vi "PDC.vi"() -> ()   [LabVIEW 2013]
uses:
  CTRLs/PMU_CMDs.ctl
panel:
  in  "data array [mag, phase (deg)]":cluster{"magnitude":dbl, "phase":dbl}[](array[cluster])=[{"magnitude"=10.0, "phase"=0.0}, {"magnitude"=10.0, "phase"=0.0}, {"magnitude"=10.0, "phase"=0.0}, {"magnitude"=10.0, "phase"=0.0}, {"magnitude"=10.0, "phase"=0.0}, {"magnitude"=10.0, "phase"=0.0}, {"magnitude"=10.0, "phase"=0.0}, {"magnitude"=10.0, "phase"=0.0}, {"magnitude"=10.0, "phase"=0.0}, {"magnitude"=10.0, "phase"=0.0}, {"magnitude"=10.0, "phase"=0.0}, {"magnitude"=10.0, "phase"=0.0}, {"magnitude"=10.0, "phase"=0.0}, {"magnitude"=10.0, "phase"=0.0}, {"magnitude"=10.0, "phase"=0.0}, {"magnitude"=10.0, "phase"=0.0}, {"magnitude"=10.0, "phase"=0.0}, {"magnitude"=10.0, "phase"=0.0}, {"magnitude"=10.0, "phase"=0.0}] {"phase" format="%0.2f"; "magnitude" format="%0.2f"}
  in  "Size":u16=4
  out "Freq":sgl[](array[numeric])
  out "path":path
  out "T button?":bool
  out "PMU1 CFG Packet":string[](array[string])
  out "PMU Row Number":i32
  out "UDP STRNG 2":string
  out "Date/Time 4":string
  out "Phasor Row Number":i32
  in  "Tab Control 2":T1(tab)
  out "MagnitudePMU":waveform(sgl)(graph)
  out "FrequencyPMU":waveform(sgl)(graph)
  out "PMUROCOF":waveform(sgl)(graph)
  out "PMUAnalogs":waveform(sgl)(graph)
  out "seconds":dbl
  out "Array 2":u16[][](array[numeric]) format="%b"
  out "Array":string[][](array[string])
  out "Analogs":string[][](array[string])
  out "Freq Floating?":bool[](array[boolean])
  out "Analog Floating?":bool[](array[boolean])
  out "Polar?":bool[](array[boolean])
  out "Transposed":string[][](array[string])
  out "Real":string[][](array[string])
  out "Imaginary":string[][](array[string])
  out "transposed array 5":sgl[][](array[numeric])
  out "transposed array 4":sgl[][](array[numeric])
  out "Phasors Floatingpoint?":bool[](array[boolean])
  out "Format":u16[](array[numeric]) format="%b"
  out "Digitals":u16[](array[numeric])
  out "Analog":u16[](array[numeric])
  out "Phasor":u16[](array[numeric])
  out "DGTL Packet":string[](array[string])
  out "ANG Packet":string[](array[string])
  out "DFREQ Packet":string[](array[string])
  out "FREQ Packet":string[](array[string])
  out "PZRs Packet":string[](array[string])
  out "UNITs 2":T2
  out "Date/Time 3":string
  out "PMU DATA Packet 2":string[](array[string])
  out "DATA FRAME 2":string
  out "error out 2":errorcluster
  out "UDP STRNG":string
  out "UNITs":T2
  out "Date/Time 2":string
  in  "Start Com Button":bool
  in  "User Configuration":T3(tab)
  in  "IP Address":string="127.0.0.1"
  in  "remote port":u16=4712
  in  "Device ID":u16
  in  "Unicast Address":string="127.0.0.1"
  in  "Local Port":u16=58431
  in  "TTL":u16=16
  in  "Send to Port":u16=58432
  out "Alert Incorrect \nNetwork Info":bool
  in  "Data Display":T4(tab)
  in  "PMU Phasors":i32(listbox)
  in  "PMU Analogs":i32(listbox)
  in  "PMU Digitals":i32(listbox)
  in  "dFreq":sgl[](array[numeric])
  in  "Frequency":sgl[](array[numeric])
  in  "Tab Control":T5(tab)
  in  "Complex Phasors":csg[][](array[numeric])
  in  "Magnitude":sgl[][](array[numeric])
  in  "Angle (Radians)":sgl[][](array[numeric])
  in  "Analog Values":sgl[][](array[numeric])
  out "Boolean array":bool[][](array[boolean])
  out "Magnitude":sgl[](array[numeric])
  out "Angle":sgl[](array[numeric])
  out "Complex Phasors":csg[](array[numeric])
  out "DFREQ Values":dbl[](array[numeric])
  out "FREQ Values":dbl[](array[numeric])
  out "Chosen Data 2":i32(listbox)
  out "DATA ONLINE":bool
  in  "Display Cluster Output":bool
  out "UDP String":string
  out "Freq >Threshold":bool
  out "Frequency Monitoring":waveform(sgl)[](graph)
  out "Freq < Threshold":bool
  out "Warning":string[](array[string])
  out "Phasor Plot":picture
  out "Available Phasors in the PMU/PDC Stream":string[](array[string])
  out "Phasor Magnitude":sgl[](array[numeric])
  out "Phasor Angle (Degrees)":sgl[](array[numeric])
  in  "Data Selector":T6(tab)
  out "No. of Digitals in this PMU":u8
  out "No. of Analogs in this PMU":u8
  out "No. of Phasors in this PMU":u8
  out "Freq/dFreq Format":string
  out "Analog Format":string
  out "Phasor Format":string
  out "Phasor Type":string
  out "DATA_RATE":u32
  in  "Names of PMUs":i32(listbox)
  out "Nominal_Frequency":string
  out "NUM_of_PMUs":u32
  in  "PMU Phasors List 2":i32(listbox)
  out "Phasor_Names":string[](array[string])
  in  "PMU Phasors List":i32(listbox)
  out "Phasors Index":u16[](array[numeric])
  out "PMU number in List":i32[](array[numeric])
  out "Phasor number in selected PMU":i32[](array[numeric])
  out "Time Quality":string[](array[string])
  out "STAT FIELD  WITH RESPEC TO PMU List":string[](array[string])
  out "PMUs List":i32(listbox)
  out "GPS Sync?":bool[](array[boolean])
  out "Status - PMU Sync with GPS":string[](array[string])
  out "Unlocked Time":string[](array[string])
  out "Config Change?":bool[](array[boolean])
  out "Change in Configuration":string[](array[string])
  out "PMUs List 2":i32(listbox)
  out "PMU DATA Packet":string[](array[string])
  out "Data size to read":u32
  out "Size of DATA Frame":u32
  out "CFG-2 Frame":string
  out "PMU1 CFG Packet":string[](array[string])
  out "Date/Time":string
  out "TIME_BASE":u32
  out "FRACSEC":u64
  out "SOC":u64
  out "IDCODE":u32
  out "FRAMSIZE":u32
  out "SYNC":u32
  out "Valid?!":bool
  out "CRC-Bytes":string
  out "DATA FRAME":string
  in  "Stop Button":bool
  out "COMMAND Frame":string
  out "bytes written":i32
  in  "DATA ON":bool
  in  "DATA OFF":bool
  out "length":i32
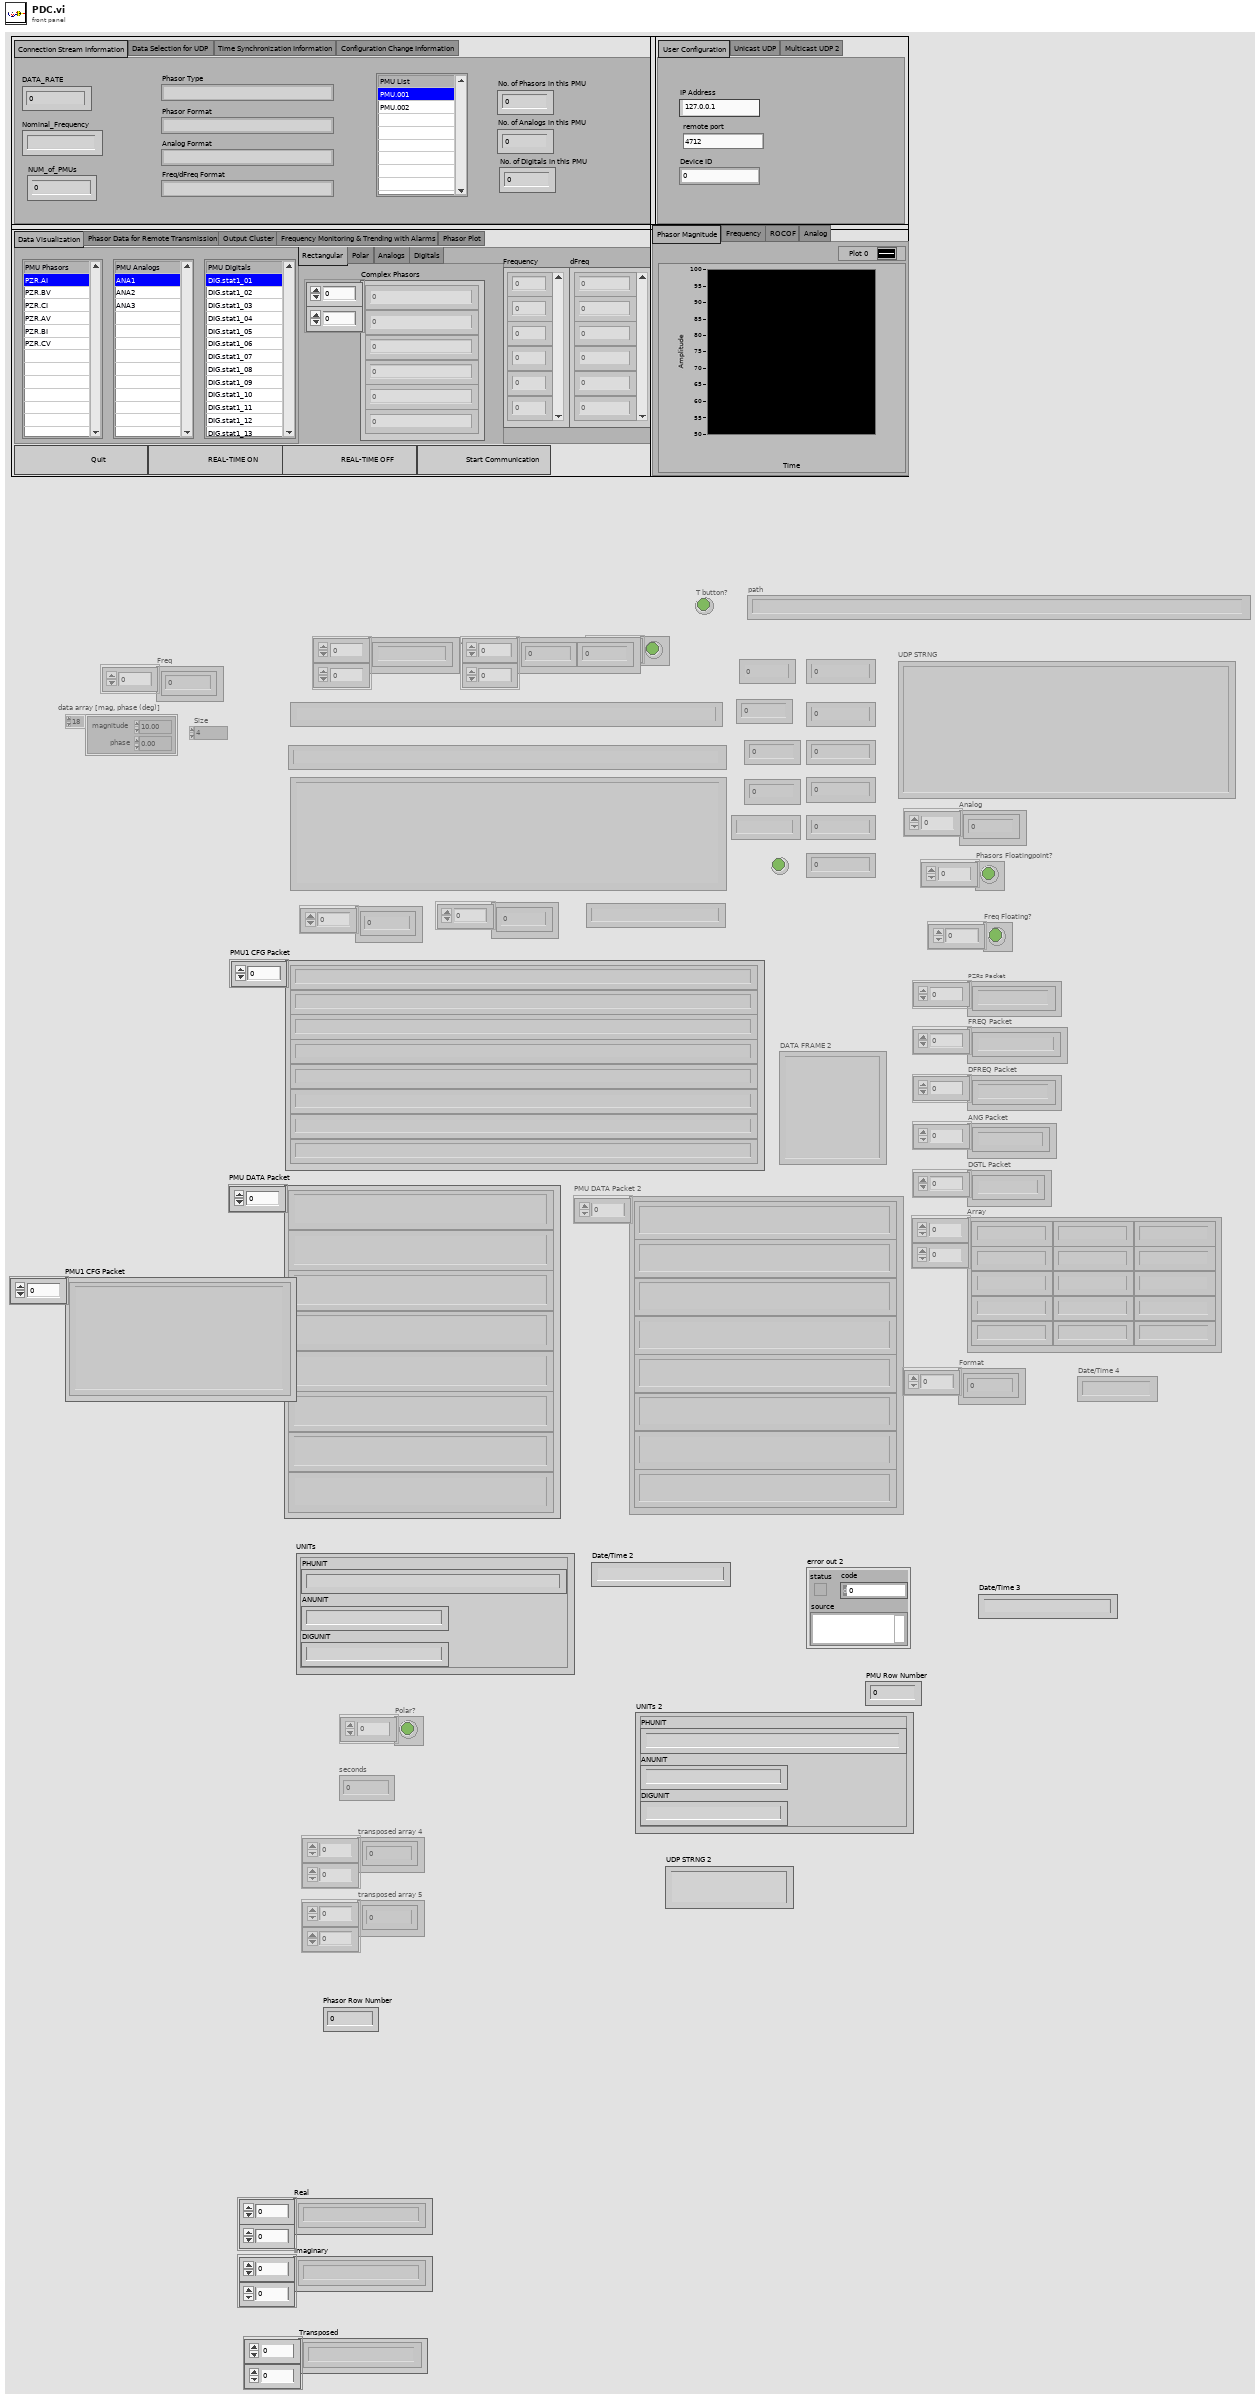
[diagram p1: front panel]
types:
  T1 = enum32{"Phasor Magnitude", "Frequency", "ROCOF", "Analog"}
  T2 = cluster{"PHUNIT":string, "ANUNIT":string, "DIGUNIT":string}
  T3 = enum32{"User Configuration", "Unicast UDP", "Multicast UDP 2"}
  T4 = enum32{"Data Visualization", "Phasor Data for Remote Transmission", "Output Cluster", "Frequency Monitoring & Trending with Alarms", "Phasor Plot"}
  T5 = enum32{"Rectangular", "Polar", "Analogs", "Digitals"}
  T6 = enum32{"Connection Stream Information", "Data Selection for UDP", "Time Synchronization Information", "Configuration Change Information"}
  T7 = cluster{"Date/Time":string, "DATA_DTLD":cluster{"PZRs Packet":string[], "FREQ Packet":string[], "DFREQ Packet":string[], "ANG Packet":string[], "DGTL Packet":string[]}}
  T8 = typedef "PMU_CMDs.ctl" = enum16{"dummy", "Turn off Transmission of Data Frame", "Turn on Transmission of Data Frame", "Send Header Frame", "Send CFG-1 Frame", "Send CFG-2 Frame", "Extended Frame"}
  T9 = cluster{"SYNC":u32, "FRAMSIZE":u32, "IDCODE":u32, "SOC":u64, "DATA_RATE":u32, "FRACSEC":u64, "TIME_BASE":u32, "NUM_PMU":u32}
  T10 = cluster{"PHASORS":cluster{"PZR 1":string, "PZR 2":string, "PZR 3":string, "PZR 4":string, "PZR 5":string, "PZR 6":string}, "NUMs":cluster{"PHNMR":u8, "ANNMR":u8, "DGNMR":u8}, "FORMAT":cluster{"PH_MAG_ANG":u16, "PH_FLOATING":u16, "AN_FLOATING":u16, "FREQ_DFREQ_FLOATING":u16}, "ANGs":cluster{"AN1":string, "AN2":string, "AN3":string}, "DIGs":cluster{"DIG 1":string, "DIG 2":string, "DIG 3":string, "DIG 4":string, "DIG 5":string, "DIG 6":string, "DIG 7":string, "DIG 8":string, "DIG 9":string, "DIG 10":string, "DIG 11":string, "DIG 12":string, "DIG 13":string, "DIG 14":string, "DIG 15":string, "DIG 16":string}, "IDCODE":u16, "Station Name":string, "UNITs":cluster{"PHUNIT":string, "ANUNIT":string, "DIGUNIT":string}, "FNOM":string, "CFGCNT":string}
  T11 = cluster{"PZRs Packet":string[], "FREQ Packet":string[], "DFREQ Packet":string[], "ANG Packet":string[], "DGTL Packet":string[]}
  T12 = typedef "LVDateTimeRec.ctl" = cluster{"fractional second":dbl, "second":i32, "minute":i32, "hour":i32, "day of month":i32, "month":i32, "year":i32, "day of week":i32, "day of year":i32, "DST":i32}
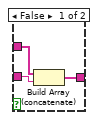
[diagram p4: hidden frame]
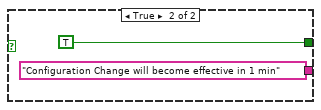
[diagram p5: hidden frame]
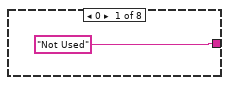
[diagram p6: hidden frame]
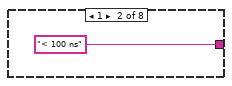
[diagram p7: hidden frame]
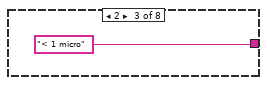
[diagram p8: hidden frame]
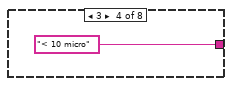
[diagram p9: hidden frame]
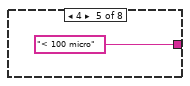
[diagram p10: hidden frame]
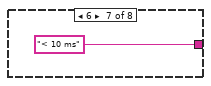
[diagram p11: hidden frame]
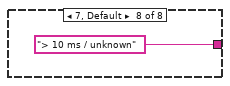
[diagram p12: hidden frame]
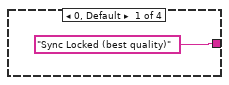
[diagram p13: hidden frame]
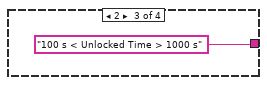
[diagram p14: hidden frame]
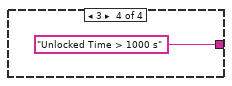
[diagram p15: hidden frame]
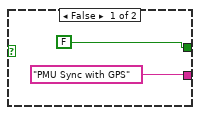
[diagram p16: hidden frame]
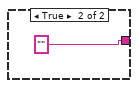
[diagram p17: hidden frame]
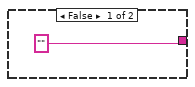
[diagram p18: hidden frame]
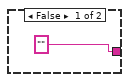
[diagram p19: hidden frame]
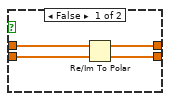
[diagram p20: hidden frame]
diagram:
  # "This file is part of BFE.\n\n    BFE is free software: you can redistribute it and/or modify\n    it under the terms of the GNU General Public License as published by\n    the Free Software Foundation, either version 3 of the License, or\n    (at your option) any later version.\n\n   BFE is distributed in the hope that it will be useful,\n    but WITHOUT ANY WARRANTY; without even the implied warranty of\n    MERCHANTABILITY or FITNESS FOR A PARTICULAR PURPOSE.  See the\n    GNU General Public License for more details.\n\n    You should have received a copy of the GNU General Public License\n    along with BFE.  If not, see <http://www.gnu.org/licenses/>."
  n1 = flat-sequence {
    tunnel: [w84] -> w64
    tunnel: [w83] -> w62
    frame #0 {
      w74 = "" ("Phasor Type")
      w73 = u8 0 ("No. of Phasors in this PMU")
      w72 = string[] [""] ("Phasor Name")
      # "License Prompt"
      # "Initializing all variables to their default values"
      n2 = Two Button Dialog(message="<BFE>  Copyright (C) <2016>  <Luigi Vanfretti, Muhammad Shoaib Almas, Maxime Baudette>\n    This program comes with ABSOLUTELY NO WARRANTY; for details click on \"show details\"'.\n    This is free software, and you are welcome to redistribute it\n    under certain conditions; click on `show details' for details.", 1:"Show Details" ("F button name (\"Cancel\")"), 2:"OK" ("T button name (\"OK\")")) -> (T button?=w67:bool)
      "T button?" <- w67
      n3 = Equal?(x=w67, y=FALSE) -> (x = y?=w65:bool)
      n4 = case shown="True" w65 {
        frame False {
        }
        frame True {
          n5 = Current VI's Path() -> (path=w79:path)
          "path" <- w79
          n6 = Strip Path(path=w79) -> (stripped path=w77:path)  [unwired: 1 out]
          n7 = Build Path(base path=w77, name or relative path="License") -> (appended path=w75:path)
          n8 = call <vilib>:"System Exec.vi"("working directory"=w75, "command line"="Notepad COPYING") -> ()  [unwired: 6 in, 4 out]
        }
      }
      n9 = property on="NUM_of_PMUs" class="DigNum (strict)"("Value"=w73) -> ()  [unwired: 2 in, 2 out]
      n10 = property on="DATA_RATE" class="DigNum (strict)"("Value"=w73) -> ()  [unwired: 2 in, 2 out]
      n11 = property on="No. of Phasors in this PMU" class="DigNum (strict)"("Value"=w73) -> ()  [unwired: 2 in, 2 out]
      n12 = property on="No. of Analogs in this PMU" class="DigNum (strict)"("Value"=w73) -> ()  [unwired: 2 in, 2 out]
      n13 = property on="No. of Digitals in this PMU" class="DigNum (strict)"("Value"=w73) -> ()  [unwired: 2 in, 2 out]
      n14 = property on="Analog Format" class="Str"("Value"=w74) -> ()  [unwired: 2 in, 2 out]
      n15 = property on="Phasor Type" class="Str"("Value"=w74) -> ()  [unwired: 2 in, 2 out]
      n16 = property on="Phasor Format" class="Str"("Value"=w74) -> ()  [unwired: 2 in, 2 out]
      n17 = property on="Freq/dFreq Format" class="Str"("Value"=w74) -> ()  [unwired: 2 in, 2 out]
      n18 = property on="Phasors Index" class="Arr (strict)"("Value"=u16[] [0, 0, 0, 0] ("Phasors Index")) -> ()  [unwired: 2 in, 2 out]
      n19 = property on="Nominal_Frequency" class="Str"("Value"=w74) -> ()  [unwired: 2 in, 2 out]
      n20 = property on="PMU Phasors List" class="LstBox (strict)"("Item Names"=w72) -> ()  [unwired: 2 in, 2 out]
      n21 = property on="PMU Analogs" class="LstBox (strict)"("Item Names"=w72) -> ()  [unwired: 2 in, 2 out]
      n22 = property on="PMU Phasors" class="LstBox (strict)"("Item Names"=w72) -> ()  [unwired: 2 in, 2 out]
      n23 = property on="PMU Digitals" class="LstBox (strict)"("Item Names"=w72) -> ()  [unwired: 2 in, 2 out]
      n24 = property on="Names of PMUs" class="LstBox (strict)"("Item Names"=w72) -> ()  [unwired: 2 in, 2 out]
      n25 = property on="Names of PMUs" class="LstBox (strict)"("Item Names"=w72) -> ()  [unwired: 2 in, 2 out]
      n26 = property on="Phasor_Names" class="Arr (strict)"("Value"=w72) -> ()  [unwired: 2 in, 2 out]
    }
    frame #1 {
      n27 = while {
        stop <- "Start Com Button" stop-if-true
      }
    }
    frame #2 {
      n28 = TCP Open Connection(address="IP Address", remote port or service name="remote port") -> (connection ID=w84:refnum<k5>, error out=w83:errorcluster)  [unwired: 3 in]
    }
  }
  n29 = flat-sequence {
    tunnel: w64 -> [w90]
    tunnel: w62 -> [w91]
    tunnel: [w89] -> w50
    tunnel: [w88] -> w49
    tunnel: ["Device ID"] -> w24
    tunnel: w50 -> [w95]
    tunnel: [w98] -> w48
    tunnel: w49 -> [w96]
    tunnel: [w97] -> w46
    tunnel: w24 -> [w92]
    tunnel: [w92] -> w23
    tunnel: w48 -> [w107]
    tunnel: [w108] -> w47
    tunnel: w46 -> [w106]
    tunnel: [w109] -> w45
    tunnel: [w100] -> w44
    tunnel: w23 -> [w99]
    tunnel: [w99] -> w22
    tunnel: w47 -> [w114]
    tunnel: [w114] -> w52
    tunnel: w45 -> [w113]
    tunnel: [w113] -> w51
    tunnel: w44 -> [w111]
    tunnel: [w111] -> w43
    tunnel: w22 -> [w110]
    tunnel: [w110] -> w21
    tunnel: w52 -> [w120]
    tunnel: [w119] -> w41
    tunnel: w51 -> [w118]
    tunnel: [w117] -> w40
    tunnel: w43 -> [w122]
    tunnel: [w122] -> w39
    tunnel: w21 -> [w115]
    tunnel: [w115] -> w20
    tunnel: w41 -> [w127]
    tunnel: w40 -> [w126]
    tunnel: [w129] -> w60
    tunnel: [w128] -> w59
    tunnel: w39 -> [w124]
    tunnel: [w124] -> w42
    tunnel: w20 -> [w123]
    tunnel: w60 -> [w141]
    tunnel: w59 -> [w140]
    tunnel: [w143] -> w58
    tunnel: [w142] -> w57
    tunnel: [w131] -> w56
    tunnel: w42 -> [w139]
    tunnel: w58 -> [w158]
    tunnel: w57 -> [w157]
    tunnel: w56 -> [w149]
    tunnel: [w158] -> w55
    tunnel: [w157] -> w54
    tunnel: [w149] -> w53
    tunnel: [w144] -> w38
    tunnel: w55 -> [w197]
    tunnel: w54 -> [w196]
    tunnel: w53 -> [w195]
    tunnel: w38 -> [w176]
    tunnel: [w197] -> w33
    tunnel: [w196] -> w32
    tunnel: [w172] -> w31
    tunnel: w33 -> [w218]
    tunnel: w32 -> [w217]
    tunnel: w31 -> [w216]
    tunnel: [w218] -> w28
    tunnel: [w217] -> w27
    tunnel: [w216] -> w26
    tunnel: [w230] -> w30
    tunnel: [w227] -> w61
    tunnel: [w225] -> w63
    tunnel: w28 -> [w226]
    tunnel: w27 -> [w228]
    tunnel: w26 -> [w230]
    frame #0 {
      n30 = call "CMD.vi"("PMU ID"="Device ID", "command"=PMU_CMDs."Turn off Transmission of Data Frame") -> ("CMD"=w87:string)  [unwired: 4 in, 1 out]
      n31 = TCP Write(connection ID=w90, data in=w87, error in (no error)=w91) -> (connection ID out=w89:refnum<k5>, error out=w88:errorcluster)  [unwired: 1 in, 1 out]
    }
    frame #1 {
      n32 = call "CMD.vi"("PMU ID"=w92, "command"=PMU_CMDs."Send CFG-2 Frame") -> ("CMD"=w93:string)  [unwired: 4 in, 1 out]
      n33 = TCP Write(connection ID=w95, data in=w93, error in (no error)=w96) -> (connection ID out=w98:refnum<k5>, error out=w97:errorcluster)  [unwired: 1 in, 1 out]
    }
    frame #2 {
      w103 = 2 ("offset (0)")
      n34 = TCP Read(connection ID=w107, bytes to read=4, error in (no error)=w106) -> (connection ID out=w108:refnum<k5>, data out=w104:string, error out=w109:errorcluster)  [unwired: 2 in]
      n35 = String Subset(string=w104, offset (0)=w103, length (rest)=w103) -> (substring=w102:string)
      n36 = Type Cast(type=u16 0 ("bytes to read"), x=w102) -> (*(type *) &x=w100:u16)
    }
    frame #3 {
      n37 = Wait (ms)(milliseconds to wait=u32 20) -> ()  [unwired: 1 out]
    }
    frame #4 {
      n38 = call "CMD.vi"("PMU ID"=w115, "command"=PMU_CMDs."Turn off Transmission of Data Frame") -> ("CMD"=w121:string)  [unwired: 4 in, 1 out]
      n39 = TCP Write(connection ID=w120, data in=w121, error in (no error)=w118) -> (connection ID out=w119:refnum<k5>, error out=w117:errorcluster)  [unwired: 1 in, 1 out]
    }
    frame #5 {
      n40 = call "CMD.vi"("PMU ID"=w123, "command"=PMU_CMDs."Send CFG-2 Frame") -> ("CMD"=w125:string)  [unwired: 4 in, 1 out]
      n41 = TCP Write(connection ID=w127, data in=w125, error in (no error)=w126) -> (connection ID out=w129:refnum<k5>, error out=w128:errorcluster)  [unwired: 1 in, 1 out]
    }
    frame #6 {
      w137 = 4 ("y")
      n42 = TCP Read(connection ID=w141, bytes to read=w139, error in (no error)=w140) -> (connection ID out=w143:refnum<k5>, data out=w132:string, error out=w142:errorcluster)  [unwired: 2 in]
      n43 = String Length(string=w132) -> (length=w138:i32)
      n44 = Subtract(x=w138, y=w137) -> (x-y=w133:i32)
      n45 = String Subset(string=w132, offset (0)=w133, length (rest)=w137) -> (substring=w136:string)
      n46 = String Subset(string=w132, offset (0)=0, length (rest)=w133) -> (substring=w135:string)
      n47 = Concatenate Strings(w136, w135) -> (w131:string)
      "CFG-2 Frame" <- w131
    }
    frame #7 {
      n48 = call "CHK_CRC.vi"("data in"=w149) -> ("Valid?!"=→"Valid?!":bool, "CRC-Bytes"=→"CRC-Bytes":string)
      n49 = call "SYS_INFO.vi"("CFG-2"=w149) -> ("output cluster"=w150:T9)
      n50 = Unbundle By Name(w150) -> ("SYNC"=→"SYNC":u32, "FRAMSIZE"=→"FRAMSIZE":u32, "IDCODE"=→"IDCODE":u32, "SOC"=w148:u64, "FRACSEC"=w146:u64, "TIME_BASE"=w145:u32, "NUM_PMU"=w144:u32, "DATA_RATE"=→"DATA_RATE":u32)
      "SOC" <- w148
      "FRACSEC" <- w146
      "TIME_BASE" <- w145
      "NUM_of_PMUs" <- w144
      n51 = call "UNIX-DATE_TIME.vi"("TIME_BASE"=w145, "FRACSEC"=w146, "SOC"=w148) -> ("Date/Time"=→"Date/Time":string)  [unwired: 1 out]
    }
    frame #8 {
      w192 = 4
      w174 = 2
      n52 = call "PMU_CFG-2_PACK.vi"("String"=w195) -> ("PMU1 CFG Packet"=w172:string[])
      "PMU1 CFG Packet" <- w172
      n53 = Index Array(array=w172, index=0) -> (element=w194:string)
      n54 = call "PMU_INFO.vi"("data in"=w194) -> ("RET_DATA"=w162:T10)
      n55 = Unbundle By Name(w162) -> ("FNOM"=w161:string)
      n56 = Type Cast(type=u16 2 ("length (rest)"), x=w161) -> (*(type *) &x=w160:u16)
      n57 = Unbundle By Name(w162) -> ("FORMAT.PH_MAG_ANG"=w168:u16, "FORMAT.PH_FLOATING"=w167:u16, "FORMAT.AN_FLOATING"=w166:u16, "FORMAT.FREQ_DFREQ_FLOATING"=w165:u16)
      n58 = case shown="1" w160 {
        tunnel: ["60 Hz Nominal" "50 Hz"] -> w159
        frame 0, Default {
        }
        frame 1 {
        }
      }
      "Nominal_Frequency" <- w159
      n59 = case shown="0, Default" w168 {
        tunnel: ["Rectangular Coordinates" "Polar Coordinates"] -> w164
        frame 0, Default {
        }
        frame 1 {
        }
      }
      "Phasor Type" <- w164
      n60 = case shown="0, Default" w167 {
        tunnel: ["16 bit integer" "32 bit floating point"] -> w171
        frame 0, Default {
        }
        frame 1 {
        }
      }
      "Phasor Format" <- w171
      n61 = case shown="0, Default" w166 {
        tunnel: ["16 bit integer" "32 bit floating point"] -> w170
        frame 0, Default {
        }
        frame 1 {
        }
      }
      "Analog Format" <- w170
      n62 = case shown="0, Default" w165 {
        tunnel: ["16 bit integer" "32 bit floating point"] -> w169
        frame 0, Default {
        }
        frame 1 {
        }
      }
      "Freq/dFreq Format" <- w169
      n63 = Unbundle By Name(w162) -> ("FORMAT.PH_FLOATING"=w185:u16, "FORMAT.AN_FLOATING"=w184:u16, "FORMAT.FREQ_DFREQ_FLOATING"=w186:u16, "NUMs.PHNMR"=w190:u8, "NUMs.ANNMR"=w182:u8, "NUMs.DGNMR"=w179:u8)  [unwired: 1 out]
      n64 = case shown="0, Default" w185 {
        tunnel: [4 8] -> w191
        frame 0, Default {
        }
        frame 1 {
          # "PH_FACTOR"
        }
      }
      n65 = case shown="0, Default" w184 {
        tunnel: [2 4] -> w183
        frame 0, Default {
        }
        frame 1 {
          # "PH_FACTOR"
        }
      }
      n66 = Multiply(x=w179, y=2) -> (x*y=w180:i32)
      n67 = case shown="1" w186 {
        tunnel: [2 4] -> w187
        frame 0, Default {
        }
        frame 1 {
          # "PH_FACTOR"
        }
      }
      n68 = Multiply(x=w191, y=w190) -> (x*y=w188:i32)
      n69 = Multiply(x=w182, y=w183) -> (x*y=w181:i32)
      n70 = Compound Arithmetic op=ADD(2, w188, w187, w187, w181, w180) -> (w177:i32)
      n71 = Multiply(x=w177, y=w176) -> (x*y=w175:u32)
      n72 = Compound Arithmetic op=ADD(w174, w174, w174, w192, w192, w175, w174) -> (→"Size of DATA Frame":u32)
    }
    frame #9 {
      n73 = property on="NUM_of_PMUs" class="DigNum (strict)"() -> ("Value"=w215:u32)  [unwired: 2 in, 2 out]
      n74 = for {
        N: w215 -> [_]
        tunnel: w216 -> [w222] mode=indexing
        tunnel: [w219] -> w214 mode=indexing
        n75 = String Subset(string=w222, offset (0)=0, length (rest)=16 ("length (rest)")) -> (substring=w219:string)
      }
      n76 = property on="PMU Phasors List 2" class="LstBox (strict)"("Item Names"=w214) -> ()  [unwired: 2 in, 2 out]
      n77 = property on="PMUs List 2" class="LstBox (strict)"("Item Names"=w214) -> ()  [unwired: 2 in, 2 out]
      n78 = property on="Names of PMUs" class="LstBox (strict)"("Item Names"=w214) -> ()  [unwired: 2 in, 2 out]
      n79 = property on="PMUs List" class="LstBox (strict)"("Item Names"=w214) -> ()  [unwired: 2 in, 2 out]
    }
    frame #10 {
      n80 = local read "Device ID"() -> (w223:u16)
      n81 = call "CMD.vi"("PMU ID"=w223, "command"=PMU_CMDs."Turn off Transmission of Data Frame") -> ("CMD"=w229:string)  [unwired: 4 in, 1 out]
      n82 = TCP Write(connection ID=w226, data in=w229, error in (no error)=w228) -> (connection ID out=w225:refnum<k5>, error out=w227:errorcluster)  [unwired: 1 in, 1 out]
    }
  }
  n83 = flat-sequence {
    tunnel: ["Send to Port"] -> w10
    tunnel: [w249] -> w7
    tunnel: [w248] -> w9
    tunnel: [w236] -> w8
    frame #0 {
      # "Local Port number on this\nmachine"
      # "Time To Live edit\nbox usually 16 is the\nbest to send over networks"
      # "IP Address of destination\nsite over UDP."
      # "send the phasor\nparameters to this\nUDP port edit box"
      # "Open a UDP port for Multicast Write Only."
      n84 = String To IP(1:"0.0.0.0" ("x")) -> (0:w245:u32)
      n85 = String To IP(1:"223.255.255.255" ("x")) -> (0:w244:u32)
      n86 = String To IP(1:"Unicast Address") -> (0:w236:u32)
      n87 = String To IP(1:"240.255.255.255" ("x")) -> (0:w240:u32)
      n88 = String To IP(1:"247.255.255.255" ("x")) -> (0:w239:u32)
      n89 = Greater Or Equal?(x=w236, y=w245) -> (x >= y?=w247:bool)
      n90 = Less Or Equal?(x=w236, y=w244) -> (x <= y?=w246:bool)
      n91 = Greater Or Equal?(x=w236, y=w240) -> (x >= y?=w235:bool)
      n92 = Less Or Equal?(x=w236, y=w239) -> (x <= y?=w234:bool)
      n93 = Not And(1:w246, 2:w247) -> (0:w233:bool)
      n94 = Not And(1:w234, 2:w235) -> (0:w232:bool)
      n95 = And(x=w233, y=w232) -> (x .and. y?=w231:bool)
      "Alert Incorrect \nNetwork Info" <- w231
      n96 = case shown="True" w231 {
        frame False {
        }
        frame True {
          n97 = call "Display Message to User"() -> ()  [unwired: 10 in, 2 out]
        }
      }
      n98 = UDP Open(9:"TTL", 11:"Local Port") -> (port=w249:refnum<k16>, 0:w248:errorcluster)  [unwired: 3 in, 1 out]
      "error out 2" <- w248
    }
  }
  n99 = Obtain Queue(name (unnamed)="DISP DATA", element data type=T7 {"Date/Time"="26-12-2013, 0:30:36 0.866666", "DATA_DTLD"={"PZRs Packet"=[], "FREQ Packet"=[], "DFREQ Packet"=[], "ANG Packet"=[], "DGTL Packet"=[]}}) -> (queue out=w4:refnum<queue>, error out=w3:errorcluster)  [unwired: 3 in, 1 out]
  n100 = Obtain Queue(name (unnamed)="DATA FRAME", element data type=cluster{"DATA Type":string, "CFG Type":string[]} {"DATA Type"="", "CFG Type"=["PMU.001\u0000\u0000\u0000\u0000\u0000\u0000\u0000\u0000\u0000\u0000\u0001\u0000\u000f\u0000\u0006\u0000\u0003\u0000\u0001PZR.AI          PZR.BV          PZR.CI          PZR.AV          PZR.BI          PZR.CV          ANA1            ANA2            ANA3            DIG.stat1_01    DIG.stat1_02    DIG.stat1_03    DIG.stat1_04    DIG.stat1_05    DIG.stat1_06    DIG.stat1_07    DIG.stat1_08    DIG.stat1_09    DIG.stat1_10    DIG.stat1_11    DIG.stat1_12    DIG.stat1_13    DIG.stat1_14    DIG.stat1_15    DIG.stat1_16    \u0001\u0000\u0000\u0000\u0000\u0000\u0000\u0000\u0001\u0000\u0000\u0000\u0000\u0000\u0000\u0000\u0001\u0000\u0000\u0000\u0000\u0000\u0000\u0000\u0000\u0000\u0000\u0000\u0000\u0000\u0000\u0000\u0000\u0000\u0000\u0000ÿÿ\u0000\u0000\u0000\u0000\u0000\u0000", "PMU.002\u0000\u0000\u0000\u0000\u0000\u0000\u0000\u0000\u0000\u0000\u0002\u0000\u000f\u0000\u0006\u0000\u0003\u0000\u0001PZR.AI          PZR.BV          PZR.CI          PZR.AV          PZR.BI          PZR.CV          ANA1            ANA2            ANA3            DIG.stat1_01    DIG.stat1_02    DIG.stat1_03    DIG.stat1_04    DIG.stat1_05    DIG.stat1_06    DIG.stat1_07    DIG.stat1_08    DIG.stat1_09    DIG.stat1_10    DIG.stat1_11    DIG.stat1_12    DIG.stat1_13    DIG.stat1_14    DIG.stat1_15    DIG.stat1_16    \u0001\u0000\u0000\u0000\u0000\u0000\u0000\u0000\u0001\u0000\u0000\u0000\u0000\u0000\u0000\u0000\u0001\u0000\u0000\u0000\u0000\u0000\u0000\u0000\u0000\u0000\u0000\u0000\u0000\u0000\u0000\u0000\u0000\u0000\u0000\u0000ÿÿ\u0000\u0000\u0000\u0000\u0000\u0000", "PMU.003\u0000\u0000\u0000\u0000\u0000\u0000\u0000\u0000\u0000\u0000\u0003\u0000\u000f\u0000\u0006\u0000\u0003\u0000\u0001PZR.AI          PZR.BV          PZR.CI          PZR.AV          PZR.BI          PZR.CV          ANA1            ANA2            ANA3            DIG.stat1_01    DIG.stat1_02    DIG.stat1_03    DIG.stat1_04    DIG.stat1_05    DIG.stat1_06    DIG.stat1_07    DIG.stat1_08    DIG.stat1_09    DIG.stat1_10    DIG.stat1_11    DIG.stat1_12    DIG.stat1_13    DIG.stat1_14    DIG.stat1_15    DIG.stat1_16    \u0001\u0000\u0000\u0000\u0000\u0000\u0000\u0000\u0001\u0000\u0000\u0000\u0000\u0000\u0000\u0000\u0001\u0000\u0000\u0000\u0000\u0000\u0000\u0000\u0000\u0000\u0000\u0000\u0000\u0000\u0000\u0000\u0000\u0000\u0000\u0000ÿÿ\u0000\u0000\u0000\u0000\u0000\u0000", "PMU.004\u0000\u0000\u0000\u0000\u0000\u0000\u0000\u0000\u0000\u0000\u0004\u0000\u000f\u0000\u0006\u0000\u0003\u0000\u0001PZR.AI          PZR.BV          PZR.CI          PZR.AV          PZR.BI          PZR.CV          ANA1            ANA2            ANA3            DIG.stat1_01    DIG.stat1_02    DIG.stat1_03    DIG.stat1_04    DIG.stat1_05    DIG.stat1_06    DIG.stat1_07    DIG.stat1_08    DIG.stat1_09    DIG.stat1_10    DIG.stat1_11    DIG.stat1_12    DIG.stat1_13    DIG.stat1_14    DIG.stat1_15    DIG.stat1_16    \u0001\u0000\u0000\u0000\u0000\u0000\u0000\u0000\u0001\u0000\u0000\u0000\u0000\u0000\u0000\u0000\u0001\u0000\u0000\u0000\u0000\u0000\u0000\u0000\u0000\u0000\u0000\u0000\u0000\u0000\u0000\u0000\u0000\u0000\u0000\u0000ÿÿ\u0000\u0000\u0000\u0000\u0000\u0000", "PMU.005\u0000\u0000\u0000\u0000\u0000\u0000\u0000\u0000\u0000\u0000\u0005\u0000\u000f\u0000\u0006\u0000\u0003\u0000\u0001PZR.AI          PZR.BV          PZR.CI          PZR.AV          PZR.BI          PZR.CV          ANA1            ANA2            ANA3            DIG.stat1_01    DIG.stat1_02    DIG.stat1_03    DIG.stat1_04    DIG.stat1_05    DIG.stat1_06    DIG.stat1_07    DIG.stat1_08    DIG.stat1_09    DIG.stat1_10    DIG.stat1_11    DIG.stat1_12    DIG.stat1_13    DIG.stat1_14    DIG.stat1_15    DIG.stat1_16    \u0001\u0000\u0000\u0000\u0000\u0000\u0000\u0000\u0001\u0000\u0000\u0000\u0000\u0000\u0000\u0000\u0001\u0000\u0000\u0000\u0000\u0000\u0000\u0000\u0000\u0000\u0000\u0000\u0000\u0000\u0000\u0000\u0000\u0000\u0000\u0000ÿÿ\u0000\u0000\u0000\u0000\u0000\u0000", "PMU.006\u0000\u0000\u0000\u0000\u0000\u0000\u0000\u0000\u0000\u0000\u0006\u0000\u000f\u0000\u0006\u0000\u0003\u0000\u0001PZR.AI          PZR.BV          PZR.CI          PZR.AV          PZR.BI          PZR.CV          ANA1            ANA2            ANA3            DIG.stat1_01    DIG.stat1_02    DIG.stat1_03    DIG.stat1_04    DIG.stat1_05    DIG.stat1_06    DIG.stat1_07    DIG.stat1_08    DIG.stat1_09    DIG.stat1_10    DIG.stat1_11    DIG.stat1_12    DIG.stat1_13    DIG.stat1_14    DIG.stat1_15    DIG.stat1_16    \u0001\u0000\u0000\u0000\u0000\u0000\u0000\u0000\u0001\u0000\u0000\u0000\u0000\u0000\u0000\u0000\u0001\u0000\u0000\u0000\u0000\u0000\u0000\u0000\u0000\u0000\u0000\u0000\u0000\u0000\u0000\u0000\u0000\u0000\u0000\u0000ÿÿ\u0000\u0000\u0000\u0000\u0000\u0000", "PMU.007\u0000\u0000\u0000\u0000\u0000\u0000\u0000\u0000\u0000\u0000\u0007\u0000\u000f\u0000\u0006\u0000\u0003\u0000\u0001PZR.AI          PZR.BV          PZR.CI          PZR.AV          PZR.BI          PZR.CV          ANA1            ANA2            ANA3            DIG.stat1_01    DIG.stat1_02    DIG.stat1_03    DIG.stat1_04    DIG.stat1_05    DIG.stat1_06    DIG.stat1_07    DIG.stat1_08    DIG.stat1_09    DIG.stat1_10    DIG.stat1_11    DIG.stat1_12    DIG.stat1_13    DIG.stat1_14    DIG.stat1_15    DIG.stat1_16    \u0001\u0000\u0000\u0000\u0000\u0000\u0000\u0000\u0001\u0000\u0000\u0000\u0000\u0000\u0000\u0000\u0001\u0000\u0000\u0000\u0000\u0000\u0000\u0000\u0000\u0000\u0000\u0000\u0000\u0000\u0000\u0000\u0000\u0000\u0000\u0000ÿÿ\u0000\u0000\u0000\u0000\u0000\u0000", "PMU.008\u0000\u0000\u0000\u0000\u0000\u0000\u0000\u0000\u0000\u0000\b\u0000\u000f\u0000\u0006\u0000\u0003\u0000\u0001PZR.AI          PZR.BV          PZR.CI          PZR.AV          PZR.BI          PZR.CV          ANA1            ANA2            ANA3            DIG.stat1_01    DIG.stat1_02    DIG.stat1_03    DIG.stat1_04    DIG.stat1_05    DIG.stat1_06    DIG.stat1_07    DIG.stat1_08    DIG.stat1_09    DIG.stat1_10    DIG.stat1_11    DIG.stat1_12    DIG.stat1_13    DIG.stat1_14    DIG.stat1_15    DIG.stat1_16    \u0001\u0000\u0000\u0000\u0000\u0000\u0000\u0000\u0001\u0000\u0000\u0000\u0000\u0000\u0000\u0000\u0001\u0000\u0000\u0000\u0000\u0000\u0000\u0000\u0000\u0000\u0000\u0000\u0000\u0000\u0000\u0000\u0000\u0000\u0000\u0000ÿÿ\u0000\u0000\u0000\u0000\u0000\u0000", "PMU.009\u0000\u0000\u0000\u0000\u0000\u0000\u0000\u0000\u0000\u0000\t\u0000\u000f\u0000\u0006\u0000\u0003\u0000\u0001PZR.AI          PZR.BV          PZR.CI          PZR.AV          PZR.BI          PZR.CV          ANA1            ANA2            ANA3            DIG.stat1_01    DIG.stat1_02    DIG.stat1_03    DIG.stat1_04    DIG.stat1_05    DIG.stat1_06    DIG.stat1_07    DIG.stat1_08    DIG.stat1_09    DIG.stat1_10    DIG.stat1_11    DIG.stat1_12    DIG.stat1_13    DIG.stat1_14    DIG.stat1_15    DIG.stat1_16    \u0001\u0000\u0000\u0000\u0000\u0000\u0000\u0000\u0001\u0000\u0000\u0000\u0000\u0000\u0000\u0000\u0001\u0000\u0000\u0000\u0000\u0000\u0000\u0000\u0000\u0000\u0000\u0000\u0000\u0000\u0000\u0000\u0000\u0000\u0000\u0000ÿÿ\u0000\u0000\u0000\u0000\u0000\u0000", "PMU.010\u0000\u0000\u0000\u0000\u0000\u0000\u0000\u0000\u0000\u0000\n\u0000\u000f\u0000\u0006\u0000\u0003\u0000\u0001PZR.AI          PZR.BV          PZR.CI          PZR.AV          PZR.BI          PZR.CV          ANA1            ANA2            ANA3            DIG.stat1_01    DIG.stat1_02    DIG.stat1_03    DIG.stat1_04    DIG.stat1_05    DIG.stat1_06    DIG.stat1_07    DIG.stat1_08    DIG.stat1_09    DIG.stat1_10    DIG.stat1_11    DIG.stat1_12    DIG.stat1_13    DIG.stat1_14    DIG.stat1_15    DIG.stat1_16    \u0001\u0000\u0000\u0000\u0000\u0000\u0000\u0000\u0001\u0000\u0000\u0000\u0000\u0000\u0000\u0000\u0001\u0000\u0000\u0000\u0000\u0000\u0000\u0000\u0000\u0000\u0000\u0000\u0000\u0000\u0000\u0000\u0000\u0000\u0000\u0000ÿÿ\u0000\u0000\u0000\u0000\u0000\u0000", "PMU.011\u0000\u0000\u0000\u0000\u0000\u0000\u0000\u0000\u0000\u0000\u000b\u0000\u000f\u0000\u0006\u0000\u0003\u0000\u0001PZR.AI          PZR.BV          PZR.CI          PZR.AV          PZR.BI          PZR.CV          ANA1            ANA2            ANA3            DIG.stat1_01    DIG.stat1_02    DIG.stat1_03    DIG.stat1_04    DIG.stat1_05    DIG.stat1_06    DIG.stat1_07    DIG.stat1_08    DIG.stat1_09    DIG.stat1_10    DIG.stat1_11    DIG.stat1_12    DIG.stat1_13    DIG.stat1_14    DIG.stat1_15    DIG.stat1_16    \u0001\u0000\u0000\u0000\u0000\u0000\u0000\u0000\u0001\u0000\u0000\u0000\u0000\u0000\u0000\u0000\u0001\u0000\u0000\u0000\u0000\u0000\u0000\u0000\u0000\u0000\u0000\u0000\u0000\u0000\u0000\u0000\u0000\u0000\u0000\u0000ÿÿ\u0000\u0000\u0000\u0000\u0000\u0000", "PMU.012\u0000\u0000\u0000\u0000\u0000\u0000\u0000\u0000\u0000\u0000\f\u0000\u000f\u0000\u0006\u0000\u0003\u0000\u0001PZR.AI          PZR.BV          PZR.CI          PZR.AV          PZR.BI          PZR.CV          ANA1            ANA2            ANA3            DIG.stat1_01    DIG.stat1_02    DIG.stat1_03    DIG.stat1_04    DIG.stat1_05    DIG.stat1_06    DIG.stat1_07    DIG.stat1_08    DIG.stat1_09    DIG.stat1_10    DIG.stat1_11    DIG.stat1_12    DIG.stat1_13    DIG.stat1_14    DIG.stat1_15    DIG.stat1_16    \u0001\u0000\u0000\u0000\u0000\u0000\u0000\u0000\u0001\u0000\u0000\u0000\u0000\u0000\u0000\u0000\u0001\u0000\u0000\u0000\u0000\u0000\u0000\u0000\u0000\u0000\u0000\u0000\u0000\u0000\u0000\u0000\u0000\u0000\u0000\u0000ÿÿ\u0000\u0000\u0000\u0000\u0000\u0000", "PMU.013\u0000\u0000\u0000\u0000\u0000\u0000\u0000\u0000\u0000\u0000\r\u0000\u000f\u0000\u0006\u0000\u0003\u0000\u0001PZR.AI          PZR.BV          PZR.CI          PZR.AV          PZR.BI          PZR.CV          ANA1            ANA2            ANA3            DIG.stat1_01    DIG.stat1_02    DIG.stat1_03    DIG.stat1_04    DIG.stat1_05    DIG.stat1_06    DIG.stat1_07    DIG.stat1_08    DIG.stat1_09    DIG.stat1_10    DIG.stat1_11    DIG.stat1_12    DIG.stat1_13    DIG.stat1_14    DIG.stat1_15    DIG.stat1_16    \u0001\u0000\u0000\u0000\u0000\u0000\u0000\u0000\u0001\u0000\u0000\u0000\u0000\u0000\u0000\u0000\u0001\u0000\u0000\u0000\u0000\u0000\u0000\u0000\u0000\u0000\u0000\u0000\u0000\u0000\u0000\u0000\u0000\u0000\u0000\u0000ÿÿ\u0000\u0000\u0000\u0000\u0000\u0000", "PMU.014\u0000\u0000\u0000\u0000\u0000\u0000\u0000\u0000\u0000\u0000\u000e\u0000\u000f\u0000\u0006\u0000\u0003\u0000\u0001PZR.AI          PZR.BV          PZR.CI          PZR.AV          PZR.BI          PZR.CV          ANA1            ANA2            ANA3            DIG.stat1_01    DIG.stat1_02    DIG.stat1_03    DIG.stat1_04    DIG.stat1_05    DIG.stat1_06    DIG.stat1_07    DIG.stat1_08    DIG.stat1_09    DIG.stat1_10    DIG.stat1_11    DIG.stat1_12    DIG.stat1_13    DIG.stat1_14    DIG.stat1_15    DIG.stat1_16    \u0001\u0000\u0000\u0000\u0000\u0000\u0000\u0000\u0001\u0000\u0000\u0000\u0000\u0000\u0000\u0000\u0001\u0000\u0000\u0000\u0000\u0000\u0000\u0000\u0000\u0000\u0000\u0000\u0000\u0000\u0000\u0000\u0000\u0000\u0000\u0000ÿÿ\u0000\u0000\u0000\u0000\u0000\u0000", "PMU.015\u0000\u0000\u0000\u0000\u0000\u0000\u0000\u0000\u0000\u0000\u000f\u0000\u000f\u0000\u0006\u0000\u0003\u0000\u0001PZR.AI          PZR.BV          PZR.CI          PZR.AV          PZR.BI          PZR.CV          ANA1            ANA2            ANA3            DIG.stat1_01    DIG.stat1_02    DIG.stat1_03    DIG.stat1_04    DIG.stat1_05    DIG.stat1_06    DIG.stat1_07    DIG.stat1_08    DIG.stat1_09    DIG.stat1_10    DIG.stat1_11    DIG.stat1_12    DIG.stat1_13    DIG.stat1_14    DIG.stat1_15    DIG.stat1_16    \u0001\u0000\u0000\u0000\u0000\u0000\u0000\u0000\u0001\u0000\u0000\u0000\u0000\u0000\u0000\u0000\u0001\u0000\u0000\u0000\u0000\u0000\u0000\u0000\u0000\u0000\u0000\u0000\u0000\u0000\u0000\u0000\u0000\u0000\u0000\u0000ÿÿ\u0000\u0000\u0000\u0000\u0000\u0000", "PMU.016\u0000\u0000\u0000\u0000\u0000\u0000\u0000\u0000\u0000\u0000\u0010\u0000\u000f\u0000\u0006\u0000\u0003\u0000\u0001PZR.AI          PZR.BV          PZR.CI          PZR.AV          PZR.BI          PZR.CV          ANA1            ANA2            ANA3            DIG.stat1_01    DIG.stat1_02    DIG.stat1_03    DIG.stat1_04    DIG.stat1_05    DIG.stat1_06    DIG.stat1_07    DIG.stat1_08    DIG.stat1_09    DIG.stat1_10    DIG.stat1_11    DIG.stat1_12    DIG.stat1_13    DIG.stat1_14    DIG.stat1_15    DIG.stat1_16    \u0001\u0000\u0000\u0000\u0000\u0000\u0000\u0000\u0001\u0000\u0000\u0000\u0000\u0000\u0000\u0000\u0001\u0000\u0000\u0000\u0000\u0000\u0000\u0000\u0000\u0000\u0000\u0000\u0000\u0000\u0000\u0000\u0000\u0000\u0000\u0000ÿÿ\u0000\u0000\u0000\u0000\u0000\u0000", "PMU.017\u0000\u0000\u0000\u0000\u0000\u0000\u0000\u0000\u0000\u0000\u0011\u0000\u000f\u0000\u0006\u0000\u0003\u0000\u0001PZR.AI          PZR.BV          PZR.CI          PZR.AV          PZR.BI          PZR.CV          ANA1            ANA2            ANA3            DIG.stat1_01    DIG.stat1_02    DIG.stat1_03    DIG.stat1_04    DIG.stat1_05    DIG.stat1_06    DIG.stat1_07    DIG.stat1_08    DIG.stat1_09    DIG.stat1_10    DIG.stat1_11    DIG.stat1_12    DIG.stat1_13    DIG.stat1_14    DIG.stat1_15    DIG.stat1_16    \u0001\u0000\u0000\u0000\u0000\u0000\u0000\u0000\u0001\u0000\u0000\u0000\u0000\u0000\u0000\u0000\u0001\u0000\u0000\u0000\u0000\u0000\u0000\u0000\u0000\u0000\u0000\u0000\u0000\u0000\u0000\u0000\u0000\u0000\u0000\u0000ÿÿ\u0000\u0000\u0000\u0000\u0000\u0000", "PMU.018\u0000\u0000\u0000\u0000\u0000\u0000\u0000\u0000\u0000\u0000\u0012\u0000\u000f\u0000\u0006\u0000\u0003\u0000\u0001PZR.AI          PZR.BV          PZR.CI          PZR.AV          PZR.BI          PZR.CV          ANA1            ANA2            ANA3            DIG.stat1_01    DIG.stat1_02    DIG.stat1_03    DIG.stat1_04    DIG.stat1_05    DIG.stat1_06    DIG.stat1_07    DIG.stat1_08    DIG.stat1_09    DIG.stat1_10    DIG.stat1_11    DIG.stat1_12    DIG.stat1_13    DIG.stat1_14    DIG.stat1_15    DIG.stat1_16    \u0001\u0000\u0000\u0000\u0000\u0000\u0000\u0000\u0001\u0000\u0000\u0000\u0000\u0000\u0000\u0000\u0001\u0000\u0000\u0000\u0000\u0000\u0000\u0000\u0000\u0000\u0000\u0000\u0000\u0000\u0000\u0000\u0000\u0000\u0000\u0000ÿÿ\u0000\u0000\u0000\u0000\u0000\u0000", "PMU.019\u0000\u0000\u0000\u0000\u0000\u0000\u0000\u0000\u0000\u0000\u0013\u0000\u000f\u0000\u0006\u0000\u0003\u0000\u0001PZR.AI          PZR.BV          PZR.CI          PZR.AV          PZR.BI          PZR.CV          ANA1            ANA2            ANA3            DIG.stat1_01    DIG.stat1_02    DIG.stat1_03    DIG.stat1_04    DIG.stat1_05    DIG.stat1_06    DIG.stat1_07    DIG.stat1_08    DIG.stat1_09    DIG.stat1_10    DIG.stat1_11    DIG.stat1_12    DIG.stat1_13    DIG.stat1_14    DIG.stat1_15    DIG.stat1_16    \u0001\u0000\u0000\u0000\u0000\u0000\u0000\u0000\u0001\u0000\u0000\u0000\u0000\u0000\u0000\u0000\u0001\u0000\u0000\u0000\u0000\u0000\u0000\u0000\u0000\u0000\u0000\u0000\u0000\u0000\u0000\u0000\u0000\u0000\u0000\u0000ÿÿ\u0000\u0000\u0000\u0000\u0000\u0000", "PMU.020\u0000\u0000\u0000\u0000\u0000\u0000\u0000\u0000\u0000\u0000\u0014\u0000\u000f\u0000\u0006\u0000\u0003\u0000\u0001PZR.AI          PZR.BV          PZR.CI          PZR.AV          PZR.BI          PZR.CV          ANA1            ANA2            ANA3            DIG.stat1_01    DIG.stat1_02    DIG.stat1_03    DIG.stat1_04    DIG.stat1_05    DIG.stat1_06    DIG.stat1_07    DIG.stat1_08    DIG.stat1_09    DIG.stat1_10    DIG.stat1_11    DIG.stat1_12    DIG.stat1_13    DIG.stat1_14    DIG.stat1_15    DIG.stat1_16    \u0001\u0000\u0000\u0000\u0000\u0000\u0000\u0000\u0001\u0000\u0000\u0000\u0000\u0000\u0000\u0000\u0001\u0000\u0000\u0000\u0000\u0000\u0000\u0000\u0000\u0000\u0000\u0000\u0000\u0000\u0000\u0000\u0000\u0000\u0000\u0000ÿÿ\u0000\u0000\u0000\u0000\u0000\u0000", "PMU.021\u0000\u0000\u0000\u0000\u0000\u0000\u0000\u0000\u0000\u0000\u0015\u0000\u000f\u0000\u0006\u0000\u0003\u0000\u0001PZR.AI          PZR.BV          PZR.CI          PZR.AV          PZR.BI          PZR.CV          ANA1            ANA2            ANA3            DIG.stat1_01    DIG.stat1_02    DIG.stat1_03    DIG.stat1_04    DIG.stat1_05    DIG.stat1_06    DIG.stat1_07    DIG.stat1_08    DIG.stat1_09    DIG.stat1_10    DIG.stat1_11    DIG.stat1_12    DIG.stat1_13    DIG.stat1_14    DIG.stat1_15    DIG.stat1_16    \u0001\u0000\u0000\u0000\u0000\u0000\u0000\u0000\u0001\u0000\u0000\u0000\u0000\u0000\u0000\u0000\u0001\u0000\u0000\u0000\u0000\u0000\u0000\u0000\u0000\u0000\u0000\u0000\u0000\u0000\u0000\u0000\u0000\u0000\u0000\u0000ÿÿ\u0000\u0000\u0000\u0000\u0000\u0000", "PMU.022\u0000\u0000\u0000\u0000\u0000\u0000\u0000\u0000\u0000\u0000\u0016\u0000\u000f\u0000\u0006\u0000\u0003\u0000\u0001PZR.AI          PZR.BV          PZR.CI          PZR.AV          PZR.BI          PZR.CV          ANA1            ANA2            ANA3            DIG.stat1_01    DIG.stat1_02    DIG.stat1_03    DIG.stat1_04    DIG.stat1_05    DIG.stat1_06    DIG.stat1_07    DIG.stat1_08    DIG.stat1_09    DIG.stat1_10    DIG.stat1_11    DIG.stat1_12    DIG.stat1_13    DIG.stat1_14    DIG.stat1_15    DIG.stat1_16    \u0001\u0000\u0000\u0000\u0000\u0000\u0000\u0000\u0001\u0000\u0000\u0000\u0000\u0000\u0000\u0000\u0001\u0000\u0000\u0000\u0000\u0000\u0000\u0000\u0000\u0000\u0000\u0000\u0000\u0000\u0000\u0000\u0000\u0000\u0000\u0000ÿÿ\u0000\u0000\u0000\u0000\u0000\u0000", "PMU.023\u0000\u0000\u0000\u0000\u0000\u0000\u0000\u0000\u0000\u0000\u0017\u0000\u000f\u0000\u0006\u0000\u0003\u0000\u0001PZR.AI          PZR.BV          PZR.CI          PZR.AV          PZR.BI          PZR.CV          ANA1            ANA2            ANA3            DIG.stat1_01    DIG.stat1_02    DIG.stat1_03    DIG.stat1_04    DIG.stat1_05    DIG.stat1_06    DIG.stat1_07    DIG.stat1_08    DIG.stat1_09    DIG.stat1_10    DIG.stat1_11    DIG.stat1_12    DIG.stat1_13    DIG.stat1_14    DIG.stat1_15    DIG.stat1_16    \u0001\u0000\u0000\u0000\u0000\u0000\u0000\u0000\u0001\u0000\u0000\u0000\u0000\u0000\u0000\u0000\u0001\u0000\u0000\u0000\u0000\u0000\u0000\u0000\u0000\u0000\u0000\u0000\u0000\u0000\u0000\u0000\u0000\u0000\u0000\u0000ÿÿ\u0000\u0000\u0000\u0000\u0000\u0000", "PMU.024\u0000\u0000\u0000\u0000\u0000\u0000\u0000\u0000\u0000\u0000\u0018\u0000\u000f\u0000\u0006\u0000\u0003\u0000\u0001PZR.AI          PZR.BV          PZR.CI          PZR.AV          PZR.BI          PZR.CV          ANA1            ANA2            ANA3            DIG.stat1_01    DIG.stat1_02    DIG.stat1_03    DIG.stat1_04    DIG.stat1_05    DIG.stat1_06    DIG.stat1_07    DIG.stat1_08    DIG.stat1_09    DIG.stat1_10    DIG.stat1_11    DIG.stat1_12    DIG.stat1_13    DIG.stat1_14    DIG.stat1_15    DIG.stat1_16    \u0001\u0000\u0000\u0000\u0000\u0000\u0000\u0000\u0001\u0000\u0000\u0000\u0000\u0000\u0000\u0000\u0001\u0000\u0000\u0000\u0000\u0000\u0000\u0000\u0000\u0000\u0000\u0000\u0000\u0000\u0000\u0000\u0000\u0000\u0000\u0000ÿÿ\u0000\u0000\u0000\u0000\u0000\u0000", "PMU.025\u0000\u0000\u0000\u0000\u0000\u0000\u0000\u0000\u0000\u0000\u0019\u0000\u000f\u0000\u0006\u0000\u0003\u0000\u0001PZR.AI          PZR.BV          PZR.CI          PZR.AV          PZR.BI          PZR.CV          ANA1            ANA2            ANA3            DIG.stat1_01    DIG.stat1_02    DIG.stat1_03    DIG.stat1_04    DIG.stat1_05    DIG.stat1_06    DIG.stat1_07    DIG.stat1_08    DIG.stat1_09    DIG.stat1_10    DIG.stat1_11    DIG.stat1_12    DIG.stat1_13    DIG.stat1_14    DIG.stat1_15    DIG.stat1_16    \u0001\u0000\u0000\u0000\u0000\u0000\u0000\u0000\u0001\u0000\u0000\u0000\u0000\u0000\u0000\u0000\u0001\u0000\u0000\u0000\u0000\u0000\u0000\u0000\u0000\u0000\u0000\u0000\u0000\u0000\u0000\u0000\u0000\u0000\u0000\u0000ÿÿ\u0000\u0000\u0000\u0000\u0000\u0000", "PMU.026\u0000\u0000\u0000\u0000\u0000\u0000\u0000\u0000\u0000\u0000\u001a\u0000\u000f\u0000\u0006\u0000\u0003\u0000\u0001PZR.AI          PZR.BV          PZR.CI          PZR.AV          PZR.BI          PZR.CV          ANA1            ANA2            ANA3            DIG.stat1_01    DIG.stat1_02    DIG.stat1_03    DIG.stat1_04    DIG.stat1_05    DIG.stat1_06    DIG.stat1_07    DIG.stat1_08    DIG.stat1_09    DIG.stat1_10    DIG.stat1_11    DIG.stat1_12    DIG.stat1_13    DIG.stat1_14    DIG.stat1_15    DIG.stat1_16    \u0001\u0000\u0000\u0000\u0000\u0000\u0000\u0000\u0001\u0000\u0000\u0000\u0000\u0000\u0000\u0000\u0001\u0000\u0000\u0000\u0000\u0000\u0000\u0000\u0000\u0000\u0000\u0000\u0000\u0000\u0000\u0000\u0000\u0000\u0000\u0000ÿÿ\u0000\u0000\u0000\u0000\u0000\u0000", "PMU.027\u0000\u0000\u0000\u0000\u0000\u0000\u0000\u0000\u0000\u0000\u001b\u0000\u000f\u0000\u0006\u0000\u0003\u0000\u0001PZR.AI          PZR.BV          PZR.CI          PZR.AV          PZR.BI          PZR.CV          ANA1            ANA2            ANA3            DIG.stat1_01    DIG.stat1_02    DIG.stat1_03    DIG.stat1_04    DIG.stat1_05    DIG.stat1_06    DIG.stat1_07    DIG.stat1_08    DIG.stat1_09    DIG.stat1_10    DIG.stat1_11    DIG.stat1_12    DIG.stat1_13    DIG.stat1_14    DIG.stat1_15    DIG.stat1_16    \u0001\u0000\u0000\u0000\u0000\u0000\u0000\u0000\u0001\u0000\u0000\u0000\u0000\u0000\u0000\u0000\u0001\u0000\u0000\u0000\u0000\u0000\u0000\u0000\u0000\u0000\u0000\u0000\u0000\u0000\u0000\u0000\u0000\u0000\u0000\u0000ÿÿ\u0000\u0000\u0000\u0000\u0000\u0000", "PMU.028\u0000\u0000\u0000\u0000\u0000\u0000\u0000\u0000\u0000\u0000\u001c\u0000\u000f\u0000\u0006\u0000\u0003\u0000\u0001PZR.AI          PZR.BV          PZR.CI          PZR.AV          PZR.BI          PZR.CV          ANA1            ANA2            ANA3            DIG.stat1_01    DIG.stat1_02    DIG.stat1_03    DIG.stat1_04    DIG.stat1_05    DIG.stat1_06    DIG.stat1_07    DIG.stat1_08    DIG.stat1_09    DIG.stat1_10    DIG.stat1_11    DIG.stat1_12    DIG.stat1_13    DIG.stat1_14    DIG.stat1_15    DIG.stat1_16    \u0001\u0000\u0000\u0000\u0000\u0000\u0000\u0000\u0001\u0000\u0000\u0000\u0000\u0000\u0000\u0000\u0001\u0000\u0000\u0000\u0000\u0000\u0000\u0000\u0000\u0000\u0000\u0000\u0000\u0000\u0000\u0000\u0000\u0000\u0000\u0000ÿÿ\u0000\u0000\u0000\u0000\u0000\u0000", "PMU.029\u0000\u0000\u0000\u0000\u0000\u0000\u0000\u0000\u0000\u0000\u001d\u0000\u000f\u0000\u0006\u0000\u0003\u0000\u0001PZR.AI          PZR.BV          PZR.CI          PZR.AV          PZR.BI          PZR.CV          ANA1            ANA2            ANA3            DIG.stat1_01    DIG.stat1_02    DIG.stat1_03    DIG.stat1_04    DIG.stat1_05    DIG.stat1_06    DIG.stat1_07    DIG.stat1_08    DIG.stat1_09    DIG.stat1_10    DIG.stat1_11    DIG.stat1_12    DIG.stat1_13    DIG.stat1_14    DIG.stat1_15    DIG.stat1_16    \u0001\u0000\u0000\u0000\u0000\u0000\u0000\u0000\u0001\u0000\u0000\u0000\u0000\u0000\u0000\u0000\u0001\u0000\u0000\u0000\u0000\u0000\u0000\u0000\u0000\u0000\u0000\u0000\u0000\u0000\u0000\u0000\u0000\u0000\u0000\u0000ÿÿ\u0000\u0000\u0000\u0000\u0000\u0000", "PMU.030\u0000\u0000\u0000\u0000\u0000\u0000\u0000\u0000\u0000\u0000\u001e\u0000\u000f\u0000\u0006\u0000\u0003\u0000\u0001PZR.AI          PZR.BV          PZR.CI          PZR.AV          PZR.BI          PZR.CV          ANA1            ANA2            ANA3            DIG.stat1_01    DIG.stat1_02    DIG.stat1_03    DIG.stat1_04    DIG.stat1_05    DIG.stat1_06    DIG.stat1_07    DIG.stat1_08    DIG.stat1_09    DIG.stat1_10    DIG.stat1_11    DIG.stat1_12    DIG.stat1_13    DIG.stat1_14    DIG.stat1_15    DIG.stat1_16    \u0001\u0000\u0000\u0000\u0000\u0000\u0000\u0000\u0001\u0000\u0000\u0000\u0000\u0000\u0000\u0000\u0001\u0000\u0000\u0000\u0000\u0000\u0000\u0000\u0000\u0000\u0000\u0000\u0000\u0000\u0000\u0000\u0000\u0000\u0000\u0000ÿÿ\u0000\u0000\u0000\u0000\u0000\u0000", "PMU.031\u0000\u0000\u0000\u0000\u0000\u0000\u0000\u0000\u0000\u0000\u001f\u0000\u000f\u0000\u0006\u0000\u0003\u0000\u0001PZR.AI          PZR.BV          PZR.CI          PZR.AV          PZR.BI          PZR.CV          ANA1            ANA2            ANA3            DIG.stat1_01    DIG.stat1_02    DIG.stat1_03    DIG.stat1_04    DIG.stat1_05    DIG.stat1_06    DIG.stat1_07    DIG.stat1_08    DIG.stat1_09    DIG.stat1_10    DIG.stat1_11    DIG.stat1_12    DIG.stat1_13    DIG.stat1_14    DIG.stat1_15    DIG.stat1_16    \u0001\u0000\u0000\u0000\u0000\u0000\u0000\u0000\u0001\u0000\u0000\u0000\u0000\u0000\u0000\u0000\u0001\u0000\u0000\u0000\u0000\u0000\u0000\u0000\u0000\u0000\u0000\u0000\u0000\u0000\u0000\u0000\u0000\u0000\u0000\u0000ÿÿ\u0000\u0000\u0000\u0000\u0000\u0000", "PMU.032\u0000\u0000\u0000\u0000\u0000\u0000\u0000\u0000\u0000\u0000 \u0000\u000f\u0000\u0006\u0000\u0003\u0000\u0001PZR.AI          PZR.BV          PZR.CI          PZR.AV          PZR.BI          PZR.CV          ANA1            ANA2            ANA3            DIG.stat1_01    DIG.stat1_02    DIG.stat1_03    DIG.stat1_04    DIG.stat1_05    DIG.stat1_06    DIG.stat1_07    DIG.stat1_08    DIG.stat1_09    DIG.stat1_10    DIG.stat1_11    DIG.stat1_12    DIG.stat1_13    DIG.stat1_14    DIG.stat1_15    DIG.stat1_16    \u0001\u0000\u0000\u0000\u0000\u0000\u0000\u0000\u0001\u0000\u0000\u0000\u0000\u0000\u0000\u0000\u0001\u0000\u0000\u0000\u0000\u0000\u0000\u0000\u0000\u0000\u0000\u0000\u0000\u0000\u0000\u0000\u0000\u0000\u0000\u0000ÿÿ\u0000\u0000\u0000\u0000\u0000\u0000", "PMU.033\u0000\u0000\u0000\u0000\u0000\u0000\u0000\u0000\u0000\u0000!\u0000\u000f\u0000\u0006\u0000\u0003\u0000\u0001PZR.AI          PZR.BV          PZR.CI          PZR.AV          PZR.BI          PZR.CV          ANA1            ANA2            ANA3            DIG.stat1_01    DIG.stat1_02    DIG.stat1_03    DIG.stat1_04    DIG.stat1_05    DIG.stat1_06    DIG.stat1_07    DIG.stat1_08    DIG.stat1_09    DIG.stat1_10    DIG.stat1_11    DIG.stat1_12    DIG.stat1_13    DIG.stat1_14    DIG.stat1_15    DIG.stat1_16    \u0001\u0000\u0000\u0000\u0000\u0000\u0000\u0000\u0001\u0000\u0000\u0000\u0000\u0000\u0000\u0000\u0001\u0000\u0000\u0000\u0000\u0000\u0000\u0000\u0000\u0000\u0000\u0000\u0000\u0000\u0000\u0000\u0000\u0000\u0000\u0000ÿÿ\u0000\u0000\u0000\u0000\u0000\u0000", "PMU.034\u0000\u0000\u0000\u0000\u0000\u0000\u0000\u0000\u0000\u0000\"\u0000\u000f\u0000\u0006\u0000\u0003\u0000\u0001PZR.AI          PZR.BV          PZR.CI          PZR.AV          PZR.BI          PZR.CV          ANA1            ANA2            ANA3            DIG.stat1_01    DIG.stat1_02    DIG.stat1_03    DIG.stat1_04    DIG.stat1_05    DIG.stat1_06    DIG.stat1_07    DIG.stat1_08    DIG.stat1_09    DIG.stat1_10    DIG.stat1_11    DIG.stat1_12    DIG.stat1_13    DIG.stat1_14    DIG.stat1_15    DIG.stat1_16    \u0001\u0000\u0000\u0000\u0000\u0000\u0000\u0000\u0001\u0000\u0000\u0000\u0000\u0000\u0000\u0000\u0001\u0000\u0000\u0000\u0000\u0000\u0000\u0000\u0000\u0000\u0000\u0000\u0000\u0000\u0000\u0000\u0000\u0000\u0000\u0000ÿÿ\u0000\u0000\u0000\u0000\u0000\u0000", "PMU.035\u0000\u0000\u0000\u0000\u0000\u0000\u0000\u0000\u0000\u0000#\u0000\u000f\u0000\u0006\u0000\u0003\u0000\u0001PZR.AI          PZR.BV          PZR.CI          PZR.AV          PZR.BI          PZR.CV          ANA1            ANA2            ANA3            DIG.stat1_01    DIG.stat1_02    DIG.stat1_03    DIG.stat1_04    DIG.stat1_05    DIG.stat1_06    DIG.stat1_07    DIG.stat1_08    DIG.stat1_09    DIG.stat1_10    DIG.stat1_11    DIG.stat1_12    DIG.stat1_13    DIG.stat1_14    DIG.stat1_15    DIG.stat1_16    \u0001\u0000\u0000\u0000\u0000\u0000\u0000\u0000\u0001\u0000\u0000\u0000\u0000\u0000\u0000\u0000\u0001\u0000\u0000\u0000\u0000\u0000\u0000\u0000\u0000\u0000\u0000\u0000\u0000\u0000\u0000\u0000\u0000\u0000\u0000\u0000ÿÿ\u0000\u0000\u0000\u0000\u0000\u0000", "PMU.036\u0000\u0000\u0000\u0000\u0000\u0000\u0000\u0000\u0000\u0000$\u0000\u000f\u0000\u0006\u0000\u0003\u0000\u0001PZR.AI          PZR.BV          PZR.CI          PZR.AV          PZR.BI          PZR.CV          ANA1            ANA2            ANA3            DIG.stat1_01    DIG.stat1_02    DIG.stat1_03    DIG.stat1_04    DIG.stat1_05    DIG.stat1_06    DIG.stat1_07    DIG.stat1_08    DIG.stat1_09    DIG.stat1_10    DIG.stat1_11    DIG.stat1_12    DIG.stat1_13    DIG.stat1_14    DIG.stat1_15    DIG.stat1_16    \u0001\u0000\u0000\u0000\u0000\u0000\u0000\u0000\u0001\u0000\u0000\u0000\u0000\u0000\u0000\u0000\u0001\u0000\u0000\u0000\u0000\u0000\u0000\u0000\u0000\u0000\u0000\u0000\u0000\u0000\u0000\u0000\u0000\u0000\u0000\u0000ÿÿ\u0000\u0000\u0000\u0000\u0000\u0000", "PMU.037\u0000\u0000\u0000\u0000\u0000\u0000\u0000\u0000\u0000\u0000%\u0000\u000f\u0000\u0006\u0000\u0003\u0000\u0001PZR.AI          PZR.BV          PZR.CI          PZR.AV          PZR.BI          PZR.CV          ANA1            ANA2            ANA3            DIG.stat1_01    DIG.stat1_02    DIG.stat1_03    DIG.stat1_04    DIG.stat1_05    DIG.stat1_06    DIG.stat1_07    DIG.stat1_08    DIG.stat1_09    DIG.stat1_10    DIG.stat1_11    DIG.stat1_12    DIG.stat1_13    DIG.stat1_14    DIG.stat1_15    DIG.stat1_16    \u0001\u0000\u0000\u0000\u0000\u0000\u0000\u0000\u0001\u0000\u0000\u0000\u0000\u0000\u0000\u0000\u0001\u0000\u0000\u0000\u0000\u0000\u0000\u0000\u0000\u0000\u0000\u0000\u0000\u0000\u0000\u0000\u0000\u0000\u0000\u0000ÿÿ\u0000\u0000\u0000\u0000\u0000\u0000", "PMU.038\u0000\u0000\u0000\u0000\u0000\u0000\u0000\u0000\u0000\u0000&\u0000\u000f\u0000\u0006\u0000\u0003\u0000\u0001PZR.AI          PZR.BV          PZR.CI          PZR.AV          PZR.BI          PZR.CV          ANA1            ANA2            ANA3            DIG.stat1_01    DIG.stat1_02    DIG.stat1_03    DIG.stat1_04    DIG.stat1_05    DIG.stat1_06    DIG.stat1_07    DIG.stat1_08    DIG.stat1_09    DIG.stat1_10    DIG.stat1_11    DIG.stat1_12    DIG.stat1_13    DIG.stat1_14    DIG.stat1_15    DIG.stat1_16    \u0001\u0000\u0000\u0000\u0000\u0000\u0000\u0000\u0001\u0000\u0000\u0000\u0000\u0000\u0000\u0000\u0001\u0000\u0000\u0000\u0000\u0000\u0000\u0000\u0000\u0000\u0000\u0000\u0000\u0000\u0000\u0000\u0000\u0000\u0000\u0000ÿÿ\u0000\u0000\u0000\u0000\u0000\u0000", "PMU.039\u0000\u0000\u0000\u0000\u0000\u0000\u0000\u0000\u0000\u0000'\u0000\u000f\u0000\u0006\u0000\u0003\u0000\u0001PZR.AI          PZR.BV          PZR.CI          PZR.AV          PZR.BI          PZR.CV          ANA1            ANA2            ANA3            DIG.stat1_01    DIG.stat1_02    DIG.stat1_03    DIG.stat1_04    DIG.stat1_05    DIG.stat1_06    DIG.stat1_07    DIG.stat1_08    DIG.stat1_09    DIG.stat1_10    DIG.stat1_11    DIG.stat1_12    DIG.stat1_13    DIG.stat1_14    DIG.stat1_15    DIG.stat1_16    \u0001\u0000\u0000\u0000\u0000\u0000\u0000\u0000\u0001\u0000\u0000\u0000\u0000\u0000\u0000\u0000\u0001\u0000\u0000\u0000\u0000\u0000\u0000\u0000\u0000\u0000\u0000\u0000\u0000\u0000\u0000\u0000\u0000\u0000\u0000\u0000ÿÿ\u0000\u0000\u0000\u0000\u0000\u0000", "PMU.040\u0000\u0000\u0000\u0000\u0000\u0000\u0000\u0000\u0000\u0000(\u0000\u000f\u0000\u0006\u0000\u0003\u0000\u0001PZR.AI          PZR.BV          PZR.CI          PZR.AV          PZR.BI          PZR.CV          ANA1            ANA2            ANA3            DIG.stat1_01    DIG.stat1_02    DIG.stat1_03    DIG.stat1_04    DIG.stat1_05    DIG.stat1_06    DIG.stat1_07    DIG.stat1_08    DIG.stat1_09    DIG.stat1_10    DIG.stat1_11    DIG.stat1_12    DIG.stat1_13    DIG.stat1_14    DIG.stat1_15    DIG.stat1_16    \u0001\u0000\u0000\u0000\u0000\u0000\u0000\u0000\u0001\u0000\u0000\u0000\u0000\u0000\u0000\u0000\u0001\u0000\u0000\u0000\u0000\u0000\u0000\u0000\u0000\u0000\u0000\u0000\u0000\u0000\u0000\u0000\u0000\u0000\u0000\u0000ÿÿ\u0000\u0000\u0000\u0000\u0000\u0000", "PMU.041\u0000\u0000\u0000\u0000\u0000\u0000\u0000\u0000\u0000\u0000)\u0000\u000f\u0000\u0006\u0000\u0003\u0000\u0001PZR.AI          PZR.BV          PZR.CI          PZR.AV          PZR.BI          PZR.CV          ANA1            ANA2            ANA3            DIG.stat1_01    DIG.stat1_02    DIG.stat1_03    DIG.stat1_04    DIG.stat1_05    DIG.stat1_06    DIG.stat1_07    DIG.stat1_08    DIG.stat1_09    DIG.stat1_10    DIG.stat1_11    DIG.stat1_12    DIG.stat1_13    DIG.stat1_14    DIG.stat1_15    DIG.stat1_16    \u0001\u0000\u0000\u0000\u0000\u0000\u0000\u0000\u0001\u0000\u0000\u0000\u0000\u0000\u0000\u0000\u0001\u0000\u0000\u0000\u0000\u0000\u0000\u0000\u0000\u0000\u0000\u0000\u0000\u0000\u0000\u0000\u0000\u0000\u0000\u0000ÿÿ\u0000\u0000\u0000\u0000\u0000\u0000", "PMU.042\u0000\u0000\u0000\u0000\u0000\u0000\u0000\u0000\u0000\u0000*\u0000\u000f\u0000\u0006\u0000\u0003\u0000\u0001PZR.AI          PZR.BV          PZR.CI          PZR.AV          PZR.BI          PZR.CV          ANA1            ANA2            ANA3            DIG.stat1_01    DIG.stat1_02    DIG.stat1_03    DIG.stat1_04    DIG.stat1_05    DIG.stat1_06    DIG.stat1_07    DIG.stat1_08    DIG.stat1_09    DIG.stat1_10    DIG.stat1_11    DIG.stat1_12    DIG.stat1_13    DIG.stat1_14    DIG.stat1_15    DIG.stat1_16    \u0001\u0000\u0000\u0000\u0000\u0000\u0000\u0000\u0001\u0000\u0000\u0000\u0000\u0000\u0000\u0000\u0001\u0000\u0000\u0000\u0000\u0000\u0000\u0000\u0000\u0000\u0000\u0000\u0000\u0000\u0000\u0000\u0000\u0000\u0000\u0000ÿÿ\u0000\u0000\u0000\u0000\u0000\u0000", "PMU.043\u0000\u0000\u0000\u0000\u0000\u0000\u0000\u0000\u0000\u0000+\u0000\u000f\u0000\u0006\u0000\u0003\u0000\u0001PZR.AI          PZR.BV          PZR.CI          PZR.AV          PZR.BI          PZR.CV          ANA1            ANA2            ANA3            DIG.stat1_01    DIG.stat1_02    DIG.stat1_03    DIG.stat1_04    DIG.stat1_05    DIG.stat1_06    DIG.stat1_07    DIG.stat1_08    DIG.stat1_09    DIG.stat1_10    DIG.stat1_11    DIG.stat1_12    DIG.stat1_13    DIG.stat1_14    DIG.stat1_15    DIG.stat1_16    \u0001\u0000\u0000\u0000\u0000\u0000\u0000\u0000\u0001\u0000\u0000\u0000\u0000\u0000\u0000\u0000\u0001\u0000\u0000\u0000\u0000\u0000\u0000\u0000\u0000\u0000\u0000\u0000\u0000\u0000\u0000\u0000\u0000\u0000\u0000\u0000ÿÿ\u0000\u0000\u0000\u0000\u0000\u0000", "PMU.044\u0000\u0000\u0000\u0000\u0000\u0000\u0000\u0000\u0000\u0000,\u0000\u000f\u0000\u0006\u0000\u0003\u0000\u0001PZR.AI          PZR.BV          PZR.CI          PZR.AV          PZR.BI          PZR.CV          ANA1            ANA2            ANA3            DIG.stat1_01    DIG.stat1_02    DIG.stat1_03    DIG.stat1_04    DIG.stat1_05    DIG.stat1_06    DIG.stat1_07    DIG.stat1_08    DIG.stat1_09    DIG.stat1_10    DIG.stat1_11    DIG.stat1_12    DIG.stat1_13    DIG.stat1_14    DIG.stat1_15    DIG.stat1_16    \u0001\u0000\u0000\u0000\u0000\u0000\u0000\u0000\u0001\u0000\u0000\u0000\u0000\u0000\u0000\u0000\u0001\u0000\u0000\u0000\u0000\u0000\u0000\u0000\u0000\u0000\u0000\u0000\u0000\u0000\u0000\u0000\u0000\u0000\u0000\u0000ÿÿ\u0000\u0000\u0000\u0000\u0000\u0000", "PMU.045\u0000\u0000\u0000\u0000\u0000\u0000\u0000\u0000\u0000\u0000-\u0000\u000f\u0000\u0006\u0000\u0003\u0000\u0001PZR.AI          PZR.BV          PZR.CI          PZR.AV          PZR.BI          PZR.CV          ANA1            ANA2            ANA3            DIG.stat1_01    DIG.stat1_02    DIG.stat1_03    DIG.stat1_04    DIG.stat1_05    DIG.stat1_06    DIG.stat1_07    DIG.stat1_08    DIG.stat1_09    DIG.stat1_10    DIG.stat1_11    DIG.stat1_12    DIG.stat1_13    DIG.stat1_14    DIG.stat1_15    DIG.stat1_16    \u0001\u0000\u0000\u0000\u0000\u0000\u0000\u0000\u0001\u0000\u0000\u0000\u0000\u0000\u0000\u0000\u0001\u0000\u0000\u0000\u0000\u0000\u0000\u0000\u0000\u0000\u0000\u0000\u0000\u0000\u0000\u0000\u0000\u0000\u0000\u0000ÿÿ\u0000\u0000\u0000\u0000\u0000\u0000", "PMU.046\u0000\u0000\u0000\u0000\u0000\u0000\u0000\u0000\u0000\u0000.\u0000\u000f\u0000\u0006\u0000\u0003\u0000\u0001PZR.AI          PZR.BV          PZR.CI          PZR.AV          PZR.BI          PZR.CV          ANA1            ANA2            ANA3            DIG.stat1_01    DIG.stat1_02    DIG.stat1_03    DIG.stat1_04    DIG.stat1_05    DIG.stat1_06    DIG.stat1_07    DIG.stat1_08    DIG.stat1_09    DIG.stat1_10    DIG.stat1_11    DIG.stat1_12    DIG.stat1_13    DIG.stat1_14    DIG.stat1_15    DIG.stat1_16    \u0001\u0000\u0000\u0000\u0000\u0000\u0000\u0000\u0001\u0000\u0000\u0000\u0000\u0000\u0000\u0000\u0001\u0000\u0000\u0000\u0000\u0000\u0000\u0000\u0000\u0000\u0000\u0000\u0000\u0000\u0000\u0000\u0000\u0000\u0000\u0000ÿÿ\u0000\u0000\u0000\u0000\u0000\u0000", "PMU.047\u0000\u0000\u0000\u0000\u0000\u0000\u0000\u0000\u0000\u0000/\u0000\u000f\u0000\u0006\u0000\u0003\u0000\u0001PZR.AI          PZR.BV          PZR.CI          PZR.AV          PZR.BI          PZR.CV          ANA1            ANA2            ANA3            DIG.stat1_01    DIG.stat1_02    DIG.stat1_03    DIG.stat1_04    DIG.stat1_05    DIG.stat1_06    DIG.stat1_07    DIG.stat1_08    DIG.stat1_09    DIG.stat1_10    DIG.stat1_11    DIG.stat1_12    DIG.stat1_13    DIG.stat1_14    DIG.stat1_15    DIG.stat1_16    \u0001\u0000\u0000\u0000\u0000\u0000\u0000\u0000\u0001\u0000\u0000\u0000\u0000\u0000\u0000\u0000\u0001\u0000\u0000\u0000\u0000\u0000\u0000\u0000\u0000\u0000\u0000\u0000\u0000\u0000\u0000\u0000\u0000\u0000\u0000\u0000ÿÿ\u0000\u0000\u0000\u0000\u0000\u0000", "PMU.048\u0000\u0000\u0000\u0000\u0000\u0000\u0000\u0000\u0000\u00000\u0000\u000f\u0000\u0006\u0000\u0003\u0000\u0001PZR.AI          PZR.BV          PZR.CI          PZR.AV          PZR.BI          PZR.CV          ANA1            ANA2            ANA3            DIG.stat1_01    DIG.stat1_02    DIG.stat1_03    DIG.stat1_04    DIG.stat1_05    DIG.stat1_06    DIG.stat1_07    DIG.stat1_08    DIG.stat1_09    DIG.stat1_10    DIG.stat1_11    DIG.stat1_12    DIG.stat1_13    DIG.stat1_14    DIG.stat1_15    DIG.stat1_16    \u0001\u0000\u0000\u0000\u0000\u0000\u0000\u0000\u0001\u0000\u0000\u0000\u0000\u0000\u0000\u0000\u0001\u0000\u0000\u0000\u0000\u0000\u0000\u0000\u0000\u0000\u0000\u0000\u0000\u0000\u0000\u0000\u0000\u0000\u0000\u0000ÿÿ\u0000\u0000\u0000\u0000\u0000\u0000", "PMU.049\u0000\u0000\u0000\u0000\u0000\u0000\u0000\u0000\u0000\u00001\u0000\u000f\u0000\u0006\u0000\u0003\u0000\u0001PZR.AI          PZR.BV          PZR.CI          PZR.AV          PZR.BI          PZR.CV          ANA1            ANA2            ANA3            DIG.stat1_01    DIG.stat1_02    DIG.stat1_03    DIG.stat1_04    DIG.stat1_05    DIG.stat1_06    DIG.stat1_07    DIG.stat1_08    DIG.stat1_09    DIG.stat1_10    DIG.stat1_11    DIG.stat1_12    DIG.stat1_13    DIG.stat1_14    DIG.stat1_15    DIG.stat1_16    \u0001\u0000\u0000\u0000\u0000\u0000\u0000\u0000\u0001\u0000\u0000\u0000\u0000\u0000\u0000\u0000\u0001\u0000\u0000\u0000\u0000\u0000\u0000\u0000\u0000\u0000\u0000\u0000\u0000\u0000\u0000\u0000\u0000\u0000\u0000\u0000ÿÿ\u0000\u0000\u0000\u0000\u0000\u0000", "PMU.050\u0000\u0000\u0000\u0000\u0000\u0000\u0000\u0000\u0000\u00002\u0000\u000f\u0000\u0006\u0000\u0003\u0000\u0001PZR.AI          PZR.BV          PZR.CI          PZR.AV          PZR.BI          PZR.CV          ANA1            ANA2            ANA3            DIG.stat1_01    DIG.stat1_02    DIG.stat1_03    DIG.stat1_04    DIG.stat1_05    DIG.stat1_06    DIG.stat1_07    DIG.stat1_08    DIG.stat1_09    DIG.stat1_10    DIG.stat1_11    DIG.stat1_12    DIG.stat1_13    DIG.stat1_14    DIG.stat1_15    DIG.stat1_16    \u0001\u0000\u0000\u0000\u0000\u0000\u0000\u0000\u0001\u0000\u0000\u0000\u0000\u0000\u0000\u0000\u0001\u0000\u0000\u0000\u0000\u0000\u0000\u0000\u0000\u0000\u0000\u0000\u0000\u0000\u0000\u0000\u0000\u0000\u0000\u0000ÿÿ\u0000\u0000\u0000\u0000\u0000\u0000", "PMU.051\u0000\u0000\u0000\u0000\u0000\u0000\u0000\u0000\u0000\u00003\u0000\u000f\u0000\u0006\u0000\u0003\u0000\u0001PZR.AI          PZR.BV          PZR.CI          PZR.AV          PZR.BI          PZR.CV          ANA1            ANA2            ANA3            DIG.stat1_01    DIG.stat1_02    DIG.stat1_03    DIG.stat1_04    DIG.stat1_05    DIG.stat1_06    DIG.stat1_07    DIG.stat1_08    DIG.stat1_09    DIG.stat1_10    DIG.stat1_11    DIG.stat1_12    DIG.stat1_13    DIG.stat1_14    DIG.stat1_15    DIG.stat1_16    \u0001\u0000\u0000\u0000\u0000\u0000\u0000\u0000\u0001\u0000\u0000\u0000\u0000\u0000\u0000\u0000\u0001\u0000\u0000\u0000\u0000\u0000\u0000\u0000\u0000\u0000\u0000\u0000\u0000\u0000\u0000\u0000\u0000\u0000\u0000\u0000ÿÿ\u0000\u0000\u0000\u0000\u0000\u0000", "PMU.052\u0000\u0000\u0000\u0000\u0000\u0000\u0000\u0000\u0000\u00004\u0000\u000f\u0000\u0006\u0000\u0003\u0000\u0001PZR.AI          PZR.BV          PZR.CI          PZR.AV          PZR.BI          PZR.CV          ANA1            ANA2            ANA3            DIG.stat1_01    DIG.stat1_02    DIG.stat1_03    DIG.stat1_04    DIG.stat1_05    DIG.stat1_06    DIG.stat1_07    DIG.stat1_08    DIG.stat1_09    DIG.stat1_10    DIG.stat1_11    DIG.stat1_12    DIG.stat1_13    DIG.stat1_14    DIG.stat1_15    DIG.stat1_16    \u0001\u0000\u0000\u0000\u0000\u0000\u0000\u0000\u0001\u0000\u0000\u0000\u0000\u0000\u0000\u0000\u0001\u0000\u0000\u0000\u0000\u0000\u0000\u0000\u0000\u0000\u0000\u0000\u0000\u0000\u0000\u0000\u0000\u0000\u0000\u0000ÿÿ\u0000\u0000\u0000\u0000\u0000\u0000", "PMU.053\u0000\u0000\u0000\u0000\u0000\u0000\u0000\u0000\u0000\u00005\u0000\u000f\u0000\u0006\u0000\u0003\u0000\u0001PZR.AI          PZR.BV          PZR.CI          PZR.AV          PZR.BI          PZR.CV          ANA1            ANA2            ANA3            DIG.stat1_01    DIG.stat1_02    DIG.stat1_03    DIG.stat1_04    DIG.stat1_05    DIG.stat1_06    DIG.stat1_07    DIG.stat1_08    DIG.stat1_09    DIG.stat1_10    DIG.stat1_11    DIG.stat1_12    DIG.stat1_13    DIG.stat1_14    DIG.stat1_15    DIG.stat1_16    \u0001\u0000\u0000\u0000\u0000\u0000\u0000\u0000\u0001\u0000\u0000\u0000\u0000\u0000\u0000\u0000\u0001\u0000\u0000\u0000\u0000\u0000\u0000\u0000\u0000\u0000\u0000\u0000\u0000\u0000\u0000\u0000\u0000\u0000\u0000\u0000ÿÿ\u0000\u0000\u0000\u0000\u0000\u0000", "PMU.054\u0000\u0000\u0000\u0000\u0000\u0000\u0000\u0000\u0000\u00006\u0000\u000f\u0000\u0006\u0000\u0003\u0000\u0001PZR.AI          PZR.BV          PZR.CI          PZR.AV          PZR.BI          PZR.CV          ANA1            ANA2            ANA3            DIG.stat1_01    DIG.stat1_02    DIG.stat1_03    DIG.stat1_04    DIG.stat1_05    DIG.stat1_06    DIG.stat1_07    DIG.stat1_08    DIG.stat1_09    DIG.stat1_10    DIG.stat1_11    DIG.stat1_12    DIG.stat1_13    DIG.stat1_14    DIG.stat1_15    DIG.stat1_16    \u0001\u0000\u0000\u0000\u0000\u0000\u0000\u0000\u0001\u0000\u0000\u0000\u0000\u0000\u0000\u0000\u0001\u0000\u0000\u0000\u0000\u0000\u0000\u0000\u0000\u0000\u0000\u0000\u0000\u0000\u0000\u0000\u0000\u0000\u0000\u0000ÿÿ\u0000\u0000\u0000\u0000\u0000\u0000", "PMU.055\u0000\u0000\u0000\u0000\u0000\u0000\u0000\u0000\u0000\u00007\u0000\u000f\u0000\u0006\u0000\u0003\u0000\u0001PZR.AI          PZR.BV          PZR.CI          PZR.AV          PZR.BI          PZR.CV          ANA1            ANA2            ANA3            DIG.stat1_01    DIG.stat1_02    DIG.stat1_03    DIG.stat1_04    DIG.stat1_05    DIG.stat1_06    DIG.stat1_07    DIG.stat1_08    DIG.stat1_09    DIG.stat1_10    DIG.stat1_11    DIG.stat1_12    DIG.stat1_13    DIG.stat1_14    DIG.stat1_15    DIG.stat1_16    \u0001\u0000\u0000\u0000\u0000\u0000\u0000\u0000\u0001\u0000\u0000\u0000\u0000\u0000\u0000\u0000\u0001\u0000\u0000\u0000\u0000\u0000\u0000\u0000\u0000\u0000\u0000\u0000\u0000\u0000\u0000\u0000\u0000\u0000\u0000\u0000ÿÿ\u0000\u0000\u0000\u0000\u0000\u0000", "PMU.056\u0000\u0000\u0000\u0000\u0000\u0000\u0000\u0000\u0000\u00008\u0000\u000f\u0000\u0006\u0000\u0003\u0000\u0001PZR.AI          PZR.BV          PZR.CI          PZR.AV          PZR.BI          PZR.CV          ANA1            ANA2            ANA3            DIG.stat1_01    DIG.stat1_02    DIG.stat1_03    DIG.stat1_04    DIG.stat1_05    DIG.stat1_06    DIG.stat1_07    DIG.stat1_08    DIG.stat1_09    DIG.stat1_10    DIG.stat1_11    DIG.stat1_12    DIG.stat1_13    DIG.stat1_14    DIG.stat1_15    DIG.stat1_16    \u0001\u0000\u0000\u0000\u0000\u0000\u0000\u0000\u0001\u0000\u0000\u0000\u0000\u0000\u0000\u0000\u0001\u0000\u0000\u0000\u0000\u0000\u0000\u0000\u0000\u0000\u0000\u0000\u0000\u0000\u0000\u0000\u0000\u0000\u0000\u0000ÿÿ\u0000\u0000\u0000\u0000\u0000\u0000", "PMU.057\u0000\u0000\u0000\u0000\u0000\u0000\u0000\u0000\u0000\u00009\u0000\u000f\u0000\u0006\u0000\u0003\u0000\u0001PZR.AI          PZR.BV          PZR.CI          PZR.AV          PZR.BI          PZR.CV          ANA1            ANA2            ANA3            DIG.stat1_01    DIG.stat1_02    DIG.stat1_03    DIG.stat1_04    DIG.stat1_05    DIG.stat1_06    DIG.stat1_07    DIG.stat1_08    DIG.stat1_09    DIG.stat1_10    DIG.stat1_11    DIG.stat1_12    DIG.stat1_13    DIG.stat1_14    DIG.stat1_15    DIG.stat1_16    \u0001\u0000\u0000\u0000\u0000\u0000\u0000\u0000\u0001\u0000\u0000\u0000\u0000\u0000\u0000\u0000\u0001\u0000\u0000\u0000\u0000\u0000\u0000\u0000\u0000\u0000\u0000\u0000\u0000\u0000\u0000\u0000\u0000\u0000\u0000\u0000ÿÿ\u0000\u0000\u0000\u0000\u0000\u0000", "PMU.058\u0000\u0000\u0000\u0000\u0000\u0000\u0000\u0000\u0000\u0000:\u0000\u000f\u0000\u0006\u0000\u0003\u0000\u0001PZR.AI          PZR.BV          PZR.CI          PZR.AV          PZR.BI          PZR.CV          ANA1            ANA2            ANA3            DIG.stat1_01    DIG.stat1_02    DIG.stat1_03    DIG.stat1_04    DIG.stat1_05    DIG.stat1_06    DIG.stat1_07    DIG.stat1_08    DIG.stat1_09    DIG.stat1_10    DIG.stat1_11    DIG.stat1_12    DIG.stat1_13    DIG.stat1_14    DIG.stat1_15    DIG.stat1_16    \u0001\u0000\u0000\u0000\u0000\u0000\u0000\u0000\u0001\u0000\u0000\u0000\u0000\u0000\u0000\u0000\u0001\u0000\u0000\u0000\u0000\u0000\u0000\u0000\u0000\u0000\u0000\u0000\u0000\u0000\u0000\u0000\u0000\u0000\u0000\u0000ÿÿ\u0000\u0000\u0000\u0000\u0000\u0000", "PMU.059\u0000\u0000\u0000\u0000\u0000\u0000\u0000\u0000\u0000\u0000;\u0000\u000f\u0000\u0006\u0000\u0003\u0000\u0001PZR.AI          PZR.BV          PZR.CI          PZR.AV          PZR.BI          PZR.CV          ANA1            ANA2            ANA3            DIG.stat1_01    DIG.stat1_02    DIG.stat1_03    DIG.stat1_04    DIG.stat1_05    DIG.stat1_06    DIG.stat1_07    DIG.stat1_08    DIG.stat1_09    DIG.stat1_10    DIG.stat1_11    DIG.stat1_12    DIG.stat1_13    DIG.stat1_14    DIG.stat1_15    DIG.stat1_16    \u0001\u0000\u0000\u0000\u0000\u0000\u0000\u0000\u0001\u0000\u0000\u0000\u0000\u0000\u0000\u0000\u0001\u0000\u0000\u0000\u0000\u0000\u0000\u0000\u0000\u0000\u0000\u0000\u0000\u0000\u0000\u0000\u0000\u0000\u0000\u0000ÿÿ\u0000\u0000\u0000\u0000\u0000\u0000", "PMU.060\u0000\u0000\u0000\u0000\u0000\u0000\u0000\u0000\u0000\u0000<\u0000\u000f\u0000\u0006\u0000\u0003\u0000\u0001PZR.AI          PZR.BV          PZR.CI          PZR.AV          PZR.BI          PZR.CV          ANA1            ANA2            ANA3            DIG.stat1_01    DIG.stat1_02    DIG.stat1_03    DIG.stat1_04    DIG.stat1_05    DIG.stat1_06    DIG.stat1_07    DIG.stat1_08    DIG.stat1_09    DIG.stat1_10    DIG.stat1_11    DIG.stat1_12    DIG.stat1_13    DIG.stat1_14    DIG.stat1_15    DIG.stat1_16    \u0001\u0000\u0000\u0000\u0000\u0000\u0000\u0000\u0001\u0000\u0000\u0000\u0000\u0000\u0000\u0000\u0001\u0000\u0000\u0000\u0000\u0000\u0000\u0000\u0000\u0000\u0000\u0000\u0000\u0000\u0000\u0000\u0000\u0000\u0000\u0000ÿÿ\u0000\u0000\u0000\u0000\u0000\u0000", "PMU.061\u0000\u0000\u0000\u0000\u0000\u0000\u0000\u0000\u0000\u0000=\u0000\u000f\u0000\u0006\u0000\u0003\u0000\u0001PZR.AI          PZR.BV          PZR.CI          PZR.AV          PZR.BI          PZR.CV          ANA1            ANA2            ANA3            DIG.stat1_01    DIG.stat1_02    DIG.stat1_03    DIG.stat1_04    DIG.stat1_05    DIG.stat1_06    DIG.stat1_07    DIG.stat1_08    DIG.stat1_09    DIG.stat1_10    DIG.stat1_11    DIG.stat1_12    DIG.stat1_13    DIG.stat1_14    DIG.stat1_15    DIG.stat1_16    \u0001\u0000\u0000\u0000\u0000\u0000\u0000\u0000\u0001\u0000\u0000\u0000\u0000\u0000\u0000\u0000\u0001\u0000\u0000\u0000\u0000\u0000\u0000\u0000\u0000\u0000\u0000\u0000\u0000\u0000\u0000\u0000\u0000\u0000\u0000\u0000ÿÿ\u0000\u0000\u0000\u0000\u0000\u0000", "PMU.062\u0000\u0000\u0000\u0000\u0000\u0000\u0000\u0000\u0000\u0000>\u0000\u000f\u0000\u0006\u0000\u0003\u0000\u0001PZR.AI          PZR.BV          PZR.CI          PZR.AV          PZR.BI          PZR.CV          ANA1            ANA2            ANA3            DIG.stat1_01    DIG.stat1_02    DIG.stat1_03    DIG.stat1_04    DIG.stat1_05    DIG.stat1_06    DIG.stat1_07    DIG.stat1_08    DIG.stat1_09    DIG.stat1_10    DIG.stat1_11    DIG.stat1_12    DIG.stat1_13    DIG.stat1_14    DIG.stat1_15    DIG.stat1_16    \u0001\u0000\u0000\u0000\u0000\u0000\u0000\u0000\u0001\u0000\u0000\u0000\u0000\u0000\u0000\u0000\u0001\u0000\u0000\u0000\u0000\u0000\u0000\u0000\u0000\u0000\u0000\u0000\u0000\u0000\u0000\u0000\u0000\u0000\u0000\u0000ÿÿ\u0000\u0000\u0000\u0000\u0000\u0000", "PMU.063\u0000\u0000\u0000\u0000\u0000\u0000\u0000\u0000\u0000\u0000?\u0000\u000f\u0000\u0006\u0000\u0003\u0000\u0001PZR.AI          PZR.BV          PZR.CI          PZR.AV          PZR.BI          PZR.CV          ANA1            ANA2            ANA3            DIG.stat1_01    DIG.stat1_02    DIG.stat1_03    DIG.stat1_04    DIG.stat1_05    DIG.stat1_06    DIG.stat1_07    DIG.stat1_08    DIG.stat1_09    DIG.stat1_10    DIG.stat1_11    DIG.stat1_12    DIG.stat1_13    DIG.stat1_14    DIG.stat1_15    DIG.stat1_16    \u0001\u0000\u0000\u0000\u0000\u0000\u0000\u0000\u0001\u0000\u0000\u0000\u0000\u0000\u0000\u0000\u0001\u0000\u0000\u0000\u0000\u0000\u0000\u0000\u0000\u0000\u0000\u0000\u0000\u0000\u0000\u0000\u0000\u0000\u0000\u0000ÿÿ\u0000\u0000\u0000\u0000\u0000\u0000", "PMU.064\u0000\u0000\u0000\u0000\u0000\u0000\u0000\u0000\u0000\u0000@\u0000\u000f\u0000\u0006\u0000\u0003\u0000\u0001PZR.AI          PZR.BV          PZR.CI          PZR.AV          PZR.BI          PZR.CV          ANA1            ANA2            ANA3            DIG.stat1_01    DIG.stat1_02    DIG.stat1_03    DIG.stat1_04    DIG.stat1_05    DIG.stat1_06    DIG.stat1_07    DIG.stat1_08    DIG.stat1_09    DIG.stat1_10    DIG.stat1_11    DIG.stat1_12    DIG.stat1_13    DIG.stat1_14    DIG.stat1_15    DIG.stat1_16    \u0001\u0000\u0000\u0000\u0000\u0000\u0000\u0000\u0001\u0000\u0000\u0000\u0000\u0000\u0000\u0000\u0001\u0000\u0000\u0000\u0000\u0000\u0000\u0000\u0000\u0000\u0000\u0000\u0000\u0000\u0000\u0000\u0000\u0000\u0000\u0000ÿÿ\u0000\u0000\u0000\u0000\u0000\u0000", "PMU.065\u0000\u0000\u0000\u0000\u0000\u0000\u0000\u0000\u0000\u0000A\u0000\u000f\u0000\u0006\u0000\u0003\u0000\u0001PZR.AI          PZR.BV          PZR.CI          PZR.AV          PZR.BI          PZR.CV          ANA1            ANA2            ANA3            DIG.stat1_01    DIG.stat1_02    DIG.stat1_03    DIG.stat1_04    DIG.stat1_05    DIG.stat1_06    DIG.stat1_07    DIG.stat1_08    DIG.stat1_09    DIG.stat1_10    DIG.stat1_11    DIG.stat1_12    DIG.stat1_13    DIG.stat1_14    DIG.stat1_15    DIG.stat1_16    \u0001\u0000\u0000\u0000\u0000\u0000\u0000\u0000\u0001\u0000\u0000\u0000\u0000\u0000\u0000\u0000\u0001\u0000\u0000\u0000\u0000\u0000\u0000\u0000\u0000\u0000\u0000\u0000\u0000\u0000\u0000\u0000\u0000\u0000\u0000\u0000ÿÿ\u0000\u0000\u0000\u0000\u0000\u0000", "PMU.066\u0000\u0000\u0000\u0000\u0000\u0000\u0000\u0000\u0000\u0000B\u0000\u000f\u0000\u0006\u0000\u0003\u0000\u0001PZR.AI          PZR.BV          PZR.CI          PZR.AV          PZR.BI          PZR.CV          ANA1            ANA2            ANA3            DIG.stat1_01    DIG.stat1_02    DIG.stat1_03    DIG.stat1_04    DIG.stat1_05    DIG.stat1_06    DIG.stat1_07    DIG.stat1_08    DIG.stat1_09    DIG.stat1_10    DIG.stat1_11    DIG.stat1_12    DIG.stat1_13    DIG.stat1_14    DIG.stat1_15    DIG.stat1_16    \u0001\u0000\u0000\u0000\u0000\u0000\u0000\u0000\u0001\u0000\u0000\u0000\u0000\u0000\u0000\u0000\u0001\u0000\u0000\u0000\u0000\u0000\u0000\u0000\u0000\u0000\u0000\u0000\u0000\u0000\u0000\u0000\u0000\u0000\u0000\u0000ÿÿ\u0000\u0000\u0000\u0000\u0000\u0000", "PMU.067\u0000\u0000\u0000\u0000\u0000\u0000\u0000\u0000\u0000\u0000C\u0000\u000f\u0000\u0006\u0000\u0003\u0000\u0001PZR.AI          PZR.BV          PZR.CI          PZR.AV          PZR.BI          PZR.CV          ANA1            ANA2            ANA3            DIG.stat1_01    DIG.stat1_02    DIG.stat1_03    DIG.stat1_04    DIG.stat1_05    DIG.stat1_06    DIG.stat1_07    DIG.stat1_08    DIG.stat1_09    DIG.stat1_10    DIG.stat1_11    DIG.stat1_12    DIG.stat1_13    DIG.stat1_14    DIG.stat1_15    DIG.stat1_16    \u0001\u0000\u0000\u0000\u0000\u0000\u0000\u0000\u0001\u0000\u0000\u0000\u0000\u0000\u0000\u0000\u0001\u0000\u0000\u0000\u0000\u0000\u0000\u0000\u0000\u0000\u0000\u0000\u0000\u0000\u0000\u0000\u0000\u0000\u0000\u0000ÿÿ\u0000\u0000\u0000\u0000\u0000\u0000", "PMU.068\u0000\u0000\u0000\u0000\u0000\u0000\u0000\u0000\u0000\u0000D\u0000\u000f\u0000\u0006\u0000\u0003\u0000\u0001PZR.AI          PZR.BV          PZR.CI          PZR.AV          PZR.BI          PZR.CV          ANA1            ANA2            ANA3            DIG.stat1_01    DIG.stat1_02    DIG.stat1_03    DIG.stat1_04    DIG.stat1_05    DIG.stat1_06    DIG.stat1_07    DIG.stat1_08    DIG.stat1_09    DIG.stat1_10    DIG.stat1_11    DIG.stat1_12    DIG.stat1_13    DIG.stat1_14    DIG.stat1_15    DIG.stat1_16    \u0001\u0000\u0000\u0000\u0000\u0000\u0000\u0000\u0001\u0000\u0000\u0000\u0000\u0000\u0000\u0000\u0001\u0000\u0000\u0000\u0000\u0000\u0000\u0000\u0000\u0000\u0000\u0000\u0000\u0000\u0000\u0000\u0000\u0000\u0000\u0000ÿÿ\u0000\u0000\u0000\u0000\u0000\u0000", "PMU.069\u0000\u0000\u0000\u0000\u0000\u0000\u0000\u0000\u0000\u0000E\u0000\u000f\u0000\u0006\u0000\u0003\u0000\u0001PZR.AI          PZR.BV          PZR.CI          PZR.AV          PZR.BI          PZR.CV          ANA1            ANA2            ANA3            DIG.stat1_01    DIG.stat1_02    DIG.stat1_03    DIG.stat1_04    DIG.stat1_05    DIG.stat1_06    DIG.stat1_07    DIG.stat1_08    DIG.stat1_09    DIG.stat1_10    DIG.stat1_11    DIG.stat1_12    DIG.stat1_13    DIG.stat1_14    DIG.stat1_15    DIG.stat1_16    \u0001\u0000\u0000\u0000\u0000\u0000\u0000\u0000\u0001\u0000\u0000\u0000\u0000\u0000\u0000\u0000\u0001\u0000\u0000\u0000\u0000\u0000\u0000\u0000\u0000\u0000\u0000\u0000\u0000\u0000\u0000\u0000\u0000\u0000\u0000\u0000ÿÿ\u0000\u0000\u0000\u0000\u0000\u0000", "PMU.070\u0000\u0000\u0000\u0000\u0000\u0000\u0000\u0000\u0000\u0000F\u0000\u000f\u0000\u0006\u0000\u0003\u0000\u0001PZR.AI          PZR.BV          PZR.CI          PZR.AV          PZR.BI          PZR.CV          ANA1            ANA2            ANA3            DIG.stat1_01    DIG.stat1_02    DIG.stat1_03    DIG.stat1_04    DIG.stat1_05    DIG.stat1_06    DIG.stat1_07    DIG.stat1_08    DIG.stat1_09    DIG.stat1_10    DIG.stat1_11    DIG.stat1_12    DIG.stat1_13    DIG.stat1_14    DIG.stat1_15    DIG.stat1_16    \u0001\u0000\u0000\u0000\u0000\u0000\u0000\u0000\u0001\u0000\u0000\u0000\u0000\u0000\u0000\u0000\u0001\u0000\u0000\u0000\u0000\u0000\u0000\u0000\u0000\u0000\u0000\u0000\u0000\u0000\u0000\u0000\u0000\u0000\u0000\u0000ÿÿ\u0000\u0000\u0000\u0000\u0000\u0000", "PMU.071\u0000\u0000\u0000\u0000\u0000\u0000\u0000\u0000\u0000\u0000G\u0000\u000f\u0000\u0006\u0000\u0003\u0000\u0001PZR.AI          PZR.BV          PZR.CI          PZR.AV          PZR.BI          PZR.CV          ANA1            ANA2            ANA3            DIG.stat1_01    DIG.stat1_02    DIG.stat1_03    DIG.stat1_04    DIG.stat1_05    DIG.stat1_06    DIG.stat1_07    DIG.stat1_08    DIG.stat1_09    DIG.stat1_10    DIG.stat1_11    DIG.stat1_12    DIG.stat1_13    DIG.stat1_14    DIG.stat1_15    DIG.stat1_16    \u0001\u0000\u0000\u0000\u0000\u0000\u0000\u0000\u0001\u0000\u0000\u0000\u0000\u0000\u0000\u0000\u0001\u0000\u0000\u0000\u0000\u0000\u0000\u0000\u0000\u0000\u0000\u0000\u0000\u0000\u0000\u0000\u0000\u0000\u0000\u0000ÿÿ\u0000\u0000\u0000\u0000\u0000\u0000", "PMU.072\u0000\u0000\u0000\u0000\u0000\u0000\u0000\u0000\u0000\u0000H\u0000\u000f\u0000\u0006\u0000\u0003\u0000\u0001PZR.AI          PZR.BV          PZR.CI          PZR.AV          PZR.BI          PZR.CV          ANA1            ANA2            ANA3            DIG.stat1_01    DIG.stat1_02    DIG.stat1_03    DIG.stat1_04    DIG.stat1_05    DIG.stat1_06    DIG.stat1_07    DIG.stat1_08    DIG.stat1_09    DIG.stat1_10    DIG.stat1_11    DIG.stat1_12    DIG.stat1_13    DIG.stat1_14    DIG.stat1_15    DIG.stat1_16    \u0001\u0000\u0000\u0000\u0000\u0000\u0000\u0000\u0001\u0000\u0000\u0000\u0000\u0000\u0000\u0000\u0001\u0000\u0000\u0000\u0000\u0000\u0000\u0000\u0000\u0000\u0000\u0000\u0000\u0000\u0000\u0000\u0000\u0000\u0000\u0000ÿÿ\u0000\u0000\u0000\u0000\u0000\u0000", "PMU.073\u0000\u0000\u0000\u0000\u0000\u0000\u0000\u0000\u0000\u0000I\u0000\u000f\u0000\u0006\u0000\u0003\u0000\u0001PZR.AI          PZR.BV          PZR.CI          PZR.AV          PZR.BI          PZR.CV          ANA1            ANA2            ANA3            DIG.stat1_01    DIG.stat1_02    DIG.stat1_03    DIG.stat1_04    DIG.stat1_05    DIG.stat1_06    DIG.stat1_07    DIG.stat1_08    DIG.stat1_09    DIG.stat1_10    DIG.stat1_11    DIG.stat1_12    DIG.stat1_13    DIG.stat1_14    DIG.stat1_15    DIG.stat1_16    \u0001\u0000\u0000\u0000\u0000\u0000\u0000\u0000\u0001\u0000\u0000\u0000\u0000\u0000\u0000\u0000\u0001\u0000\u0000\u0000\u0000\u0000\u0000\u0000\u0000\u0000\u0000\u0000\u0000\u0000\u0000\u0000\u0000\u0000\u0000\u0000ÿÿ\u0000\u0000\u0000\u0000\u0000\u0000", "PMU.074\u0000\u0000\u0000\u0000\u0000\u0000\u0000\u0000\u0000\u0000J\u0000\u000f\u0000\u0006\u0000\u0003\u0000\u0001PZR.AI          PZR.BV          PZR.CI          PZR.AV          PZR.BI          PZR.CV          ANA1            ANA2            ANA3            DIG.stat1_01    DIG.stat1_02    DIG.stat1_03    DIG.stat1_04    DIG.stat1_05    DIG.stat1_06    DIG.stat1_07    DIG.stat1_08    DIG.stat1_09    DIG.stat1_10    DIG.stat1_11    DIG.stat1_12    DIG.stat1_13    DIG.stat1_14    DIG.stat1_15    DIG.stat1_16    \u0001\u0000\u0000\u0000\u0000\u0000\u0000\u0000\u0001\u0000\u0000\u0000\u0000\u0000\u0000\u0000\u0001\u0000\u0000\u0000\u0000\u0000\u0000\u0000\u0000\u0000\u0000\u0000\u0000\u0000\u0000\u0000\u0000\u0000\u0000\u0000ÿÿ\u0000\u0000\u0000\u0000\u0000\u0000", "PMU.075\u0000\u0000\u0000\u0000\u0000\u0000\u0000\u0000\u0000\u0000K\u0000\u000f\u0000\u0006\u0000\u0003\u0000\u0001PZR.AI          PZR.BV          PZR.CI          PZR.AV          PZR.BI          PZR.CV          ANA1            ANA2            ANA3            DIG.stat1_01    DIG.stat1_02    DIG.stat1_03    DIG.stat1_04    DIG.stat1_05    DIG.stat1_06    DIG.stat1_07    DIG.stat1_08    DIG.stat1_09    DIG.stat1_10    DIG.stat1_11    DIG.stat1_12    DIG.stat1_13    DIG.stat1_14    DIG.stat1_15    DIG.stat1_16    \u0001\u0000\u0000\u0000\u0000\u0000\u0000\u0000\u0001\u0000\u0000\u0000\u0000\u0000\u0000\u0000\u0001\u0000\u0000\u0000\u0000\u0000\u0000\u0000\u0000\u0000\u0000\u0000\u0000\u0000\u0000\u0000\u0000\u0000\u0000\u0000ÿÿ\u0000\u0000\u0000\u0000\u0000\u0000", "PMU.076\u0000\u0000\u0000\u0000\u0000\u0000\u0000\u0000\u0000\u0000L\u0000\u000f\u0000\u0006\u0000\u0003\u0000\u0001PZR.AI          PZR.BV          PZR.CI          PZR.AV          PZR.BI          PZR.CV          ANA1            ANA2            ANA3            DIG.stat1_01    DIG.stat1_02    DIG.stat1_03    DIG.stat1_04    DIG.stat1_05    DIG.stat1_06    DIG.stat1_07    DIG.stat1_08    DIG.stat1_09    DIG.stat1_10    DIG.stat1_11    DIG.stat1_12    DIG.stat1_13    DIG.stat1_14    DIG.stat1_15    DIG.stat1_16    \u0001\u0000\u0000\u0000\u0000\u0000\u0000\u0000\u0001\u0000\u0000\u0000\u0000\u0000\u0000\u0000\u0001\u0000\u0000\u0000\u0000\u0000\u0000\u0000\u0000\u0000\u0000\u0000\u0000\u0000\u0000\u0000\u0000\u0000\u0000\u0000ÿÿ\u0000\u0000\u0000\u0000\u0000\u0000", "PMU.077\u0000\u0000\u0000\u0000\u0000\u0000\u0000\u0000\u0000\u0000M\u0000\u000f\u0000\u0006\u0000\u0003\u0000\u0001PZR.AI          PZR.BV          PZR.CI          PZR.AV          PZR.BI          PZR.CV          ANA1            ANA2            ANA3            DIG.stat1_01    DIG.stat1_02    DIG.stat1_03    DIG.stat1_04    DIG.stat1_05    DIG.stat1_06    DIG.stat1_07    DIG.stat1_08    DIG.stat1_09    DIG.stat1_10    DIG.stat1_11    DIG.stat1_12    DIG.stat1_13    DIG.stat1_14    DIG.stat1_15    DIG.stat1_16    \u0001\u0000\u0000\u0000\u0000\u0000\u0000\u0000\u0001\u0000\u0000\u0000\u0000\u0000\u0000\u0000\u0001\u0000\u0000\u0000\u0000\u0000\u0000\u0000\u0000\u0000\u0000\u0000\u0000\u0000\u0000\u0000\u0000\u0000\u0000\u0000ÿÿ\u0000\u0000\u0000\u0000\u0000\u0000", "PMU.078\u0000\u0000\u0000\u0000\u0000\u0000\u0000\u0000\u0000\u0000N\u0000\u000f\u0000\u0006\u0000\u0003\u0000\u0001PZR.AI          PZR.BV          PZR.CI          PZR.AV          PZR.BI          PZR.CV          ANA1            ANA2            ANA3            DIG.stat1_01    DIG.stat1_02    DIG.stat1_03    DIG.stat1_04    DIG.stat1_05    DIG.stat1_06    DIG.stat1_07    DIG.stat1_08    DIG.stat1_09    DIG.stat1_10    DIG.stat1_11    DIG.stat1_12    DIG.stat1_13    DIG.stat1_14    DIG.stat1_15    DIG.stat1_16    \u0001\u0000\u0000\u0000\u0000\u0000\u0000\u0000\u0001\u0000\u0000\u0000\u0000\u0000\u0000\u0000\u0001\u0000\u0000\u0000\u0000\u0000\u0000\u0000\u0000\u0000\u0000\u0000\u0000\u0000\u0000\u0000\u0000\u0000\u0000\u0000ÿÿ\u0000\u0000\u0000\u0000\u0000\u0000", "PMU.079\u0000\u0000\u0000\u0000\u0000\u0000\u0000\u0000\u0000\u0000O\u0000\u000f\u0000\u0006\u0000\u0003\u0000\u0001PZR.AI          PZR.BV          PZR.CI          PZR.AV          PZR.BI          PZR.CV          ANA1            ANA2            ANA3            DIG.stat1_01    DIG.stat1_02    DIG.stat1_03    DIG.stat1_04    DIG.stat1_05    DIG.stat1_06    DIG.stat1_07    DIG.stat1_08    DIG.stat1_09    DIG.stat1_10    DIG.stat1_11    DIG.stat1_12    DIG.stat1_13    DIG.stat1_14    DIG.stat1_15    DIG.stat1_16    \u0001\u0000\u0000\u0000\u0000\u0000\u0000\u0000\u0001\u0000\u0000\u0000\u0000\u0000\u0000\u0000\u0001\u0000\u0000\u0000\u0000\u0000\u0000\u0000\u0000\u0000\u0000\u0000\u0000\u0000\u0000\u0000\u0000\u0000\u0000\u0000ÿÿ\u0000\u0000\u0000\u0000\u0000\u0000", "PMU.080\u0000\u0000\u0000\u0000\u0000\u0000\u0000\u0000\u0000\u0000P\u0000\u000f\u0000\u0006\u0000\u0003\u0000\u0001PZR.AI          PZR.BV          PZR.CI          PZR.AV          PZR.BI          PZR.CV          ANA1            ANA2            ANA3            DIG.stat1_01    DIG.stat1_02    DIG.stat1_03    DIG.stat1_04    DIG.stat1_05    DIG.stat1_06    DIG.stat1_07    DIG.stat1_08    DIG.stat1_09    DIG.stat1_10    DIG.stat1_11    DIG.stat1_12    DIG.stat1_13    DIG.stat1_14    DIG.stat1_15    DIG.stat1_16    \u0001\u0000\u0000\u0000\u0000\u0000\u0000\u0000\u0001\u0000\u0000\u0000\u0000\u0000\u0000\u0000\u0001\u0000\u0000\u0000\u0000\u0000\u0000\u0000\u0000\u0000\u0000\u0000\u0000\u0000\u0000\u0000\u0000\u0000\u0000\u0000ÿÿ\u0000\u0000\u0000\u0000\u0000\u0000", "PMU.081\u0000\u0000\u0000\u0000\u0000\u0000\u0000\u0000\u0000\u0000Q\u0000\u000f\u0000\u0006\u0000\u0003\u0000\u0001PZR.AI          PZR.BV          PZR.CI          PZR.AV          PZR.BI          PZR.CV          ANA1            ANA2            ANA3            DIG.stat1_01    DIG.stat1_02    DIG.stat1_03    DIG.stat1_04    DIG.stat1_05    DIG.stat1_06    DIG.stat1_07    DIG.stat1_08    DIG.stat1_09    DIG.stat1_10    DIG.stat1_11    DIG.stat1_12    DIG.stat1_13    DIG.stat1_14    DIG.stat1_15    DIG.stat1_16    \u0001\u0000\u0000\u0000\u0000\u0000\u0000\u0000\u0001\u0000\u0000\u0000\u0000\u0000\u0000\u0000\u0001\u0000\u0000\u0000\u0000\u0000\u0000\u0000\u0000\u0000\u0000\u0000\u0000\u0000\u0000\u0000\u0000\u0000\u0000\u0000ÿÿ\u0000\u0000\u0000\u0000\u0000\u0000", "PMU.082\u0000\u0000\u0000\u0000\u0000\u0000\u0000\u0000\u0000\u0000R\u0000\u000f\u0000\u0006\u0000\u0003\u0000\u0001PZR.AI          PZR.BV          PZR.CI          PZR.AV          PZR.BI          PZR.CV          ANA1            ANA2            ANA3            DIG.stat1_01    DIG.stat1_02    DIG.stat1_03    DIG.stat1_04    DIG.stat1_05    DIG.stat1_06    DIG.stat1_07    DIG.stat1_08    DIG.stat1_09    DIG.stat1_10    DIG.stat1_11    DIG.stat1_12    DIG.stat1_13    DIG.stat1_14    DIG.stat1_15    DIG.stat1_16    \u0001\u0000\u0000\u0000\u0000\u0000\u0000\u0000\u0001\u0000\u0000\u0000\u0000\u0000\u0000\u0000\u0001\u0000\u0000\u0000\u0000\u0000\u0000\u0000\u0000\u0000\u0000\u0000\u0000\u0000\u0000\u0000\u0000\u0000\u0000\u0000ÿÿ\u0000\u0000\u0000\u0000\u0000\u0000", "PMU.083\u0000\u0000\u0000\u0000\u0000\u0000\u0000\u0000\u0000\u0000S\u0000\u000f\u0000\u0006\u0000\u0003\u0000\u0001PZR.AI          PZR.BV          PZR.CI          PZR.AV          PZR.BI          PZR.CV          ANA1            ANA2            ANA3            DIG.stat1_01    DIG.stat1_02    DIG.stat1_03    DIG.stat1_04    DIG.stat1_05    DIG.stat1_06    DIG.stat1_07    DIG.stat1_08    DIG.stat1_09    DIG.stat1_10    DIG.stat1_11    DIG.stat1_12    DIG.stat1_13    DIG.stat1_14    DIG.stat1_15    DIG.stat1_16    \u0001\u0000\u0000\u0000\u0000\u0000\u0000\u0000\u0001\u0000\u0000\u0000\u0000\u0000\u0000\u0000\u0001\u0000\u0000\u0000\u0000\u0000\u0000\u0000\u0000\u0000\u0000\u0000\u0000\u0000\u0000\u0000\u0000\u0000\u0000\u0000ÿÿ\u0000\u0000\u0000\u0000\u0000\u0000", "PMU.084\u0000\u0000\u0000\u0000\u0000\u0000\u0000\u0000\u0000\u0000T\u0000\u000f\u0000\u0006\u0000\u0003\u0000\u0001PZR.AI          PZR.BV          PZR.CI          PZR.AV          PZR.BI          PZR.CV          ANA1            ANA2            ANA3            DIG.stat1_01    DIG.stat1_02    DIG.stat1_03    DIG.stat1_04    DIG.stat1_05    DIG.stat1_06    DIG.stat1_07    DIG.stat1_08    DIG.stat1_09    DIG.stat1_10    DIG.stat1_11    DIG.stat1_12    DIG.stat1_13    DIG.stat1_14    DIG.stat1_15    DIG.stat1_16    \u0001\u0000\u0000\u0000\u0000\u0000\u0000\u0000\u0001\u0000\u0000\u0000\u0000\u0000\u0000\u0000\u0001\u0000\u0000\u0000\u0000\u0000\u0000\u0000\u0000\u0000\u0000\u0000\u0000\u0000\u0000\u0000\u0000\u0000\u0000\u0000ÿÿ\u0000\u0000\u0000\u0000\u0000\u0000", "PMU.085\u0000\u0000\u0000\u0000\u0000\u0000\u0000\u0000\u0000\u0000U\u0000\u000f\u0000\u0006\u0000\u0003\u0000\u0001PZR.AI          PZR.BV          PZR.CI          PZR.AV          PZR.BI          PZR.CV          ANA1            ANA2            ANA3            DIG.stat1_01    DIG.stat1_02    DIG.stat1_03    DIG.stat1_04    DIG.stat1_05    DIG.stat1_06    DIG.stat1_07    DIG.stat1_08    DIG.stat1_09    DIG.stat1_10    DIG.stat1_11    DIG.stat1_12    DIG.stat1_13    DIG.stat1_14    DIG.stat1_15    DIG.stat1_16    \u0001\u0000\u0000\u0000\u0000\u0000\u0000\u0000\u0001\u0000\u0000\u0000\u0000\u0000\u0000\u0000\u0001\u0000\u0000\u0000\u0000\u0000\u0000\u0000\u0000\u0000\u0000\u0000\u0000\u0000\u0000\u0000\u0000\u0000\u0000\u0000ÿÿ\u0000\u0000\u0000\u0000\u0000\u0000", "PMU.086\u0000\u0000\u0000\u0000\u0000\u0000\u0000\u0000\u0000\u0000V\u0000\u000f\u0000\u0006\u0000\u0003\u0000\u0001PZR.AI          PZR.BV          PZR.CI          PZR.AV          PZR.BI          PZR.CV          ANA1            ANA2            ANA3            DIG.stat1_01    DIG.stat1_02    DIG.stat1_03    DIG.stat1_04    DIG.stat1_05    DIG.stat1_06    DIG.stat1_07    DIG.stat1_08    DIG.stat1_09    DIG.stat1_10    DIG.stat1_11    DIG.stat1_12    DIG.stat1_13    DIG.stat1_14    DIG.stat1_15    DIG.stat1_16    \u0001\u0000\u0000\u0000\u0000\u0000\u0000\u0000\u0001\u0000\u0000\u0000\u0000\u0000\u0000\u0000\u0001\u0000\u0000\u0000\u0000\u0000\u0000\u0000\u0000\u0000\u0000\u0000\u0000\u0000\u0000\u0000\u0000\u0000\u0000\u0000ÿÿ\u0000\u0000\u0000\u0000\u0000\u0000", "PMU.087\u0000\u0000\u0000\u0000\u0000\u0000\u0000\u0000\u0000\u0000W\u0000\u000f\u0000\u0006\u0000\u0003\u0000\u0001PZR.AI          PZR.BV          PZR.CI          PZR.AV          PZR.BI          PZR.CV          ANA1            ANA2            ANA3            DIG.stat1_01    DIG.stat1_02    DIG.stat1_03    DIG.stat1_04    DIG.stat1_05    DIG.stat1_06    DIG.stat1_07    DIG.stat1_08    DIG.stat1_09    DIG.stat1_10    DIG.stat1_11    DIG.stat1_12    DIG.stat1_13    DIG.stat1_14    DIG.stat1_15    DIG.stat1_16    \u0001\u0000\u0000\u0000\u0000\u0000\u0000\u0000\u0001\u0000\u0000\u0000\u0000\u0000\u0000\u0000\u0001\u0000\u0000\u0000\u0000\u0000\u0000\u0000\u0000\u0000\u0000\u0000\u0000\u0000\u0000\u0000\u0000\u0000\u0000\u0000ÿÿ\u0000\u0000\u0000\u0000\u0000\u0000", "PMU.088\u0000\u0000\u0000\u0000\u0000\u0000\u0000\u0000\u0000\u0000X\u0000\u000f\u0000\u0006\u0000\u0003\u0000\u0001PZR.AI          PZR.BV          PZR.CI          PZR.AV          PZR.BI          PZR.CV          ANA1            ANA2            ANA3            DIG.stat1_01    DIG.stat1_02    DIG.stat1_03    DIG.stat1_04    DIG.stat1_05    DIG.stat1_06    DIG.stat1_07    DIG.stat1_08    DIG.stat1_09    DIG.stat1_10    DIG.stat1_11    DIG.stat1_12    DIG.stat1_13    DIG.stat1_14    DIG.stat1_15    DIG.stat1_16    \u0001\u0000\u0000\u0000\u0000\u0000\u0000\u0000\u0001\u0000\u0000\u0000\u0000\u0000\u0000\u0000\u0001\u0000\u0000\u0000\u0000\u0000\u0000\u0000\u0000\u0000\u0000\u0000\u0000\u0000\u0000\u0000\u0000\u0000\u0000\u0000ÿÿ\u0000\u0000\u0000\u0000\u0000\u0000", "PMU.089\u0000\u0000\u0000\u0000\u0000\u0000\u0000\u0000\u0000\u0000Y\u0000\u000f\u0000\u0006\u0000\u0003\u0000\u0001PZR.AI          PZR.BV          PZR.CI          PZR.AV          PZR.BI          PZR.CV          ANA1            ANA2            ANA3            DIG.stat1_01    DIG.stat1_02    DIG.stat1_03    DIG.stat1_04    DIG.stat1_05    DIG.stat1_06    DIG.stat1_07    DIG.stat1_08    DIG.stat1_09    DIG.stat1_10    DIG.stat1_11    DIG.stat1_12    DIG.stat1_13    DIG.stat1_14    DIG.stat1_15    DIG.stat1_16    \u0001\u0000\u0000\u0000\u0000\u0000\u0000\u0000\u0001\u0000\u0000\u0000\u0000\u0000\u0000\u0000\u0001\u0000\u0000\u0000\u0000\u0000\u0000\u0000\u0000\u0000\u0000\u0000\u0000\u0000\u0000\u0000\u0000\u0000\u0000\u0000ÿÿ\u0000\u0000\u0000\u0000\u0000\u0000", "PMU.090\u0000\u0000\u0000\u0000\u0000\u0000\u0000\u0000\u0000\u0000Z\u0000\u000f\u0000\u0006\u0000\u0003\u0000\u0001PZR.AI          PZR.BV          PZR.CI          PZR.AV          PZR.BI          PZR.CV          ANA1            ANA2            ANA3            DIG.stat1_01    DIG.stat1_02    DIG.stat1_03    DIG.stat1_04    DIG.stat1_05    DIG.stat1_06    DIG.stat1_07    DIG.stat1_08    DIG.stat1_09    DIG.stat1_10    DIG.stat1_11    DIG.stat1_12    DIG.stat1_13    DIG.stat1_14    DIG.stat1_15    DIG.stat1_16    \u0001\u0000\u0000\u0000\u0000\u0000\u0000\u0000\u0001\u0000\u0000\u0000\u0000\u0000\u0000\u0000\u0001\u0000\u0000\u0000\u0000\u0000\u0000\u0000\u0000\u0000\u0000\u0000\u0000\u0000\u0000\u0000\u0000\u0000\u0000\u0000ÿÿ\u0000\u0000\u0000\u0000\u0000\u0000", "PMU.091\u0000\u0000\u0000\u0000\u0000\u0000\u0000\u0000\u0000\u0000[\u0000\u000f\u0000\u0006\u0000\u0003\u0000\u0001PZR.AI          PZR.BV          PZR.CI          PZR.AV          PZR.BI          PZR.CV          ANA1            ANA2            ANA3            DIG.stat1_01    DIG.stat1_02    DIG.stat1_03    DIG.stat1_04    DIG.stat1_05    DIG.stat1_06    DIG.stat1_07    DIG.stat1_08    DIG.stat1_09    DIG.stat1_10    DIG.stat1_11    DIG.stat1_12    DIG.stat1_13    DIG.stat1_14    DIG.stat1_15    DIG.stat1_16    \u0001\u0000\u0000\u0000\u0000\u0000\u0000\u0000\u0001\u0000\u0000\u0000\u0000\u0000\u0000\u0000\u0001\u0000\u0000\u0000\u0000\u0000\u0000\u0000\u0000\u0000\u0000\u0000\u0000\u0000\u0000\u0000\u0000\u0000\u0000\u0000ÿÿ\u0000\u0000\u0000\u0000\u0000\u0000", "PMU.092\u0000\u0000\u0000\u0000\u0000\u0000\u0000\u0000\u0000\u0000\\\u0000\u000f\u0000\u0006\u0000\u0003\u0000\u0001PZR.AI          PZR.BV          PZR.CI          PZR.AV          PZR.BI          PZR.CV          ANA1            ANA2            ANA3            DIG.stat1_01    DIG.stat1_02    DIG.stat1_03    DIG.stat1_04    DIG.stat1_05    DIG.stat1_06    DIG.stat1_07    DIG.stat1_08    DIG.stat1_09    DIG.stat1_10    DIG.stat1_11    DIG.stat1_12    DIG.stat1_13    DIG.stat1_14    DIG.stat1_15    DIG.stat1_16    \u0001\u0000\u0000\u0000\u0000\u0000\u0000\u0000\u0001\u0000\u0000\u0000\u0000\u0000\u0000\u0000\u0001\u0000\u0000\u0000\u0000\u0000\u0000\u0000\u0000\u0000\u0000\u0000\u0000\u0000\u0000\u0000\u0000\u0000\u0000\u0000ÿÿ\u0000\u0000\u0000\u0000\u0000\u0000", "PMU.093\u0000\u0000\u0000\u0000\u0000\u0000\u0000\u0000\u0000\u0000]\u0000\u000f\u0000\u0006\u0000\u0003\u0000\u0001PZR.AI          PZR.BV          PZR.CI          PZR.AV          PZR.BI          PZR.CV          ANA1            ANA2            ANA3            DIG.stat1_01    DIG.stat1_02    DIG.stat1_03    DIG.stat1_04    DIG.stat1_05    DIG.stat1_06    DIG.stat1_07    DIG.stat1_08    DIG.stat1_09    DIG.stat1_10    DIG.stat1_11    DIG.stat1_12    DIG.stat1_13    DIG.stat1_14    DIG.stat1_15    DIG.stat1_16    \u0001\u0000\u0000\u0000\u0000\u0000\u0000\u0000\u0001\u0000\u0000\u0000\u0000\u0000\u0000\u0000\u0001\u0000\u0000\u0000\u0000\u0000\u0000\u0000\u0000\u0000\u0000\u0000\u0000\u0000\u0000\u0000\u0000\u0000\u0000\u0000ÿÿ\u0000\u0000\u0000\u0000\u0000\u0000", "PMU.094\u0000\u0000\u0000\u0000\u0000\u0000\u0000\u0000\u0000\u0000^\u0000\u000f\u0000\u0006\u0000\u0003\u0000\u0001PZR.AI          PZR.BV          PZR.CI          PZR.AV          PZR.BI          PZR.CV          ANA1            ANA2            ANA3            DIG.stat1_01    DIG.stat1_02    DIG.stat1_03    DIG.stat1_04    DIG.stat1_05    DIG.stat1_06    DIG.stat1_07    DIG.stat1_08    DIG.stat1_09    DIG.stat1_10    DIG.stat1_11    DIG.stat1_12    DIG.stat1_13    DIG.stat1_14    DIG.stat1_15    DIG.stat1_16    \u0001\u0000\u0000\u0000\u0000\u0000\u0000\u0000\u0001\u0000\u0000\u0000\u0000\u0000\u0000\u0000\u0001\u0000\u0000\u0000\u0000\u0000\u0000\u0000\u0000\u0000\u0000\u0000\u0000\u0000\u0000\u0000\u0000\u0000\u0000\u0000ÿÿ\u0000\u0000\u0000\u0000\u0000\u0000", "PMU.095\u0000\u0000\u0000\u0000\u0000\u0000\u0000\u0000\u0000\u0000_\u0000\u000f\u0000\u0006\u0000\u0003\u0000\u0001PZR.AI          PZR.BV          PZR.CI          PZR.AV          PZR.BI          PZR.CV          ANA1            ANA2            ANA3            DIG.stat1_01    DIG.stat1_02    DIG.stat1_03    DIG.stat1_04    DIG.stat1_05    DIG.stat1_06    DIG.stat1_07    DIG.stat1_08    DIG.stat1_09    DIG.stat1_10    DIG.stat1_11    DIG.stat1_12    DIG.stat1_13    DIG.stat1_14    DIG.stat1_15    DIG.stat1_16    \u0001\u0000\u0000\u0000\u0000\u0000\u0000\u0000\u0001\u0000\u0000\u0000\u0000\u0000\u0000\u0000\u0001\u0000\u0000\u0000\u0000\u0000\u0000\u0000\u0000\u0000\u0000\u0000\u0000\u0000\u0000\u0000\u0000\u0000\u0000\u0000ÿÿ\u0000\u0000\u0000\u0000\u0000\u0000", "PMU.096\u0000\u0000\u0000\u0000\u0000\u0000\u0000\u0000\u0000\u0000`\u0000\u000f\u0000\u0006\u0000\u0003\u0000\u0001PZR.AI          PZR.BV          PZR.CI          PZR.AV          PZR.BI          PZR.CV          ANA1            ANA2            ANA3            DIG.stat1_01    DIG.stat1_02    DIG.stat1_03    DIG.stat1_04    DIG.stat1_05    DIG.stat1_06    DIG.stat1_07    DIG.stat1_08    DIG.stat1_09    DIG.stat1_10    DIG.stat1_11    DIG.stat1_12    DIG.stat1_13    DIG.stat1_14    DIG.stat1_15    DIG.stat1_16    \u0001\u0000\u0000\u0000\u0000\u0000\u0000\u0000\u0001\u0000\u0000\u0000\u0000\u0000\u0000\u0000\u0001\u0000\u0000\u0000\u0000\u0000\u0000\u0000\u0000\u0000\u0000\u0000\u0000\u0000\u0000\u0000\u0000\u0000\u0000\u0000ÿÿ\u0000\u0000\u0000\u0000\u0000\u0000", "PMU.097\u0000\u0000\u0000\u0000\u0000\u0000\u0000\u0000\u0000\u0000a\u0000\u000f\u0000\u0006\u0000\u0003\u0000\u0001PZR.AI          PZR.BV          PZR.CI          PZR.AV          PZR.BI          PZR.CV          ANA1            ANA2            ANA3            DIG.stat1_01    DIG.stat1_02    DIG.stat1_03    DIG.stat1_04    DIG.stat1_05    DIG.stat1_06    DIG.stat1_07    DIG.stat1_08    DIG.stat1_09    DIG.stat1_10    DIG.stat1_11    DIG.stat1_12    DIG.stat1_13    DIG.stat1_14    DIG.stat1_15    DIG.stat1_16    \u0001\u0000\u0000\u0000\u0000\u0000\u0000\u0000\u0001\u0000\u0000\u0000\u0000\u0000\u0000\u0000\u0001\u0000\u0000\u0000\u0000\u0000\u0000\u0000\u0000\u0000\u0000\u0000\u0000\u0000\u0000\u0000\u0000\u0000\u0000\u0000ÿÿ\u0000\u0000\u0000\u0000\u0000\u0000", "PMU.098\u0000\u0000\u0000\u0000\u0000\u0000\u0000\u0000\u0000\u0000b\u0000\u000f\u0000\u0006\u0000\u0003\u0000\u0001PZR.AI          PZR.BV          PZR.CI          PZR.AV          PZR.BI          PZR.CV          ANA1            ANA2            ANA3            DIG.stat1_01    DIG.stat1_02    DIG.stat1_03    DIG.stat1_04    DIG.stat1_05    DIG.stat1_06    DIG.stat1_07    DIG.stat1_08    DIG.stat1_09    DIG.stat1_10    DIG.stat1_11    DIG.stat1_12    DIG.stat1_13    DIG.stat1_14    DIG.stat1_15    DIG.stat1_16    \u0001\u0000\u0000\u0000\u0000\u0000\u0000\u0000\u0001\u0000\u0000\u0000\u0000\u0000\u0000\u0000\u0001\u0000\u0000\u0000\u0000\u0000\u0000\u0000\u0000\u0000\u0000\u0000\u0000\u0000\u0000\u0000\u0000\u0000\u0000\u0000ÿÿ\u0000\u0000\u0000\u0000\u0000\u0000", "PMU.099\u0000\u0000\u0000\u0000\u0000\u0000\u0000\u0000\u0000\u0000c\u0000\u000f\u0000\u0006\u0000\u0003\u0000\u0001PZR.AI          PZR.BV          PZR.CI          PZR.AV          PZR.BI          PZR.CV          ANA1            ANA2            ANA3            DIG.stat1_01    DIG.stat1_02    DIG.stat1_03    DIG.stat1_04    DIG.stat1_05    DIG.stat1_06    DIG.stat1_07    DIG.stat1_08    DIG.stat1_09    DIG.stat1_10    DIG.stat1_11    DIG.stat1_12    DIG.stat1_13    DIG.stat1_14    DIG.stat1_15    DIG.stat1_16    \u0001\u0000\u0000\u0000\u0000\u0000\u0000\u0000\u0001\u0000\u0000\u0000\u0000\u0000\u0000\u0000\u0001\u0000\u0000\u0000\u0000\u0000\u0000\u0000\u0000\u0000\u0000\u0000\u0000\u0000\u0000\u0000\u0000\u0000\u0000\u0000ÿÿ\u0000\u0000\u0000\u0000\u0000\u0000", "PMU.100\u0000\u0000\u0000\u0000\u0000\u0000\u0000\u0000\u0000\u0000d\u0000\u000f\u0000\u0006\u0000\u0003\u0000\u0001PZR.AI          PZR.BV          PZR.CI          PZR.AV          PZR.BI          PZR.CV          ANA1            ANA2            ANA3            DIG.stat1_01    DIG.stat1_02    DIG.stat1_03    DIG.stat1_04    DIG.stat1_05    DIG.stat1_06    DIG.stat1_07    DIG.stat1_08    DIG.stat1_09    DIG.stat1_10    DIG.stat1_11    DIG.stat1_12    DIG.stat1_13    DIG.stat1_14    DIG.stat1_15    DIG.stat1_16    \u0001\u0000\u0000\u0000\u0000\u0000\u0000\u0000\u0001\u0000\u0000\u0000\u0000\u0000\u0000\u0000\u0001\u0000\u0000\u0000\u0000\u0000\u0000\u0000\u0000\u0000\u0000\u0000\u0000\u0000\u0000\u0000\u0000\u0000\u0000\u0000ÿÿ\u0000\u0000\u0000\u0000\u0000\u0000", "PMU.101\u0000\u0000\u0000\u0000\u0000\u0000\u0000\u0000\u0000\u0000e\u0000\u000f\u0000\u0006\u0000\u0003\u0000\u0001PZR.AI          PZR.BV          PZR.CI          PZR.AV          PZR.BI          PZR.CV          ANA1            ANA2            ANA3            DIG.stat1_01    DIG.stat1_02    DIG.stat1_03    DIG.stat1_04    DIG.stat1_05    DIG.stat1_06    DIG.stat1_07    DIG.stat1_08    DIG.stat1_09    DIG.stat1_10    DIG.stat1_11    DIG.stat1_12    DIG.stat1_13    DIG.stat1_14    DIG.stat1_15    DIG.stat1_16    \u0001\u0000\u0000\u0000\u0000\u0000\u0000\u0000\u0001\u0000\u0000\u0000\u0000\u0000\u0000\u0000\u0001\u0000\u0000\u0000\u0000\u0000\u0000\u0000\u0000\u0000\u0000\u0000\u0000\u0000\u0000\u0000\u0000\u0000\u0000\u0000ÿÿ\u0000\u0000\u0000\u0000\u0000\u0000", "PMU.102\u0000\u0000\u0000\u0000\u0000\u0000\u0000\u0000\u0000\u0000f\u0000\u000f\u0000\u0006\u0000\u0003\u0000\u0001PZR.AI          PZR.BV          PZR.CI          PZR.AV          PZR.BI          PZR.CV          ANA1            ANA2            ANA3            DIG.stat1_01    DIG.stat1_02    DIG.stat1_03    DIG.stat1_04    DIG.stat1_05    DIG.stat1_06    DIG.stat1_07    DIG.stat1_08    DIG.stat1_09    DIG.stat1_10    DIG.stat1_11    DIG.stat1_12    DIG.stat1_13    DIG.stat1_14    DIG.stat1_15    DIG.stat1_16    \u0001\u0000\u0000\u0000\u0000\u0000\u0000\u0000\u0001\u0000\u0000\u0000\u0000\u0000\u0000\u0000\u0001\u0000\u0000\u0000\u0000\u0000\u0000\u0000\u0000\u0000\u0000\u0000\u0000\u0000\u0000\u0000\u0000\u0000\u0000\u0000ÿÿ\u0000\u0000\u0000\u0000\u0000\u0000", "PMU.103\u0000\u0000\u0000\u0000\u0000\u0000\u0000\u0000\u0000\u0000g\u0000\u000f\u0000\u0006\u0000\u0003\u0000\u0001PZR.AI          PZR.BV          PZR.CI          PZR.AV          PZR.BI          PZR.CV          ANA1            ANA2            ANA3            DIG.stat1_01    DIG.stat1_02    DIG.stat1_03    DIG.stat1_04    DIG.stat1_05    DIG.stat1_06    DIG.stat1_07    DIG.stat1_08    DIG.stat1_09    DIG.stat1_10    DIG.stat1_11    DIG.stat1_12    DIG.stat1_13    DIG.stat1_14    DIG.stat1_15    DIG.stat1_16    \u0001\u0000\u0000\u0000\u0000\u0000\u0000\u0000\u0001\u0000\u0000\u0000\u0000\u0000\u0000\u0000\u0001\u0000\u0000\u0000\u0000\u0000\u0000\u0000\u0000\u0000\u0000\u0000\u0000\u0000\u0000\u0000\u0000\u0000\u0000\u0000ÿÿ\u0000\u0000\u0000\u0000\u0000\u0000", "PMU.104\u0000\u0000\u0000\u0000\u0000\u0000\u0000\u0000\u0000\u0000h\u0000\u000f\u0000\u0006\u0000\u0003\u0000\u0001PZR.AI          PZR.BV          PZR.CI          PZR.AV          PZR.BI          PZR.CV          ANA1            ANA2            ANA3            DIG.stat1_01    DIG.stat1_02    DIG.stat1_03    DIG.stat1_04    DIG.stat1_05    DIG.stat1_06    DIG.stat1_07    DIG.stat1_08    DIG.stat1_09    DIG.stat1_10    DIG.stat1_11    DIG.stat1_12    DIG.stat1_13    DIG.stat1_14    DIG.stat1_15    DIG.stat1_16    \u0001\u0000\u0000\u0000\u0000\u0000\u0000\u0000\u0001\u0000\u0000\u0000\u0000\u0000\u0000\u0000\u0001\u0000\u0000\u0000\u0000\u0000\u0000\u0000\u0000\u0000\u0000\u0000\u0000\u0000\u0000\u0000\u0000\u0000\u0000\u0000ÿÿ\u0000\u0000\u0000\u0000\u0000\u0000", "PMU.105\u0000\u0000\u0000\u0000\u0000\u0000\u0000\u0000\u0000\u0000i\u0000\u000f\u0000\u0006\u0000\u0003\u0000\u0001PZR.AI          PZR.BV          PZR.CI          PZR.AV          PZR.BI          PZR.CV          ANA1            ANA2            ANA3            DIG.stat1_01    DIG.stat1_02    DIG.stat1_03    DIG.stat1_04    DIG.stat1_05    DIG.stat1_06    DIG.stat1_07    DIG.stat1_08    DIG.stat1_09    DIG.stat1_10    DIG.stat1_11    DIG.stat1_12    DIG.stat1_13    DIG.stat1_14    DIG.stat1_15    DIG.stat1_16    \u0001\u0000\u0000\u0000\u0000\u0000\u0000\u0000\u0001\u0000\u0000\u0000\u0000\u0000\u0000\u0000\u0001\u0000\u0000\u0000\u0000\u0000\u0000\u0000\u0000\u0000\u0000\u0000\u0000\u0000\u0000\u0000\u0000\u0000\u0000\u0000ÿÿ\u0000\u0000\u0000\u0000\u0000\u0000", "PMU.106\u0000\u0000\u0000\u0000\u0000\u0000\u0000\u0000\u0000\u0000j\u0000\u000f\u0000\u0006\u0000\u0003\u0000\u0001PZR.AI          PZR.BV          PZR.CI          PZR.AV          PZR.BI          PZR.CV          ANA1            ANA2            ANA3            DIG.stat1_01    DIG.stat1_02    DIG.stat1_03    DIG.stat1_04    DIG.stat1_05    DIG.stat1_06    DIG.stat1_07    DIG.stat1_08    DIG.stat1_09    DIG.stat1_10    DIG.stat1_11    DIG.stat1_12    DIG.stat1_13    DIG.stat1_14    DIG.stat1_15    DIG.stat1_16    \u0001\u0000\u0000\u0000\u0000\u0000\u0000\u0000\u0001\u0000\u0000\u0000\u0000\u0000\u0000\u0000\u0001\u0000\u0000\u0000\u0000\u0000\u0000\u0000\u0000\u0000\u0000\u0000\u0000\u0000\u0000\u0000\u0000\u0000\u0000\u0000ÿÿ\u0000\u0000\u0000\u0000\u0000\u0000", "PMU.107\u0000\u0000\u0000\u0000\u0000\u0000\u0000\u0000\u0000\u0000k\u0000\u000f\u0000\u0006\u0000\u0003\u0000\u0001PZR.AI          PZR.BV          PZR.CI          PZR.AV          PZR.BI          PZR.CV          ANA1            ANA2            ANA3            DIG.stat1_01    DIG.stat1_02    DIG.stat1_03    DIG.stat1_04    DIG.stat1_05    DIG.stat1_06    DIG.stat1_07    DIG.stat1_08    DIG.stat1_09    DIG.stat1_10    DIG.stat1_11    DIG.stat1_12    DIG.stat1_13    DIG.stat1_14    DIG.stat1_15    DIG.stat1_16    \u0001\u0000\u0000\u0000\u0000\u0000\u0000\u0000\u0001\u0000\u0000\u0000\u0000\u0000\u0000\u0000\u0001\u0000\u0000\u0000\u0000\u0000\u0000\u0000\u0000\u0000\u0000\u0000\u0000\u0000\u0000\u0000\u0000\u0000\u0000\u0000ÿÿ\u0000\u0000\u0000\u0000\u0000\u0000", "PMU.108\u0000\u0000\u0000\u0000\u0000\u0000\u0000\u0000\u0000\u0000l\u0000\u000f\u0000\u0006\u0000\u0003\u0000\u0001PZR.AI          PZR.BV          PZR.CI          PZR.AV          PZR.BI          PZR.CV          ANA1            ANA2            ANA3            DIG.stat1_01    DIG.stat1_02    DIG.stat1_03    DIG.stat1_04    DIG.stat1_05    DIG.stat1_06    DIG.stat1_07    DIG.stat1_08    DIG.stat1_09    DIG.stat1_10    DIG.stat1_11    DIG.stat1_12    DIG.stat1_13    DIG.stat1_14    DIG.stat1_15    DIG.stat1_16    \u0001\u0000\u0000\u0000\u0000\u0000\u0000\u0000\u0001\u0000\u0000\u0000\u0000\u0000\u0000\u0000\u0001\u0000\u0000\u0000\u0000\u0000\u0000\u0000\u0000\u0000\u0000\u0000\u0000\u0000\u0000\u0000\u0000\u0000\u0000\u0000ÿÿ\u0000\u0000\u0000\u0000\u0000\u0000", "PMU.109\u0000\u0000\u0000\u0000\u0000\u0000\u0000\u0000\u0000\u0000m\u0000\u000f\u0000\u0006\u0000\u0003\u0000\u0001PZR.AI          PZR.BV          PZR.CI          PZR.AV          PZR.BI          PZR.CV          ANA1            ANA2            ANA3            DIG.stat1_01    DIG.stat1_02    DIG.stat1_03    DIG.stat1_04    DIG.stat1_05    DIG.stat1_06    DIG.stat1_07    DIG.stat1_08    DIG.stat1_09    DIG.stat1_10    DIG.stat1_11    DIG.stat1_12    DIG.stat1_13    DIG.stat1_14    DIG.stat1_15    DIG.stat1_16    \u0001\u0000\u0000\u0000\u0000\u0000\u0000\u0000\u0001\u0000\u0000\u0000\u0000\u0000\u0000\u0000\u0001\u0000\u0000\u0000\u0000\u0000\u0000\u0000\u0000\u0000\u0000\u0000\u0000\u0000\u0000\u0000\u0000\u0000\u0000\u0000ÿÿ\u0000\u0000\u0000\u0000\u0000\u0000", "PMU.110\u0000\u0000\u0000\u0000\u0000\u0000\u0000\u0000\u0000\u0000n\u0000\u000f\u0000\u0006\u0000\u0003\u0000\u0001PZR.AI          PZR.BV          PZR.CI          PZR.AV          PZR.BI          PZR.CV          ANA1            ANA2            ANA3            DIG.stat1_01    DIG.stat1_02    DIG.stat1_03    DIG.stat1_04    DIG.stat1_05    DIG.stat1_06    DIG.stat1_07    DIG.stat1_08    DIG.stat1_09    DIG.stat1_10    DIG.stat1_11    DIG.stat1_12    DIG.stat1_13    DIG.stat1_14    DIG.stat1_15    DIG.stat1_16    \u0001\u0000\u0000\u0000\u0000\u0000\u0000\u0000\u0001\u0000\u0000\u0000\u0000\u0000\u0000\u0000\u0001\u0000\u0000\u0000\u0000\u0000\u0000\u0000\u0000\u0000\u0000\u0000\u0000\u0000\u0000\u0000\u0000\u0000\u0000\u0000ÿÿ\u0000\u0000\u0000\u0000\u0000\u0000", "PMU.111\u0000\u0000\u0000\u0000\u0000\u0000\u0000\u0000\u0000\u0000o\u0000\u000f\u0000\u0006\u0000\u0003\u0000\u0001PZR.AI          PZR.BV          PZR.CI          PZR.AV          PZR.BI          PZR.CV          ANA1            ANA2            ANA3            DIG.stat1_01    DIG.stat1_02    DIG.stat1_03    DIG.stat1_04    DIG.stat1_05    DIG.stat1_06    DIG.stat1_07    DIG.stat1_08    DIG.stat1_09    DIG.stat1_10    DIG.stat1_11    DIG.stat1_12    DIG.stat1_13    DIG.stat1_14    DIG.stat1_15    DIG.stat1_16    \u0001\u0000\u0000\u0000\u0000\u0000\u0000\u0000\u0001\u0000\u0000\u0000\u0000\u0000\u0000\u0000\u0001\u0000\u0000\u0000\u0000\u0000\u0000\u0000\u0000\u0000\u0000\u0000\u0000\u0000\u0000\u0000\u0000\u0000\u0000\u0000ÿÿ\u0000\u0000\u0000\u0000\u0000\u0000", "PMU.112\u0000\u0000\u0000\u0000\u0000\u0000\u0000\u0000\u0000\u0000p\u0000\u000f\u0000\u0006\u0000\u0003\u0000\u0001PZR.AI          PZR.BV          PZR.CI          PZR.AV          PZR.BI          PZR.CV          ANA1            ANA2            ANA3            DIG.stat1_01    DIG.stat1_02    DIG.stat1_03    DIG.stat1_04    DIG.stat1_05    DIG.stat1_06    DIG.stat1_07    DIG.stat1_08    DIG.stat1_09    DIG.stat1_10    DIG.stat1_11    DIG.stat1_12    DIG.stat1_13    DIG.stat1_14    DIG.stat1_15    DIG.stat1_16    \u0001\u0000\u0000\u0000\u0000\u0000\u0000\u0000\u0001\u0000\u0000\u0000\u0000\u0000\u0000\u0000\u0001\u0000\u0000\u0000\u0000\u0000\u0000\u0000\u0000\u0000\u0000\u0000\u0000\u0000\u0000\u0000\u0000\u0000\u0000\u0000ÿÿ\u0000\u0000\u0000\u0000\u0000\u0000", "PMU.113\u0000\u0000\u0000\u0000\u0000\u0000\u0000\u0000\u0000\u0000q\u0000\u000f\u0000\u0006\u0000\u0003\u0000\u0001PZR.AI          PZR.BV          PZR.CI          PZR.AV          PZR.BI          PZR.CV          ANA1            ANA2            ANA3            DIG.stat1_01    DIG.stat1_02    DIG.stat1_03    DIG.stat1_04    DIG.stat1_05    DIG.stat1_06    DIG.stat1_07    DIG.stat1_08    DIG.stat1_09    DIG.stat1_10    DIG.stat1_11    DIG.stat1_12    DIG.stat1_13    DIG.stat1_14    DIG.stat1_15    DIG.stat1_16    \u0001\u0000\u0000\u0000\u0000\u0000\u0000\u0000\u0001\u0000\u0000\u0000\u0000\u0000\u0000\u0000\u0001\u0000\u0000\u0000\u0000\u0000\u0000\u0000\u0000\u0000\u0000\u0000\u0000\u0000\u0000\u0000\u0000\u0000\u0000\u0000ÿÿ\u0000\u0000\u0000\u0000\u0000\u0000", "PMU.114\u0000\u0000\u0000\u0000\u0000\u0000\u0000\u0000\u0000\u0000r\u0000\u000f\u0000\u0006\u0000\u0003\u0000\u0001PZR.AI          PZR.BV          PZR.CI          PZR.AV          PZR.BI          PZR.CV          ANA1            ANA2            ANA3            DIG.stat1_01    DIG.stat1_02    DIG.stat1_03    DIG.stat1_04    DIG.stat1_05    DIG.stat1_06    DIG.stat1_07    DIG.stat1_08    DIG.stat1_09    DIG.stat1_10    DIG.stat1_11    DIG.stat1_12    DIG.stat1_13    DIG.stat1_14    DIG.stat1_15    DIG.stat1_16    \u0001\u0000\u0000\u0000\u0000\u0000\u0000\u0000\u0001\u0000\u0000\u0000\u0000\u0000\u0000\u0000\u0001\u0000\u0000\u0000\u0000\u0000\u0000\u0000\u0000\u0000\u0000\u0000\u0000\u0000\u0000\u0000\u0000\u0000\u0000\u0000ÿÿ\u0000\u0000\u0000\u0000\u0000\u0000", "PMU.115\u0000\u0000\u0000\u0000\u0000\u0000\u0000\u0000\u0000\u0000s\u0000\u000f\u0000\u0006\u0000\u0003\u0000\u0001PZR.AI          PZR.BV          PZR.CI          PZR.AV          PZR.BI          PZR.CV          ANA1            ANA2            ANA3            DIG.stat1_01    DIG.stat1_02    DIG.stat1_03    DIG.stat1_04    DIG.stat1_05    DIG.stat1_06    DIG.stat1_07    DIG.stat1_08    DIG.stat1_09    DIG.stat1_10    DIG.stat1_11    DIG.stat1_12    DIG.stat1_13    DIG.stat1_14    DIG.stat1_15    DIG.stat1_16    \u0001\u0000\u0000\u0000\u0000\u0000\u0000\u0000\u0001\u0000\u0000\u0000\u0000\u0000\u0000\u0000\u0001\u0000\u0000\u0000\u0000\u0000\u0000\u0000\u0000\u0000\u0000\u0000\u0000\u0000\u0000\u0000\u0000\u0000\u0000\u0000ÿÿ\u0000\u0000\u0000\u0000\u0000\u0000", "PMU.116\u0000\u0000\u0000\u0000\u0000\u0000\u0000\u0000\u0000\u0000t\u0000\u000f\u0000\u0006\u0000\u0003\u0000\u0001PZR.AI          PZR.BV          PZR.CI          PZR.AV          PZR.BI          PZR.CV          ANA1            ANA2            ANA3            DIG.stat1_01    DIG.stat1_02    DIG.stat1_03    DIG.stat1_04    DIG.stat1_05    DIG.stat1_06    DIG.stat1_07    DIG.stat1_08    DIG.stat1_09    DIG.stat1_10    DIG.stat1_11    DIG.stat1_12    DIG.stat1_13    DIG.stat1_14    DIG.stat1_15    DIG.stat1_16    \u0001\u0000\u0000\u0000\u0000\u0000\u0000\u0000\u0001\u0000\u0000\u0000\u0000\u0000\u0000\u0000\u0001\u0000\u0000\u0000\u0000\u0000\u0000\u0000\u0000\u0000\u0000\u0000\u0000\u0000\u0000\u0000\u0000\u0000\u0000\u0000ÿÿ\u0000\u0000\u0000\u0000\u0000\u0000", "PMU.117\u0000\u0000\u0000\u0000\u0000\u0000\u0000\u0000\u0000\u0000u\u0000\u000f\u0000\u0006\u0000\u0003\u0000\u0001PZR.AI          PZR.BV          PZR.CI          PZR.AV          PZR.BI          PZR.CV          ANA1            ANA2            ANA3            DIG.stat1_01    DIG.stat1_02    DIG.stat1_03    DIG.stat1_04    DIG.stat1_05    DIG.stat1_06    DIG.stat1_07    DIG.stat1_08    DIG.stat1_09    DIG.stat1_10    DIG.stat1_11    DIG.stat1_12    DIG.stat1_13    DIG.stat1_14    DIG.stat1_15    DIG.stat1_16    \u0001\u0000\u0000\u0000\u0000\u0000\u0000\u0000\u0001\u0000\u0000\u0000\u0000\u0000\u0000\u0000\u0001\u0000\u0000\u0000\u0000\u0000\u0000\u0000\u0000\u0000\u0000\u0000\u0000\u0000\u0000\u0000\u0000\u0000\u0000\u0000ÿÿ\u0000\u0000\u0000\u0000\u0000\u0000", "PMU.118\u0000\u0000\u0000\u0000\u0000\u0000\u0000\u0000\u0000\u0000v\u0000\u000f\u0000\u0006\u0000\u0003\u0000\u0001PZR.AI          PZR.BV          PZR.CI          PZR.AV          PZR.BI          PZR.CV          ANA1            ANA2            ANA3            DIG.stat1_01    DIG.stat1_02    DIG.stat1_03    DIG.stat1_04    DIG.stat1_05    DIG.stat1_06    DIG.stat1_07    DIG.stat1_08    DIG.stat1_09    DIG.stat1_10    DIG.stat1_11    DIG.stat1_12    DIG.stat1_13    DIG.stat1_14    DIG.stat1_15    DIG.stat1_16    \u0001\u0000\u0000\u0000\u0000\u0000\u0000\u0000\u0001\u0000\u0000\u0000\u0000\u0000\u0000\u0000\u0001\u0000\u0000\u0000\u0000\u0000\u0000\u0000\u0000\u0000\u0000\u0000\u0000\u0000\u0000\u0000\u0000\u0000\u0000\u0000ÿÿ\u0000\u0000\u0000\u0000\u0000\u0000", "PMU.119\u0000\u0000\u0000\u0000\u0000\u0000\u0000\u0000\u0000\u0000w\u0000\u000f\u0000\u0006\u0000\u0003\u0000\u0001PZR.AI          PZR.BV          PZR.CI          PZR.AV          PZR.BI          PZR.CV          ANA1            ANA2            ANA3            DIG.stat1_01    DIG.stat1_02    DIG.stat1_03    DIG.stat1_04    DIG.stat1_05    DIG.stat1_06    DIG.stat1_07    DIG.stat1_08    DIG.stat1_09    DIG.stat1_10    DIG.stat1_11    DIG.stat1_12    DIG.stat1_13    DIG.stat1_14    DIG.stat1_15    DIG.stat1_16    \u0001\u0000\u0000\u0000\u0000\u0000\u0000\u0000\u0001\u0000\u0000\u0000\u0000\u0000\u0000\u0000\u0001\u0000\u0000\u0000\u0000\u0000\u0000\u0000\u0000\u0000\u0000\u0000\u0000\u0000\u0000\u0000\u0000\u0000\u0000\u0000ÿÿ\u0000\u0000\u0000\u0000\u0000\u0000", "PMU.120\u0000\u0000\u0000\u0000\u0000\u0000\u0000\u0000\u0000\u0000x\u0000\u000f\u0000\u0006\u0000\u0003\u0000\u0001PZR.AI          PZR.BV          PZR.CI          PZR.AV          PZR.BI          PZR.CV          ANA1            ANA2            ANA3            DIG.stat1_01    DIG.stat1_02    DIG.stat1_03    DIG.stat1_04    DIG.stat1_05    DIG.stat1_06    DIG.stat1_07    DIG.stat1_08    DIG.stat1_09    DIG.stat1_10    DIG.stat1_11    DIG.stat1_12    DIG.stat1_13    DIG.stat1_14    DIG.stat1_15    DIG.stat1_16    \u0001\u0000\u0000\u0000\u0000\u0000\u0000\u0000\u0001\u0000\u0000\u0000\u0000\u0000\u0000\u0000\u0001\u0000\u0000\u0000\u0000\u0000\u0000\u0000\u0000\u0000\u0000\u0000\u0000\u0000\u0000\u0000\u0000\u0000\u0000\u0000ÿÿ\u0000\u0000\u0000\u0000\u0000\u0000", "PMU.121\u0000\u0000\u0000\u0000\u0000\u0000\u0000\u0000\u0000\u0000y\u0000\u000f\u0000\u0006\u0000\u0003\u0000\u0001PZR.AI          PZR.BV          PZR.CI          PZR.AV          PZR.BI          PZR.CV          ANA1            ANA2            ANA3            DIG.stat1_01    DIG.stat1_02    DIG.stat1_03    DIG.stat1_04    DIG.stat1_05    DIG.stat1_06    DIG.stat1_07    DIG.stat1_08    DIG.stat1_09    DIG.stat1_10    DIG.stat1_11    DIG.stat1_12    DIG.stat1_13    DIG.stat1_14    DIG.stat1_15    DIG.stat1_16    \u0001\u0000\u0000\u0000\u0000\u0000\u0000\u0000\u0001\u0000\u0000\u0000\u0000\u0000\u0000\u0000\u0001\u0000\u0000\u0000\u0000\u0000\u0000\u0000\u0000\u0000\u0000\u0000\u0000\u0000\u0000\u0000\u0000\u0000\u0000\u0000ÿÿ\u0000\u0000\u0000\u0000\u0000\u0000", "PMU.122\u0000\u0000\u0000\u0000\u0000\u0000\u0000\u0000\u0000\u0000z\u0000\u000f\u0000\u0006\u0000\u0003\u0000\u0001PZR.AI          PZR.BV          PZR.CI          PZR.AV          PZR.BI          PZR.CV          ANA1            ANA2            ANA3            DIG.stat1_01    DIG.stat1_02    DIG.stat1_03    DIG.stat1_04    DIG.stat1_05    DIG.stat1_06    DIG.stat1_07    DIG.stat1_08    DIG.stat1_09    DIG.stat1_10    DIG.stat1_11    DIG.stat1_12    DIG.stat1_13    DIG.stat1_14    DIG.stat1_15    DIG.stat1_16    \u0001\u0000\u0000\u0000\u0000\u0000\u0000\u0000\u0001\u0000\u0000\u0000\u0000\u0000\u0000\u0000\u0001\u0000\u0000\u0000\u0000\u0000\u0000\u0000\u0000\u0000\u0000\u0000\u0000\u0000\u0000\u0000\u0000\u0000\u0000\u0000ÿÿ\u0000\u0000\u0000\u0000\u0000\u0000", "PMU.123\u0000\u0000\u0000\u0000\u0000\u0000\u0000\u0000\u0000\u0000{\u0000\u000f\u0000\u0006\u0000\u0003\u0000\u0001PZR.AI          PZR.BV          PZR.CI          PZR.AV          PZR.BI          PZR.CV          ANA1            ANA2            ANA3            DIG.stat1_01    DIG.stat1_02    DIG.stat1_03    DIG.stat1_04    DIG.stat1_05    DIG.stat1_06    DIG.stat1_07    DIG.stat1_08    DIG.stat1_09    DIG.stat1_10    DIG.stat1_11    DIG.stat1_12    DIG.stat1_13    DIG.stat1_14    DIG.stat1_15    DIG.stat1_16    \u0001\u0000\u0000\u0000\u0000\u0000\u0000\u0000\u0001\u0000\u0000\u0000\u0000\u0000\u0000\u0000\u0001\u0000\u0000\u0000\u0000\u0000\u0000\u0000\u0000\u0000\u0000\u0000\u0000\u0000\u0000\u0000\u0000\u0000\u0000\u0000ÿÿ\u0000\u0000\u0000\u0000\u0000\u0000", "PMU.124\u0000\u0000\u0000\u0000\u0000\u0000\u0000\u0000\u0000\u0000|\u0000\u000f\u0000\u0006\u0000\u0003\u0000\u0001PZR.AI          PZR.BV          PZR.CI          PZR.AV          PZR.BI          PZR.CV          ANA1            ANA2            ANA3            DIG.stat1_01    DIG.stat1_02    DIG.stat1_03    DIG.stat1_04    DIG.stat1_05    DIG.stat1_06    DIG.stat1_07    DIG.stat1_08    DIG.stat1_09    DIG.stat1_10    DIG.stat1_11    DIG.stat1_12    DIG.stat1_13    DIG.stat1_14    DIG.stat1_15    DIG.stat1_16    \u0001\u0000\u0000\u0000\u0000\u0000\u0000\u0000\u0001\u0000\u0000\u0000\u0000\u0000\u0000\u0000\u0001\u0000\u0000\u0000\u0000\u0000\u0000\u0000\u0000\u0000\u0000\u0000\u0000\u0000\u0000\u0000\u0000\u0000\u0000\u0000ÿÿ\u0000\u0000\u0000\u0000\u0000\u0000", "PMU.125\u0000\u0000\u0000\u0000\u0000\u0000\u0000\u0000\u0000\u0000}\u0000\u000f\u0000\u0006\u0000\u0003\u0000\u0001PZR.AI          PZR.BV          PZR.CI          PZR.AV          PZR.BI          PZR.CV          ANA1            ANA2            ANA3            DIG.stat1_01    DIG.stat1_02    DIG.stat1_03    DIG.stat1_04    DIG.stat1_05    DIG.stat1_06    DIG.stat1_07    DIG.stat1_08    DIG.stat1_09    DIG.stat1_10    DIG.stat1_11    DIG.stat1_12    DIG.stat1_13    DIG.stat1_14    DIG.stat1_15    DIG.stat1_16    \u0001\u0000\u0000\u0000\u0000\u0000\u0000\u0000\u0001\u0000\u0000\u0000\u0000\u0000\u0000\u0000\u0001\u0000\u0000\u0000\u0000\u0000\u0000\u0000\u0000\u0000\u0000\u0000\u0000\u0000\u0000\u0000\u0000\u0000\u0000\u0000ÿÿ\u0000\u0000\u0000\u0000\u0000\u0000", "PMU.126\u0000\u0000\u0000\u0000\u0000\u0000\u0000\u0000\u0000\u0000~\u0000\u000f\u0000\u0006\u0000\u0003\u0000\u0001PZR.AI          PZR.BV          PZR.CI          PZR.AV          PZR.BI          PZR.CV          ANA1            ANA2            ANA3            DIG.stat1_01    DIG.stat1_02    DIG.stat1_03    DIG.stat1_04    DIG.stat1_05    DIG.stat1_06    DIG.stat1_07    DIG.stat1_08    DIG.stat1_09    DIG.stat1_10    DIG.stat1_11    DIG.stat1_12    DIG.stat1_13    DIG.stat1_14    DIG.stat1_15    DIG.stat1_16    \u0001\u0000\u0000\u0000\u0000\u0000\u0000\u0000\u0001\u0000\u0000\u0000\u0000\u0000\u0000\u0000\u0001\u0000\u0000\u0000\u0000\u0000\u0000\u0000\u0000\u0000\u0000\u0000\u0000\u0000\u0000\u0000\u0000\u0000\u0000\u0000ÿÿ\u0000\u0000\u0000\u0000\u0000\u0000", "PMU.127\u0000\u0000\u0000\u0000\u0000\u0000\u0000\u0000\u0000\u0000\u0000\u000f\u0000\u0006\u0000\u0003\u0000\u0001PZR.AI          PZR.BV          PZR.CI          PZR.AV          PZR.BI          PZR.CV          ANA1            ANA2            ANA3            DIG.stat1_01    DIG.stat1_02    DIG.stat1_03    DIG.stat1_04    DIG.stat1_05    DIG.stat1_06    DIG.stat1_07    DIG.stat1_08    DIG.stat1_09    DIG.stat1_10    DIG.stat1_11    DIG.stat1_12    DIG.stat1_13    DIG.stat1_14    DIG.stat1_15    DIG.stat1_16    \u0001\u0000\u0000\u0000\u0000\u0000\u0000\u0000\u0001\u0000\u0000\u0000\u0000\u0000\u0000\u0000\u0001\u0000\u0000\u0000\u0000\u0000\u0000\u0000\u0000\u0000\u0000\u0000\u0000\u0000\u0000\u0000\u0000\u0000\u0000\u0000ÿÿ\u0000\u0000\u0000\u0000\u0000\u0000", "PMU.128\u0000\u0000\u0000\u0000\u0000\u0000\u0000\u0000\u0000\u0000€\u0000\u000f\u0000\u0006\u0000\u0003\u0000\u0001PZR.AI          PZR.BV          PZR.CI          PZR.AV          PZR.BI          PZR.CV          ANA1            ANA2            ANA3            DIG.stat1_01    DIG.stat1_02    DIG.stat1_03    DIG.stat1_04    DIG.stat1_05    DIG.stat1_06    DIG.stat1_07    DIG.stat1_08    DIG.stat1_09    DIG.stat1_10    DIG.stat1_11    DIG.stat1_12    DIG.stat1_13    DIG.stat1_14    DIG.stat1_15    DIG.stat1_16    \u0001\u0000\u0000\u0000\u0000\u0000\u0000\u0000\u0001\u0000\u0000\u0000\u0000\u0000\u0000\u0000\u0001\u0000\u0000\u0000\u0000\u0000\u0000\u0000\u0000\u0000\u0000\u0000\u0000\u0000\u0000\u0000\u0000\u0000\u0000\u0000ÿÿ\u0000\u0000\u0000\u0000\u0000\u0000", "PMU.129\u0000\u0000\u0000\u0000\u0000\u0000\u0000\u0000\u0000\u0000\u0000\u000f\u0000\u0006\u0000\u0003\u0000\u0001PZR.AI          PZR.BV          PZR.CI          PZR.AV          PZR.BI          PZR.CV          ANA1            ANA2            ANA3            DIG.stat1_01    DIG.stat1_02    DIG.stat1_03    DIG.stat1_04    DIG.stat1_05    DIG.stat1_06    DIG.stat1_07    DIG.stat1_08    DIG.stat1_09    DIG.stat1_10    DIG.stat1_11    DIG.stat1_12    DIG.stat1_13    DIG.stat1_14    DIG.stat1_15    DIG.stat1_16    \u0001\u0000\u0000\u0000\u0000\u0000\u0000\u0000\u0001\u0000\u0000\u0000\u0000\u0000\u0000\u0000\u0001\u0000\u0000\u0000\u0000\u0000\u0000\u0000\u0000\u0000\u0000\u0000\u0000\u0000\u0000\u0000\u0000\u0000\u0000\u0000ÿÿ\u0000\u0000\u0000\u0000\u0000\u0000", "PMU.130\u0000\u0000\u0000\u0000\u0000\u0000\u0000\u0000\u0000\u0000‚\u0000\u000f\u0000\u0006\u0000\u0003\u0000\u0001PZR.AI          PZR.BV          PZR.CI          PZR.AV          PZR.BI          PZR.CV          ANA1            ANA2            ANA3            DIG.stat1_01    DIG.stat1_02    DIG.stat1_03    DIG.stat1_04    DIG.stat1_05    DIG.stat1_06    DIG.stat1_07    DIG.stat1_08    DIG.stat1_09    DIG.stat1_10    DIG.stat1_11    DIG.stat1_12    DIG.stat1_13    DIG.stat1_14    DIG.stat1_15    DIG.stat1_16    \u0001\u0000\u0000\u0000\u0000\u0000\u0000\u0000\u0001\u0000\u0000\u0000\u0000\u0000\u0000\u0000\u0001\u0000\u0000\u0000\u0000\u0000\u0000\u0000\u0000\u0000\u0000\u0000\u0000\u0000\u0000\u0000\u0000\u0000\u0000\u0000ÿÿ\u0000\u0000\u0000\u0000\u0000\u0000", "PMU.131\u0000\u0000\u0000\u0000\u0000\u0000\u0000\u0000\u0000\u0000ƒ\u0000\u000f\u0000\u0006\u0000\u0003\u0000\u0001PZR.AI          PZR.BV          PZR.CI          PZR.AV          PZR.BI          PZR.CV          ANA1            ANA2            ANA3            DIG.stat1_01    DIG.stat1_02    DIG.stat1_03    DIG.stat1_04    DIG.stat1_05    DIG.stat1_06    DIG.stat1_07    DIG.stat1_08    DIG.stat1_09    DIG.stat1_10    DIG.stat1_11    DIG.stat1_12    DIG.stat1_13    DIG.stat1_14    DIG.stat1_15    DIG.stat1_16    \u0001\u0000\u0000\u0000\u0000\u0000\u0000\u0000\u0001\u0000\u0000\u0000\u0000\u0000\u0000\u0000\u0001\u0000\u0000\u0000\u0000\u0000\u0000\u0000\u0000\u0000\u0000\u0000\u0000\u0000\u0000\u0000\u0000\u0000\u0000\u0000ÿÿ\u0000\u0000\u0000\u0000\u0000\u0000", "PMU.132\u0000\u0000\u0000\u0000\u0000\u0000\u0000\u0000\u0000\u0000„\u0000\u000f\u0000\u0006\u0000\u0003\u0000\u0001PZR.AI          PZR.BV          PZR.CI          PZR.AV          PZR.BI          PZR.CV          ANA1            ANA2            ANA3            DIG.stat1_01    DIG.stat1_02    DIG.stat1_03    DIG.stat1_04    DIG.stat1_05    DIG.stat1_06    DIG.stat1_07    DIG.stat1_08    DIG.stat1_09    DIG.stat1_10    DIG.stat1_11    DIG.stat1_12    DIG.stat1_13    DIG.stat1_14    DIG.stat1_15    DIG.stat1_16    \u0001\u0000\u0000\u0000\u0000\u0000\u0000\u0000\u0001\u0000\u0000\u0000\u0000\u0000\u0000\u0000\u0001\u0000\u0000\u0000\u0000\u0000\u0000\u0000\u0000\u0000\u0000\u0000\u0000\u0000\u0000\u0000\u0000\u0000\u0000\u0000ÿÿ\u0000\u0000\u0000\u0000\u0000\u0000", "PMU.133\u0000\u0000\u0000\u0000\u0000\u0000\u0000\u0000\u0000\u0000…\u0000\u000f\u0000\u0006\u0000\u0003\u0000\u0001PZR.AI          PZR.BV          PZR.CI          PZR.AV          PZR.BI          PZR.CV          ANA1            ANA2            ANA3            DIG.stat1_01    DIG.stat1_02    DIG.stat1_03    DIG.stat1_04    DIG.stat1_05    DIG.stat1_06    DIG.stat1_07    DIG.stat1_08    DIG.stat1_09    DIG.stat1_10    DIG.stat1_11    DIG.stat1_12    DIG.stat1_13    DIG.stat1_14    DIG.stat1_15    DIG.stat1_16    \u0001\u0000\u0000\u0000\u0000\u0000\u0000\u0000\u0001\u0000\u0000\u0000\u0000\u0000\u0000\u0000\u0001\u0000\u0000\u0000\u0000\u0000\u0000\u0000\u0000\u0000\u0000\u0000\u0000\u0000\u0000\u0000\u0000\u0000\u0000\u0000ÿÿ\u0000\u0000\u0000\u0000\u0000\u0000", "PMU.134\u0000\u0000\u0000\u0000\u0000\u0000\u0000\u0000\u0000\u0000†\u0000\u000f\u0000\u0006\u0000\u0003\u0000\u0001PZR.AI          PZR.BV          PZR.CI          PZR.AV          PZR.BI          PZR.CV          ANA1            ANA2            ANA3            DIG.stat1_01    DIG.stat1_02    DIG.stat1_03    DIG.stat1_04    DIG.stat1_05    DIG.stat1_06    DIG.stat1_07    DIG.stat1_08    DIG.stat1_09    DIG.stat1_10    DIG.stat1_11    DIG.stat1_12    DIG.stat1_13    DIG.stat1_14    DIG.stat1_15    DIG.stat1_16    \u0001\u0000\u0000\u0000\u0000\u0000\u0000\u0000\u0001\u0000\u0000\u0000\u0000\u0000\u0000\u0000\u0001\u0000\u0000\u0000\u0000\u0000\u0000\u0000\u0000\u0000\u0000\u0000\u0000\u0000\u0000\u0000\u0000\u0000\u0000\u0000ÿÿ\u0000\u0000\u0000\u0000\u0000\u0000", "PMU.135\u0000\u0000\u0000\u0000\u0000\u0000\u0000\u0000\u0000\u0000‡\u0000\u000f\u0000\u0006\u0000\u0003\u0000\u0001PZR.AI          PZR.BV          PZR.CI          PZR.AV          PZR.BI          PZR.CV          ANA1            ANA2            ANA3            DIG.stat1_01    DIG.stat1_02    DIG.stat1_03    DIG.stat1_04    DIG.stat1_05    DIG.stat1_06    DIG.stat1_07    DIG.stat1_08    DIG.stat1_09    DIG.stat1_10    DIG.stat1_11    DIG.stat1_12    DIG.stat1_13    DIG.stat1_14    DIG.stat1_15    DIG.stat1_16    \u0001\u0000\u0000\u0000\u0000\u0000\u0000\u0000\u0001\u0000\u0000\u0000\u0000\u0000\u0000\u0000\u0001\u0000\u0000\u0000\u0000\u0000\u0000\u0000\u0000\u0000\u0000\u0000\u0000\u0000\u0000\u0000\u0000\u0000\u0000\u0000ÿÿ\u0000\u0000\u0000\u0000\u0000\u0000", "PMU.136\u0000\u0000\u0000\u0000\u0000\u0000\u0000\u0000\u0000\u0000ˆ\u0000\u000f\u0000\u0006\u0000\u0003\u0000\u0001PZR.AI          PZR.BV          PZR.CI          PZR.AV          PZR.BI          PZR.CV          ANA1            ANA2            ANA3            DIG.stat1_01    DIG.stat1_02    DIG.stat1_03    DIG.stat1_04    DIG.stat1_05    DIG.stat1_06    DIG.stat1_07    DIG.stat1_08    DIG.stat1_09    DIG.stat1_10    DIG.stat1_11    DIG.stat1_12    DIG.stat1_13    DIG.stat1_14    DIG.stat1_15    DIG.stat1_16    \u0001\u0000\u0000\u0000\u0000\u0000\u0000\u0000\u0001\u0000\u0000\u0000\u0000\u0000\u0000\u0000\u0001\u0000\u0000\u0000\u0000\u0000\u0000\u0000\u0000\u0000\u0000\u0000\u0000\u0000\u0000\u0000\u0000\u0000\u0000\u0000ÿÿ\u0000\u0000\u0000\u0000\u0000\u0000", "PMU.137\u0000\u0000\u0000\u0000\u0000\u0000\u0000\u0000\u0000\u0000‰\u0000\u000f\u0000\u0006\u0000\u0003\u0000\u0001PZR.AI          PZR.BV          PZR.CI          PZR.AV          PZR.BI          PZR.CV          ANA1            ANA2            ANA3            DIG.stat1_01    DIG.stat1_02    DIG.stat1_03    DIG.stat1_04    DIG.stat1_05    DIG.stat1_06    DIG.stat1_07    DIG.stat1_08    DIG.stat1_09    DIG.stat1_10    DIG.stat1_11    DIG.stat1_12    DIG.stat1_13    DIG.stat1_14    DIG.stat1_15    DIG.stat1_16    \u0001\u0000\u0000\u0000\u0000\u0000\u0000\u0000\u0001\u0000\u0000\u0000\u0000\u0000\u0000\u0000\u0001\u0000\u0000\u0000\u0000\u0000\u0000\u0000\u0000\u0000\u0000\u0000\u0000\u0000\u0000\u0000\u0000\u0000\u0000\u0000ÿÿ\u0000\u0000\u0000\u0000\u0000\u0000", "PMU.138\u0000\u0000\u0000\u0000\u0000\u0000\u0000\u0000\u0000\u0000Š\u0000\u000f\u0000\u0006\u0000\u0003\u0000\u0001PZR.AI          PZR.BV          PZR.CI          PZR.AV          PZR.BI          PZR.CV          ANA1            ANA2            ANA3            DIG.stat1_01    DIG.stat1_02    DIG.stat1_03    DIG.stat1_04    DIG.stat1_05    DIG.stat1_06    DIG.stat1_07    DIG.stat1_08    DIG.stat1_09    DIG.stat1_10    DIG.stat1_11    DIG.stat1_12    DIG.stat1_13    DIG.stat1_14    DIG.stat1_15    DIG.stat1_16    \u0001\u0000\u0000\u0000\u0000\u0000\u0000\u0000\u0001\u0000\u0000\u0000\u0000\u0000\u0000\u0000\u0001\u0000\u0000\u0000\u0000\u0000\u0000\u0000\u0000\u0000\u0000\u0000\u0000\u0000\u0000\u0000\u0000\u0000\u0000\u0000ÿÿ\u0000\u0000\u0000\u0000\u0000\u0000", "PMU.139\u0000\u0000\u0000\u0000\u0000\u0000\u0000\u0000\u0000\u0000‹\u0000\u000f\u0000\u0006\u0000\u0003\u0000\u0001PZR.AI          PZR.BV          PZR.CI          PZR.AV          PZR.BI          PZR.CV          ANA1            ANA2            ANA3            DIG.stat1_01    DIG.stat1_02    DIG.stat1_03    DIG.stat1_04    DIG.stat1_05    DIG.stat1_06    DIG.stat1_07    DIG.stat1_08    DIG.stat1_09    DIG.stat1_10    DIG.stat1_11    DIG.stat1_12    DIG.stat1_13    DIG.stat1_14    DIG.stat1_15    DIG.stat1_16    \u0001\u0000\u0000\u0000\u0000\u0000\u0000\u0000\u0001\u0000\u0000\u0000\u0000\u0000\u0000\u0000\u0001\u0000\u0000\u0000\u0000\u0000\u0000\u0000\u0000\u0000\u0000\u0000\u0000\u0000\u0000\u0000\u0000\u0000\u0000\u0000ÿÿ\u0000\u0000\u0000\u0000\u0000\u0000"]}) -> (queue out=w19:refnum<queue>, error out=w18:errorcluster)  [unwired: 3 in, 1 out]
  n101 = Obtain Queue(name (unnamed)="UDP Communication", element data type="" ("string")) -> (queue out=w2:refnum<queue>, error out=w1:errorcluster)  [unwired: 3 in, 1 out]
  n102 = while {
    tunnel: [w264] -> w12
    tunnel: [w263] -> w11
    tunnel: w7 -> [w262]
    tunnel: w9 -> [w261]
    tunnel: w10 -> [w259]
    tunnel: w8 -> [w258]
    tunnel: w2 -> [w256]
    tunnel: w1 -> [w255]
    stop <- w266 stop-if-true
    # "UDP Loop"
    n103 = Dequeue Element(queue=w256, error in (no error)=w255) -> (element=w254:string)  [unwired: 1 in, 3 out]
    "UDP STRNG" <- w254
    n104 = case shown="True" "Display Cluster Output" {
      tunnel: [_ w270] -> w253
      tunnel: w254 -> [_ w270]
      tunnel: [_ w269] -> w260
      tunnel: w254 -> [_ w269]
      tunnel: [FALSE TRUE] -> w257
      frame False {
      }
      frame True {
      }
    }
    "DATA ONLINE" <- w257
    "UDP String" <- w253
    n105 = local read "Stop Button"() -> (w266:bool)
    n106 = UDP Write(address=w258, port or service name=w259, connection ID=w262, data in=w260, 8:w261) -> (error out=w263:errorcluster, 3:w264:refnum<k16>)  [unwired: 1 in]
  }
  n107 = UDP Close(connection ID=w12, 8:w11) -> ()  [unwired: 2 out]
  n108 = while {
    tunnel: w19 -> [w305]
    tunnel: w18 -> [w304]
    tunnel: [w303] -> _
    tunnel: [w302] -> _
    tunnel: w4 -> [w280]
    tunnel: w3 -> [w279]
    tunnel: [w278] -> _
    tunnel: [w277] -> _
    stop <- w301 stop-if-true
    w294 = u32 0
    w290 = 4 ("length (rest)")
    # "Data Frame Parsing"
    n109 = Dequeue Element(queue=w305, error in (no error)=w304) -> (queue out=w303:refnum<queue>, element=w300:cluster{"DATA Type":string, "CFG Type":string[]}, error out=w302:errorcluster)  [unwired: 1 in, 1 out]
    n110 = Unbundle By Name(w300) -> ("DATA Type"=w286:string, "CFG Type"=w299:string[])
    "DATA FRAME" <- w286
    n111 = property on="Names of PMUs" class="LstBox (strict)"() -> ("Value"=w272:i32)  [unwired: 2 in, 2 out]
    n112 = String Subset(string=w286, offset (0)=6, length (rest)=w290) -> (substring=w292:string)
    n113 = String Subset(string=w286, offset (0)=10, length (rest)=w290) -> (substring=w288:string)
    n114 = Index Array(array=w299, index=w272) -> (element=w291:string)
    n115 = property on="TIME_BASE" class="DigNum (strict)"() -> ("Value"=w296:u32)  [unwired: 2 in, 2 out]
    n116 = property on="NUM_of_PMUs" class="DigNum (strict)"() -> ("Value"=w298:u32)  [unwired: 2 in, 2 out]
    n117 = Type Cast(type=w294, x=w292) -> (*(type *) &x=w293:u32)
    n118 = Type Cast(type=w294, x=w288) -> (*(type *) &x=w287:u32)
    n119 = call "PMU_INFO.vi"("data in"=w291) -> ("RET_DATA"=w284:T10)
    n120 = call "PMU_DATA_PACK.vi"("DATA FRAME"=w286, "DATA_IN"=w284, "PMUs_NUM"=w298) -> ("PMU DATA Packet"=→"PMU DATA Packet":string[], "DATA_DTLD"=w275:T11, "STAT FIELD"=→"STAT FIELD  WITH RESPEC TO PMU List":string[])  [unwired: 5 in]
    n121 = call "UNIX-DATE_TIME.vi"("TIME_BASE"=w296, "FRACSEC"=w287, "SOC"=w293) -> ("Date/Time"=w282:string)  [unwired: 1 out]
    n122 = Not Equal?(x=w282, y="1-1-1970, 2:0:0 0.000000") -> (x != y?=w285:bool)
    n123 = Unbundle By Name(w284) -> ("UNITs"=→"UNITs":T2)
    n124 = case shown="True" w285 {
      tunnel: [_ w306] -> w274
      tunnel: w282 -> [_ w306]
      frame False {
      }
      frame True {
      }
    }
    "Date/Time 2" <- w274
    n125 = Bundle By Name(cluster=T7 {"Date/Time"="26-12-2013, 0:30:36 0.866666", "DATA_DTLD"={"PZRs Packet"=[], "FREQ Packet"=[], "DFREQ Packet"=[], "ANG Packet"=[], "DGTL Packet"=[]}}, "DATA_DTLD"=w275, "Date/Time"=w274) -> (w273:T7)
    n126 = Enqueue Element(queue=w280, element=w273, error in (no error)=w279) -> (queue out=w278:refnum<queue>, error out=w277:errorcluster)  [unwired: 1 in, 1 out]
    n127 = local read "Stop Button"() -> (w301:bool)
  }
  n128 = while {
    tunnel: w19 -> [w422]
    tunnel: w18 -> [w421]
    tunnel: w4 -> [w420]
    tunnel: w3 -> [w419]
    tunnel: [w418] -> _
    tunnel: [w417] -> _
    tunnel: [w416] -> _
    tunnel: [w415] -> _
    stop <- w443 stop-if-true
    w338 = 50.05
    w339 = 49.95
    w380 = u16 8
    w383 = u16 4
    w388 = u16 1
    w397 = u16 2
    w438 = u32 0
    w434 = 4 ("length (rest)")
    n129 = local read "STAT FIELD  WITH RESPEC TO PMU List"() -> (w325:string[])
    n130 = Dequeue Element(queue=w422, error in (no error)=w421) -> (queue out=w418:refnum<queue>, element=w442:cluster{"DATA Type":string, "CFG Type":string[]}, error out=w417:errorcluster)  [unwired: 1 in, 1 out]
    n131 = Unbundle By Name(w442) -> ("DATA Type"=w430:string, "CFG Type"=w441:string[])
    "DATA FRAME 2" <- w430
    n132 = local read "Angle (Radians)"() -> (w313:sgl[][])
    n133 = property on="Names of PMUs" class="LstBox (strict)"() -> ("Value"=w413:i32)  [unwired: 2 in, 2 out]
    n134 = local read "Magnitude"() -> (w314:sgl[][])
    n135 = for {
      tunnel: w325 -> [w475] mode=indexing
      tunnel: [w476] -> w324 mode=indexing
      tunnel: [w474] -> w323 mode=indexing
      tunnel: [w464] -> w322 mode=indexing
      tunnel: [w458] -> w321 mode=indexing
      tunnel: [w457] -> w320 mode=indexing
      tunnel: [w456] -> w319 mode=indexing
      w477 = u16 0  # type single
      n136 = Type Cast(type=w477, x=w475) -> (*(type *) &x=w473:u16)
      n137 = Number To Boolean Array(number=w473) -> (Boolean array=w450:bool[])
      n138 = Array Subset(array=w450, index=10, length=1) -> (w454:bool[])
      n139 = Array Subset(array=w450, index=4, length=2) -> (w465:bool[])
      n140 = Array Subset(array=w450, index=13, length=1) -> (w470:bool[])
      n141 = Array Subset(array=w450, index=6, length=3) -> (w462:bool[])
      n142 = Index Array(array=w454, index=0) -> (element=w451:bool)
      n143 = Boolean Array To Number(Boolean array=w465) -> (number=w463:u32)
      n144 = Boolean Array To Number(Boolean array=w462) -> (number=w459:u32)
      n145 = case shown="False" w451 {
        tunnel: [FALSE TRUE] -> w457
        tunnel: ["Configuration are up-to-date" "Configuration Change will become effective in 1 min"] -> w456
        frame False {
        }
        frame True {
        }
      }
      n146 = Index Array(array=w470, index=0) -> (element=w468:bool)
      n147 = case shown="1" w463 {
        tunnel: ["Sync Locked (best quality)" "10 s < Unlocked Time > 100 s" "100 s < Unlocked Time > 1000 s" "Unlocked Time > 1000 s"] -> w464
        frame 0, Default {
        }
        frame 1 {
        }
        frame 2 {
        }
        frame 3 {
        }
      }
      n148 = case shown="5" w459 {
        tunnel: ["Not Used" "< 100 ns" "< 1 micro" "< 10 micro" "< 100 micro" "< 1 ms" "< 10 ms" "> 10 ms / unknown"] -> w458
        frame 0 {
        }
        frame 1 {
        }
        frame 2 {
        }
        frame 3 {
        }
        frame 4 {
        }
        frame 5 {
        }
        frame 6 {
        }
        frame 7, Default {
        }
      }
      n149 = case shown="True" w468 {
        tunnel: [FALSE TRUE] -> w476
        tunnel: ["PMU Sync with GPS" "PMU Not Sync with GPS"] -> w474
        frame False {
        }
        frame True {
        }
      }
    }
    "GPS Sync?" <- w324
    "Status - PMU Sync with GPS" <- w323
    "Unlocked Time" <- w322
    "Time Quality" <- w321
    "Change in Configuration" <- w319
    "Config Change?" <- w320
    n150 = for {
      tunnel: w314 -> [w449] mode=indexing
      tunnel: w313 -> [w448] mode=indexing
      tunnel: [w449] -> w312 mode=concatenating
      tunnel: [w448] -> w310 mode=concatenating
    }
    "Phasor Magnitude" <- w312
    n151 = property on="TIME_BASE" class="DigNum (strict)"() -> ("Value"=w412:u32)  [unwired: 2 in, 2 out]
    n152 = String Subset(string=w430, offset (0)=6, length (rest)=w434) -> (substring=w436:string)
    n153 = String Subset(string=w430, offset (0)=10, length (rest)=w434) -> (substring=w432:string)
    n154 = Index Array(array=w441, index=w413) -> (element=w435:string)
    n155 = property on="NUM_of_PMUs" class="DigNum (strict)"() -> ("Value"=w414:u32)  [unwired: 2 in, 2 out]
    n156 = Type Cast(type=w438, x=w436) -> (*(type *) &x=w437:u32)
    n157 = Type Cast(type=w438, x=w432) -> (*(type *) &x=w431:u32)
    n158 = call "PMU_INFO.vi"("data in"=w435) -> ("RET_DATA"=w428:T10)
    n159 = call "PMU_DATA_PACK.vi"("DATA FRAME"=w430, "DATA_IN"=w428, "PMUs_NUM"=w414) -> ("PMU DATA Packet"=→"PMU DATA Packet 2":string[], "DATA_DTLD"=w410:T11)  [unwired: 5 in, 1 out]
    n160 = call "UNIX-DATE_TIME.vi"("TIME_BASE"=w412, "FRACSEC"=w431, "SOC"=w437) -> ("Date/Time"=w426:string, "seconds"=→"seconds":dbl)
    n161 = expression code="x*180/pi"(w310) -> (w309:sgl[])
    "Phasor Angle (Degrees)" <- w309
    n162 = Not Equal?(x=w426, y="1-1-1970, 2:0:0 0.000000") -> (x != y?=w429:bool)
    n163 = local read "Available Phasors in the PMU/PDC Stream"() -> (w315:string[])
    n164 = Unbundle By Name(w428) -> ("UNITs"=→"UNITs 2":T2)
    n165 = case shown="True" w429 {
      tunnel: [_ w639] -> w423
      tunnel: w426 -> [_ w639]
      frame False {
      }
      frame True {
      }
    }
    "Date/Time 3" <- w423
    n166 = for {
      tunnel: w312 -> [w446] mode=indexing
      tunnel: w309 -> [w445] mode=indexing
      tunnel: "data array [mag, phase (deg)]" -> [w447] mode=indexing
      tunnel: [w444] -> w311 mode=indexing
      n167 = Bundle By Name(cluster=w447, "magnitude"=w446, "phase"=w445) -> (w444:cluster{"magnitude":dbl, "phase":dbl})
    }
    n168 = Bundle By Name(cluster=T7 {"Date/Time"="26-12-2013, 0:30:36 0.866666", "DATA_DTLD"={"PZRs Packet"=[], "FREQ Packet"=[], "DFREQ Packet"=[], "ANG Packet"=[], "DGTL Packet"=[]}}, "DATA_DTLD"=w410, "Date/Time"=w423) -> (w411:T7)
    n169 = call "Polar Plot with Point Options.vi"("data array [mag, phase (deg)]"=w311, "Name"=w315, "Size"="Size") -> ("new picture"=→"Phasor Plot":picture)  [unwired: 12 in]
    n170 = Unbundle By Name(w410) -> ("PZRs Packet"=w403:string[], "FREQ Packet"=w409:string[], "DFREQ Packet"=w408:string[], "ANG Packet"=w384:string[], "DGTL Packet"=w373:string[])
    "PZRs Packet" <- w403
    "FREQ Packet" <- w409
    "DFREQ Packet" <- w408
    "ANG Packet" <- w384
    "DGTL Packet" <- w373
    n171 = Enqueue Element(queue=w420, element=w411, error in (no error)=w419) -> (queue out=w416:refnum<queue>, error out=w415:errorcluster)  [unwired: 1 in, 1 out]
    n172 = local read "Stop Button"() -> (w443:bool)
    n173 = local read "Phasors Floatingpoint?"() -> (w395:bool[])
    n174 = local read "Polar?"() -> (w385:bool[])
    n175 = for {
      tunnel: w384 -> [w531] mode=indexing
      tunnel: [w529] -> w376 mode=indexing
      tunnel: [w528] -> w355 mode=indexing
      i -> [w533]
      n176 = local read "Analog"() -> (w532:u16[])
      n177 = Index Array(array=w532, index=w533) -> (element=w527:u16)
      n178 = for {
        N: w527 -> [w537]
        tunnel: w531 -> [w542]
        shift-right: [w538] -> _
        shift-left: 0 ("offset (0)") -> [w540]
        tunnel: [w536] -> w529 mode=indexing
        tunnel: [w534] -> w528 mode=indexing
        n179 = String Length(string=w542) -> (length=w541:i32)
        n180 = Divide(x=w541, y=w537) -> (x/y=w539:dbl)
        n181 = Add(x=w540, y=w539) -> (x+y=w538:dbl)
        n182 = String Subset(string=w542, offset (0)=w540, length (rest)=w539) -> (substring=w536:string)
        n183 = Type Cast(type=sgl 0.0 ("32-bit IEEE 754"), x=w536) -> (*(type *) &x=w534:sgl)
      }
    }
    "Analogs" <- w376
    n184 = for {
      tunnel: w373 -> [w513] mode=indexing
      tunnel: [w509] -> w375 mode=indexing
      tunnel: [w508] -> w374 mode=indexing
      tunnel: w373 -> [w505] mode=indexing
      tunnel: [w504] -> w372 mode=indexing
      i -> [w514]
      n185 = local read "Digitals"() -> (w511:u16[])
      n186 = Index Array(array=w511, index=w514) -> (element=w510:u16)
      n187 = for {
        N: w510 -> [w521]
        tunnel: w513 -> [w526]
        shift-right: [w522] -> _
        shift-left: 0 ("offset (0)") -> [w524]
        tunnel: [w517] -> w509 mode=indexing
        tunnel: [w520] -> w508 mode=indexing
        tunnel: [w515] -> _ mode=indexing
        n188 = String Length(string=w526) -> (length=w525:i32)
        n189 = Divide(x=w525, y=w521) -> (x/y=w523:dbl)
        n190 = Add(x=w524, y=w523) -> (x+y=w522:dbl)
        n191 = String Subset(string=w526, offset (0)=w524, length (rest)=w523) -> (substring=w517:string)
        n192 = Type Cast(type=u16 0 ("offset (0)"), x=w517) -> (*(type *) &x=w516:u16)
        n193 = Type Cast(type=u16 1 ("y"), x=w517) -> (*(type *) &x=w520:u16)
        n194 = Number To Boolean Array(number=w516) -> (Boolean array=w515:bool[])
      }
      n195 = Type Cast(type=u16 0 ("offset (0)"), x=w505) -> (*(type *) &x=w507:u16)
      n196 = Number To Boolean Array(number=w507) -> (Boolean array=w504:bool[])
    }
    "Array" <- w375
    "Array 2" <- w374
    "Boolean array" <- w372
    n197 = for {
      tunnel: w409 -> [w638] mode=indexing
      tunnel: [w637] -> w369 mode=indexing
      n198 = call "HEX_DEC.vi"("HEX IN"=w638) -> ("DEC OUT"=w637:sgl)
    }
    n199 = for {
      tunnel: w408 -> [w636] mode=indexing
      tunnel: [w635] -> w368 mode=indexing
      n200 = call "HEX_DEC.vi"("HEX IN"=w636) -> ("DEC OUT"=w635:sgl)
    }
    n201 = for {
      tunnel: w403 -> [w553] mode=indexing
      tunnel: [w556] -> w402 mode=indexing
      tunnel: [w554] -> w400 mode=indexing
      tunnel: w395 -> [w552] mode=indexing
      tunnel: [w550] -> w393 mode=indexing
      tunnel: [w546] -> w392 mode=indexing
      tunnel: [w545] -> w391 mode=indexing
      tunnel: w385 -> [w547] mode=indexing
      tunnel: [w548] -> w370 mode=indexing
      tunnel: [w544] -> w367 mode=indexing
      tunnel: [w543] -> w371 mode=indexing
      i -> [w558]
      n202 = local read "Phasor"() -> (w559:u16[])
      n203 = Index Array(array=w559, index=w558) -> (element=w549:u16)
      n204 = for {
        N: w549 -> [w604]
        tunnel: w553 -> [w610]
        shift-right: [w606] -> _
        shift-left: 0 ("offset (0)") -> [w608]
        tunnel: [w605] -> w556 mode=indexing
        n205 = String Length(string=w610) -> (length=w609:i32)
        n206 = Divide(x=w609, y=w604) -> (x/y=w607:dbl)
        n207 = Add(x=w608, y=w607) -> (x+y=w606:dbl)
        n208 = String Subset(string=w610, offset (0)=w608, length (rest)=w607) -> (substring=w605:string)
      }
      n209 = for {
        N: w549 -> [w596]
        tunnel: w553 -> [w601]
        shift-right: [w594] -> _
        shift-left: 0 ("offset (0)") -> [w599]
        tunnel: [w591] -> w554 mode=indexing
        tunnel: w552 -> [w593]
        tunnel: [w589] -> w546 mode=indexing
        n210 = String Length(string=w601) -> (length=w600:i32)
        n211 = Multiply(x=w596, y=2) -> (x*y=w597:i32)
        n212 = Divide(x=w600, y=w597) -> (x/y=w598:dbl)
        n213 = String Subset(string=w601, offset (0)=w599, length (rest)=w598) -> (substring=w591:string)
        n214 = case shown="False" w593 {
          tunnel: [4 ("y") 8 ("y")] -> w592
          frame False {
          }
          frame True {
          }
        }
        n215 = Add(x=w599, y=w592) -> (x+y=w594:i32)
        n216 = Type Cast(type=sgl 0.0 ("32-bit IEEE 754"), x=w591) -> (*(type *) &x=w589:sgl)
      }
      n217 = for {
        N: w549 -> [w581]
        tunnel: w553 -> [w586]
        shift-right: [w579] -> _
        shift-left: 4 -> [w584]
        tunnel: [w575] -> w550 mode=indexing
        tunnel: w552 -> [w578]
        tunnel: [w574] -> w545 mode=indexing
        n218 = String Length(string=w586) -> (length=w585:i32)
        n219 = Multiply(x=w581, y=2) -> (x*y=w582:i32)
        n220 = Divide(x=w585, y=w582) -> (x/y=w583:dbl)
        n221 = String Subset(string=w586, offset (0)=w584, length (rest)=w583) -> (substring=w575:string)
        n222 = case shown="False" w578 {
          tunnel: [4 ("y") 8 ("y")] -> w577
          frame False {
          }
          frame True {
          }
        }
        n223 = Add(x=w584, y=w577) -> (x+y=w579:i32)
        n224 = Type Cast(type=sgl 0.0 ("32-bit IEEE 754"), x=w575) -> (*(type *) &x=w574:sgl)
      }
      n225 = case shown="False" w547 {
        tunnel: w546 -> [w568 w573]
        tunnel: w545 -> [w567 w572]
        tunnel: [w566 w571] -> w548
        frame False {
          n226 = Re/Im To Polar(2:w567, 3:w568) -> (0:w569:sgl[], 1:w570:sgl[])
          n227 = Polar To Complex(1:w569, 2:w570) -> (0:w566:csg[])
        }
        frame True {
          n228 = Polar To Complex(1:w572, 2:w573) -> (0:w571:csg[])
        }
      }
      n229 = case shown="True" w547 {
        tunnel: w546 -> [w563 w565]
        tunnel: w545 -> [w562 w564]
        tunnel: [w561 w565] -> w544
        tunnel: [w560 w564] -> w543
        frame False {
          n230 = Re/Im To Polar(2:w562, 3:w563) -> (0:w560:sgl[], 1:w561:sgl[])
        }
        frame True {
        }
      }
    }
    n231 = property on="Frequency" class="Arr (strict)"("Value"=w369) -> ()  [unwired: 2 in, 2 out]
    n232 = local read "PMU1 CFG Packet"() -> (w404:string[])
    n233 = property on="dFreq" class="Arr (strict)"("Value"=w368) -> ()  [unwired: 2 in, 2 out]
    n234 = for {
      tunnel: w404 -> [w616] mode=indexing
      tunnel: [w630] -> w407 mode=indexing
      tunnel: [w622] -> w406 mode=indexing
      tunnel: [w621] -> w405 mode=indexing
      tunnel: [w611] -> w378 mode=indexing
      n235 = String Subset(string=w616, offset (0)=20, length (rest)=2 ("length (rest)")) -> (substring=w632:string)
      n236 = String Subset(string=w616, offset (0)=22, length (rest)=2 ("length (rest)")) -> (substring=w628:string)
      n237 = String Subset(string=w616, offset (0)=18, length (rest)=2 ("length (rest)")) -> (substring=w619:string)
      n238 = String Subset(string=w616, offset (0)=24, length (rest)=2 ("length (rest)")) -> (substring=w623:string)
      n239 = Type Cast(type=u16 0, x=w632) -> (*(type *) &x=w630:u16)
      n240 = Type Cast(type=u16 0, x=w628) -> (*(type *) &x=w622:u16)
      n241 = Type Cast(type=u16 0 ("element"), x=w619) -> (*(type *) &x=w615:u16)
      n242 = Type Cast(type=u16 0, x=w623) -> (*(type *) &x=w621:u16)
      n243 = Split Number(x=w615) -> (lo(x)=w614:u8)  [unwired: 1 out]
      n244 = And(x=w614, y=u16 15 ("element")) -> (x .and. y?=w611:u16)
    }
    "Phasor" <- w407
    "Analog" <- w406
    "Digitals" <- w405
    "Format" <- w378
    n245 = local read "Names of PMUs"() -> (w354:i32)
    n246 = Transpose 2D Array(2D array=w392) -> (transposed array=→"transposed array 4":sgl[][])
    n247 = And(x=w378, y=w397) -> (x .and. y?=w398:u16[])
    n248 = property on="Complex Phasors" class="Arr (strict)"("Value"=w370) -> ()  [unwired: 2 in, 2 out]
    n249 = Transpose 2D Array(2D array=w400) -> (transposed array=→"Real":string[][])
    n250 = Transpose 2D Array(2D array=w393) -> (transposed array=→"Imaginary":string[][])
    n251 = Transpose 2D Array(2D array=w391) -> (transposed array=→"transposed array 5":sgl[][])
    n252 = And(x=w378, y=w380) -> (x .and. y?=w379:u16[])
    n253 = And(x=w378, y=w383) -> (x .and. y?=w382:u16[])
    n254 = And(x=w378, y=w388) -> (x .and. y?=w387:u16[])
    n255 = Transpose 2D Array(2D array=w402) -> (transposed array=→"Transposed":string[][])
    n256 = property on="Magnitude" class="Arr (strict)"("Value"=w367) -> ()  [unwired: 2 in, 2 out]
    n257 = property on="Angle (Radians)" class="Arr (strict)"("Value"=w371) -> ()  [unwired: 2 in, 2 out]
    n258 = property on="Analog Values" class="Arr (strict)"("Value"=w355) -> ()  [unwired: 2 in, 2 out]
    n259 = Index Array(array=w367, index (row)=w354) -> (element=w316:sgl[])  [unwired: 1 in]
    n260 = Equal?(x=w398, y=w397) -> (x = y?=→"Phasors Floatingpoint?":bool[])
    n261 = Equal?(x=w379, y=w380) -> (x = y?=→"Freq Floating?":bool[])
    n262 = Equal?(x=w382, y=w383) -> (x = y?=→"Analog Floating?":bool[])
    n263 = Equal?(x=w387, y=w388) -> (x = y?=→"Polar?":bool[])
    n264 = Index Array(array=w355, index (row)=w354) -> (element=w353:sgl[])  [unwired: 1 in]
    n265 = local read "seconds"() -> (w341:dbl)
    n266 = local read "Freq"() -> (w337:sgl[])
    n267 = Index Array(array=w337, index=0) -> (element=w335:sgl)
    n268 = local read "Frequency"() -> (w350:sgl[])
    n269 = local read "DATA_RATE"() -> (w349:u32)
    n270 = Less?(x=w335, y=w339) -> (x < y?=w332:bool)
    "Freq < Threshold" <- w332
    n271 = Greater?(x=w335, y=w338) -> (0:w333:bool)
    "Freq >Threshold" <- w333
    n272 = Seconds To Date/Time(time stamp (now)=w341) -> (date time rec=w342:T12)  [unwired: 1 in]
    n273 = local read "dFreq"() -> (w357:sgl[])
    n274 = Or(x=w333, y=w332) -> (x .or. y?=w334:bool)
    n275 = Date/Time To Seconds(2:w342) -> (0:w340:timestamp)  [unwired: 1 in]
    n276 = Reciprocal(x=w349) -> (1/x=w348:dbl)
    n277 = case shown="True" w332 {
      tunnel: ["" "Frequency is lesser than threshold. Increase generation"] -> w331
      frame False {
      }
      frame True {
      }
    }
    n278 = case shown="True" w333 {
      tunnel: ["" "Frequency is greater than threshold. Reduce generation"] -> w330
      frame False {
      }
      frame True {
      }
    }
    n279 = case shown="False" w334 {
      tunnel: ["Frequency is normal" ""] -> w329
      frame False {
      }
      frame True {
      }
    }
    n280 = Build Array(w339) -> (w346:dbl[])
    n281 = Build Array(w338) -> (w345:dbl[])
    n282 = Bundle By Name("t0"=w340, "Y"=w337, "dt"=w348) -> (w327:waveform(sgl))  [unwired: 1 in]
    n283 = local read "seconds"() -> (w365:dbl)
    n284 = Index Array(array=w350, index=w354) -> (element=w361:sgl)
    n285 = Index Array(array=w357, index=w354) -> (element=w358:sgl)
    n286 = Bundle By Name(cluster=w327, "Y"=w346) -> (w326:waveform(sgl))
    n287 = Bundle By Name(cluster=w326, "Y"=w345) -> (w344:waveform(sgl))
    n288 = local read "DATA_RATE"() -> (w363:u32)
    n289 = Build Array(w361) -> (w360:sgl[])
    "Freq" <- w360
    n290 = Build Array(w358) -> (w359:sgl[])
    n291 = Build Array(w327, w326, w344) -> (→"Frequency Monitoring":waveform(sgl)[])
    n292 = Seconds To Date/Time(time stamp (now)=w365) -> (date time rec=w364:T12)  [unwired: 1 in]
    n293 = Reciprocal(x=w363) -> (1/x=w352:dbl)
    n294 = Date/Time To Seconds(2:w364) -> (0:w347:timestamp)  [unwired: 1 in]
    n295 = Bundle By Name("t0"=w347, "Y"=w316, "dt"=w352) -> (→"MagnitudePMU":waveform(sgl))  [unwired: 1 in]
    n296 = Bundle By Name("t0"=w347, "Y"=w360, "dt"=w352) -> (→"FrequencyPMU":waveform(sgl))  [unwired: 1 in]
    n297 = Bundle By Name("t0"=w347, "Y"=w359, "dt"=w352) -> (→"PMUROCOF":waveform(sgl))  [unwired: 1 in]
    n298 = Bundle By Name("t0"=w347, "Y"=w353, "dt"=w352) -> (→"PMUAnalogs":waveform(sgl))  [unwired: 1 in]
    n299 = Build Array(w331, w330, w329) -> (→"Warning":string[])
  }
  n300 = while {
    tunnel: w63 -> [w641]
    tunnel: w61 -> [w646]
    tunnel: [w644] -> _
    tunnel: [w645] -> _
    stop <- w642 stop-if-true
    # "Send Commands"
    n301 = event shown="[1] \"Stop Button\": Mouse Down" {
      selector: _ -> [_ _ _ _]
      dyn-events: _ -> [_ _ _ _]
      timeout: _ -> [_ _ _ _]
      tunnel: [PMU_CMDs."Turn off Transmission of Data Frame" ("command 2") w655 PMU_CMDs."Turn off Transmission of Data Frame" ("command 2") PMU_CMDs."Turn on Transmission of Data Frame" ("command 2")] -> w647
      tunnel: [TRUE ("Stop Button") TRUE ("Stop Button") FALSE ("Stop Button") FALSE ("Stop Button")] -> w642
      tunnel: [_ _ _ w660] -> w643
      tunnel: w641 -> [_ w656 _ _]
      event Timeout {
        n302 = event-data() -> ()  [unwired: 1 in, 3 out]
      }
      event "Stop Button": Mouse Down {
        w655 = PMU_CMDs."Turn off Transmission of Data Frame" ("command 2")
        n303 = event-data() -> ()  [unwired: 1 in, 4 out]
        n304 = local read "Device ID"() -> (w652:u16)
        n305 = call "CMD.vi"("PMU ID"=w652, "command"=w655) -> ("error out"=w653:errorcluster, "CMD"=w654:string)  [unwired: 4 in]
        n306 = TCP Write(connection ID=w656, data in=w654, error in (no error)=w653) -> ()  [unwired: 1 in, 3 out]
      }
      event "DATA OFF": Mouse Down {
        n307 = event-data() -> ()  [unwired: 1 in, 3 out]
      }
      event "DATA ON": Mouse Down {
        n308 = event-data() -> ()  [unwired: 1 in, 3 out]
        n309 = local read "Size of DATA Frame"() -> (w660:u32)
      }
    }
    "Data size to read" <- w643
    n310 = local read "Device ID"() -> (w640:u16)
    n311 = Stop(stop? (T)=w642) -> ()
    n312 = call "CMD.vi"("PMU ID"=w640, "command"=w647) -> ("CMD"=w648:string)  [unwired: 4 in, 1 out]
    "COMMAND Frame" <- w648
    n313 = TCP Write(connection ID=w641, data in=w648, error in (no error)=w646) -> (connection ID out=w644:refnum<k5>, bytes written=→"bytes written":i32, error out=w645:errorcluster)  [unwired: 1 in]
  }
  n314 = while {
    tunnel: w63 -> [w679]
    tunnel: w61 -> [w678]
    tunnel: [w677] -> _
    tunnel: [w676] -> _
    tunnel: w19 -> [w670]
    tunnel: [w669] -> w36
    tunnel: [w668] -> w35
    tunnel: w18 -> [w667]
    tunnel: w30 -> [w665]
    stop <- w674 stop-if-true
    # "Receive Loop"
    n315 = local read "Data size to read"() -> (w673:u32)
    n316 = TCP Read(connection ID=w679, bytes to read=w673, error in (no error)=w678) -> (connection ID out=w682:refnum<k5>, data out=w680:string, error out=w681:errorcluster)  [unwired: 2 in]
    n317 = String Length(string=w680) -> (length=w675:i32)
    "length" <- w675
    n318 = control-ref of="Data size to read"() -> (w671:refnum<vi>)
    n319 = TCP Read(connection ID=w682, bytes to read=w675, error in (no error)=w681) -> (connection ID out=w677:refnum<k5>, data out=w672:string, error out=w676:errorcluster)  [unwired: 2 in]
    n320 = call "DATA_RSHP.vi"("Digital in"=w671, "data in"=w672) -> ("DATA FRAME"=w666:string)
    n321 = Bundle By Name(cluster=cluster{"DATA Type":string, "CFG Type":string[]} {"DATA Type"="", "CFG Type"=["PMU.001\u0000\u0000\u0000\u0000\u0000\u0000\u0000\u0000\u0000\u0000\u0001\u0000\u000f\u0000\u0006\u0000\u0003\u0000\u0001PZR.AI          PZR.BV          PZR.CI          PZR.AV          PZR.BI          PZR.CV          ANA1            ANA2            ANA3            DIG.stat1_01    DIG.stat1_02    DIG.stat1_03    DIG.stat1_04    DIG.stat1_05    DIG.stat1_06    DIG.stat1_07    DIG.stat1_08    DIG.stat1_09    DIG.stat1_10    DIG.stat1_11    DIG.stat1_12    DIG.stat1_13    DIG.stat1_14    DIG.stat1_15    DIG.stat1_16    \u0001\u0000\u0000\u0000\u0000\u0000\u0000\u0000\u0001\u0000\u0000\u0000\u0000\u0000\u0000\u0000\u0001\u0000\u0000\u0000\u0000\u0000\u0000\u0000\u0000\u0000\u0000\u0000\u0000\u0000\u0000\u0000\u0000\u0000\u0000\u0000ÿÿ\u0000\u0000\u0000\u0000\u0000\u0000", "PMU.002\u0000\u0000\u0000\u0000\u0000\u0000\u0000\u0000\u0000\u0000\u0002\u0000\u000f\u0000\u0006\u0000\u0003\u0000\u0001PZR.AI          PZR.BV          PZR.CI          PZR.AV          PZR.BI          PZR.CV          ANA1            ANA2            ANA3            DIG.stat1_01    DIG.stat1_02    DIG.stat1_03    DIG.stat1_04    DIG.stat1_05    DIG.stat1_06    DIG.stat1_07    DIG.stat1_08    DIG.stat1_09    DIG.stat1_10    DIG.stat1_11    DIG.stat1_12    DIG.stat1_13    DIG.stat1_14    DIG.stat1_15    DIG.stat1_16    \u0001\u0000\u0000\u0000\u0000\u0000\u0000\u0000\u0001\u0000\u0000\u0000\u0000\u0000\u0000\u0000\u0001\u0000\u0000\u0000\u0000\u0000\u0000\u0000\u0000\u0000\u0000\u0000\u0000\u0000\u0000\u0000\u0000\u0000\u0000\u0000ÿÿ\u0000\u0000\u0000\u0000\u0000\u0000", "PMU.003\u0000\u0000\u0000\u0000\u0000\u0000\u0000\u0000\u0000\u0000\u0003\u0000\u000f\u0000\u0006\u0000\u0003\u0000\u0001PZR.AI          PZR.BV          PZR.CI          PZR.AV          PZR.BI          PZR.CV          ANA1            ANA2            ANA3            DIG.stat1_01    DIG.stat1_02    DIG.stat1_03    DIG.stat1_04    DIG.stat1_05    DIG.stat1_06    DIG.stat1_07    DIG.stat1_08    DIG.stat1_09    DIG.stat1_10    DIG.stat1_11    DIG.stat1_12    DIG.stat1_13    DIG.stat1_14    DIG.stat1_15    DIG.stat1_16    \u0001\u0000\u0000\u0000\u0000\u0000\u0000\u0000\u0001\u0000\u0000\u0000\u0000\u0000\u0000\u0000\u0001\u0000\u0000\u0000\u0000\u0000\u0000\u0000\u0000\u0000\u0000\u0000\u0000\u0000\u0000\u0000\u0000\u0000\u0000\u0000ÿÿ\u0000\u0000\u0000\u0000\u0000\u0000", "PMU.004\u0000\u0000\u0000\u0000\u0000\u0000\u0000\u0000\u0000\u0000\u0004\u0000\u000f\u0000\u0006\u0000\u0003\u0000\u0001PZR.AI          PZR.BV          PZR.CI          PZR.AV          PZR.BI          PZR.CV          ANA1            ANA2            ANA3            DIG.stat1_01    DIG.stat1_02    DIG.stat1_03    DIG.stat1_04    DIG.stat1_05    DIG.stat1_06    DIG.stat1_07    DIG.stat1_08    DIG.stat1_09    DIG.stat1_10    DIG.stat1_11    DIG.stat1_12    DIG.stat1_13    DIG.stat1_14    DIG.stat1_15    DIG.stat1_16    \u0001\u0000\u0000\u0000\u0000\u0000\u0000\u0000\u0001\u0000\u0000\u0000\u0000\u0000\u0000\u0000\u0001\u0000\u0000\u0000\u0000\u0000\u0000\u0000\u0000\u0000\u0000\u0000\u0000\u0000\u0000\u0000\u0000\u0000\u0000\u0000ÿÿ\u0000\u0000\u0000\u0000\u0000\u0000", "PMU.005\u0000\u0000\u0000\u0000\u0000\u0000\u0000\u0000\u0000\u0000\u0005\u0000\u000f\u0000\u0006\u0000\u0003\u0000\u0001PZR.AI          PZR.BV          PZR.CI          PZR.AV          PZR.BI          PZR.CV          ANA1            ANA2            ANA3            DIG.stat1_01    DIG.stat1_02    DIG.stat1_03    DIG.stat1_04    DIG.stat1_05    DIG.stat1_06    DIG.stat1_07    DIG.stat1_08    DIG.stat1_09    DIG.stat1_10    DIG.stat1_11    DIG.stat1_12    DIG.stat1_13    DIG.stat1_14    DIG.stat1_15    DIG.stat1_16    \u0001\u0000\u0000\u0000\u0000\u0000\u0000\u0000\u0001\u0000\u0000\u0000\u0000\u0000\u0000\u0000\u0001\u0000\u0000\u0000\u0000\u0000\u0000\u0000\u0000\u0000\u0000\u0000\u0000\u0000\u0000\u0000\u0000\u0000\u0000\u0000ÿÿ\u0000\u0000\u0000\u0000\u0000\u0000", "PMU.006\u0000\u0000\u0000\u0000\u0000\u0000\u0000\u0000\u0000\u0000\u0006\u0000\u000f\u0000\u0006\u0000\u0003\u0000\u0001PZR.AI          PZR.BV          PZR.CI          PZR.AV          PZR.BI          PZR.CV          ANA1            ANA2            ANA3            DIG.stat1_01    DIG.stat1_02    DIG.stat1_03    DIG.stat1_04    DIG.stat1_05    DIG.stat1_06    DIG.stat1_07    DIG.stat1_08    DIG.stat1_09    DIG.stat1_10    DIG.stat1_11    DIG.stat1_12    DIG.stat1_13    DIG.stat1_14    DIG.stat1_15    DIG.stat1_16    \u0001\u0000\u0000\u0000\u0000\u0000\u0000\u0000\u0001\u0000\u0000\u0000\u0000\u0000\u0000\u0000\u0001\u0000\u0000\u0000\u0000\u0000\u0000\u0000\u0000\u0000\u0000\u0000\u0000\u0000\u0000\u0000\u0000\u0000\u0000\u0000ÿÿ\u0000\u0000\u0000\u0000\u0000\u0000", "PMU.007\u0000\u0000\u0000\u0000\u0000\u0000\u0000\u0000\u0000\u0000\u0007\u0000\u000f\u0000\u0006\u0000\u0003\u0000\u0001PZR.AI          PZR.BV          PZR.CI          PZR.AV          PZR.BI          PZR.CV          ANA1            ANA2            ANA3            DIG.stat1_01    DIG.stat1_02    DIG.stat1_03    DIG.stat1_04    DIG.stat1_05    DIG.stat1_06    DIG.stat1_07    DIG.stat1_08    DIG.stat1_09    DIG.stat1_10    DIG.stat1_11    DIG.stat1_12    DIG.stat1_13    DIG.stat1_14    DIG.stat1_15    DIG.stat1_16    \u0001\u0000\u0000\u0000\u0000\u0000\u0000\u0000\u0001\u0000\u0000\u0000\u0000\u0000\u0000\u0000\u0001\u0000\u0000\u0000\u0000\u0000\u0000\u0000\u0000\u0000\u0000\u0000\u0000\u0000\u0000\u0000\u0000\u0000\u0000\u0000ÿÿ\u0000\u0000\u0000\u0000\u0000\u0000", "PMU.008\u0000\u0000\u0000\u0000\u0000\u0000\u0000\u0000\u0000\u0000\b\u0000\u000f\u0000\u0006\u0000\u0003\u0000\u0001PZR.AI          PZR.BV          PZR.CI          PZR.AV          PZR.BI          PZR.CV          ANA1            ANA2            ANA3            DIG.stat1_01    DIG.stat1_02    DIG.stat1_03    DIG.stat1_04    DIG.stat1_05    DIG.stat1_06    DIG.stat1_07    DIG.stat1_08    DIG.stat1_09    DIG.stat1_10    DIG.stat1_11    DIG.stat1_12    DIG.stat1_13    DIG.stat1_14    DIG.stat1_15    DIG.stat1_16    \u0001\u0000\u0000\u0000\u0000\u0000\u0000\u0000\u0001\u0000\u0000\u0000\u0000\u0000\u0000\u0000\u0001\u0000\u0000\u0000\u0000\u0000\u0000\u0000\u0000\u0000\u0000\u0000\u0000\u0000\u0000\u0000\u0000\u0000\u0000\u0000ÿÿ\u0000\u0000\u0000\u0000\u0000\u0000", "PMU.009\u0000\u0000\u0000\u0000\u0000\u0000\u0000\u0000\u0000\u0000\t\u0000\u000f\u0000\u0006\u0000\u0003\u0000\u0001PZR.AI          PZR.BV          PZR.CI          PZR.AV          PZR.BI          PZR.CV          ANA1            ANA2            ANA3            DIG.stat1_01    DIG.stat1_02    DIG.stat1_03    DIG.stat1_04    DIG.stat1_05    DIG.stat1_06    DIG.stat1_07    DIG.stat1_08    DIG.stat1_09    DIG.stat1_10    DIG.stat1_11    DIG.stat1_12    DIG.stat1_13    DIG.stat1_14    DIG.stat1_15    DIG.stat1_16    \u0001\u0000\u0000\u0000\u0000\u0000\u0000\u0000\u0001\u0000\u0000\u0000\u0000\u0000\u0000\u0000\u0001\u0000\u0000\u0000\u0000\u0000\u0000\u0000\u0000\u0000\u0000\u0000\u0000\u0000\u0000\u0000\u0000\u0000\u0000\u0000ÿÿ\u0000\u0000\u0000\u0000\u0000\u0000", "PMU.010\u0000\u0000\u0000\u0000\u0000\u0000\u0000\u0000\u0000\u0000\n\u0000\u000f\u0000\u0006\u0000\u0003\u0000\u0001PZR.AI          PZR.BV          PZR.CI          PZR.AV          PZR.BI          PZR.CV          ANA1            ANA2            ANA3            DIG.stat1_01    DIG.stat1_02    DIG.stat1_03    DIG.stat1_04    DIG.stat1_05    DIG.stat1_06    DIG.stat1_07    DIG.stat1_08    DIG.stat1_09    DIG.stat1_10    DIG.stat1_11    DIG.stat1_12    DIG.stat1_13    DIG.stat1_14    DIG.stat1_15    DIG.stat1_16    \u0001\u0000\u0000\u0000\u0000\u0000\u0000\u0000\u0001\u0000\u0000\u0000\u0000\u0000\u0000\u0000\u0001\u0000\u0000\u0000\u0000\u0000\u0000\u0000\u0000\u0000\u0000\u0000\u0000\u0000\u0000\u0000\u0000\u0000\u0000\u0000ÿÿ\u0000\u0000\u0000\u0000\u0000\u0000", "PMU.011\u0000\u0000\u0000\u0000\u0000\u0000\u0000\u0000\u0000\u0000\u000b\u0000\u000f\u0000\u0006\u0000\u0003\u0000\u0001PZR.AI          PZR.BV          PZR.CI          PZR.AV          PZR.BI          PZR.CV          ANA1            ANA2            ANA3            DIG.stat1_01    DIG.stat1_02    DIG.stat1_03    DIG.stat1_04    DIG.stat1_05    DIG.stat1_06    DIG.stat1_07    DIG.stat1_08    DIG.stat1_09    DIG.stat1_10    DIG.stat1_11    DIG.stat1_12    DIG.stat1_13    DIG.stat1_14    DIG.stat1_15    DIG.stat1_16    \u0001\u0000\u0000\u0000\u0000\u0000\u0000\u0000\u0001\u0000\u0000\u0000\u0000\u0000\u0000\u0000\u0001\u0000\u0000\u0000\u0000\u0000\u0000\u0000\u0000\u0000\u0000\u0000\u0000\u0000\u0000\u0000\u0000\u0000\u0000\u0000ÿÿ\u0000\u0000\u0000\u0000\u0000\u0000", "PMU.012\u0000\u0000\u0000\u0000\u0000\u0000\u0000\u0000\u0000\u0000\f\u0000\u000f\u0000\u0006\u0000\u0003\u0000\u0001PZR.AI          PZR.BV          PZR.CI          PZR.AV          PZR.BI          PZR.CV          ANA1            ANA2            ANA3            DIG.stat1_01    DIG.stat1_02    DIG.stat1_03    DIG.stat1_04    DIG.stat1_05    DIG.stat1_06    DIG.stat1_07    DIG.stat1_08    DIG.stat1_09    DIG.stat1_10    DIG.stat1_11    DIG.stat1_12    DIG.stat1_13    DIG.stat1_14    DIG.stat1_15    DIG.stat1_16    \u0001\u0000\u0000\u0000\u0000\u0000\u0000\u0000\u0001\u0000\u0000\u0000\u0000\u0000\u0000\u0000\u0001\u0000\u0000\u0000\u0000\u0000\u0000\u0000\u0000\u0000\u0000\u0000\u0000\u0000\u0000\u0000\u0000\u0000\u0000\u0000ÿÿ\u0000\u0000\u0000\u0000\u0000\u0000", "PMU.013\u0000\u0000\u0000\u0000\u0000\u0000\u0000\u0000\u0000\u0000\r\u0000\u000f\u0000\u0006\u0000\u0003\u0000\u0001PZR.AI          PZR.BV          PZR.CI          PZR.AV          PZR.BI          PZR.CV          ANA1            ANA2            ANA3            DIG.stat1_01    DIG.stat1_02    DIG.stat1_03    DIG.stat1_04    DIG.stat1_05    DIG.stat1_06    DIG.stat1_07    DIG.stat1_08    DIG.stat1_09    DIG.stat1_10    DIG.stat1_11    DIG.stat1_12    DIG.stat1_13    DIG.stat1_14    DIG.stat1_15    DIG.stat1_16    \u0001\u0000\u0000\u0000\u0000\u0000\u0000\u0000\u0001\u0000\u0000\u0000\u0000\u0000\u0000\u0000\u0001\u0000\u0000\u0000\u0000\u0000\u0000\u0000\u0000\u0000\u0000\u0000\u0000\u0000\u0000\u0000\u0000\u0000\u0000\u0000ÿÿ\u0000\u0000\u0000\u0000\u0000\u0000", "PMU.014\u0000\u0000\u0000\u0000\u0000\u0000\u0000\u0000\u0000\u0000\u000e\u0000\u000f\u0000\u0006\u0000\u0003\u0000\u0001PZR.AI          PZR.BV          PZR.CI          PZR.AV          PZR.BI          PZR.CV          ANA1            ANA2            ANA3            DIG.stat1_01    DIG.stat1_02    DIG.stat1_03    DIG.stat1_04    DIG.stat1_05    DIG.stat1_06    DIG.stat1_07    DIG.stat1_08    DIG.stat1_09    DIG.stat1_10    DIG.stat1_11    DIG.stat1_12    DIG.stat1_13    DIG.stat1_14    DIG.stat1_15    DIG.stat1_16    \u0001\u0000\u0000\u0000\u0000\u0000\u0000\u0000\u0001\u0000\u0000\u0000\u0000\u0000\u0000\u0000\u0001\u0000\u0000\u0000\u0000\u0000\u0000\u0000\u0000\u0000\u0000\u0000\u0000\u0000\u0000\u0000\u0000\u0000\u0000\u0000ÿÿ\u0000\u0000\u0000\u0000\u0000\u0000", "PMU.015\u0000\u0000\u0000\u0000\u0000\u0000\u0000\u0000\u0000\u0000\u000f\u0000\u000f\u0000\u0006\u0000\u0003\u0000\u0001PZR.AI          PZR.BV          PZR.CI          PZR.AV          PZR.BI          PZR.CV          ANA1            ANA2            ANA3            DIG.stat1_01    DIG.stat1_02    DIG.stat1_03    DIG.stat1_04    DIG.stat1_05    DIG.stat1_06    DIG.stat1_07    DIG.stat1_08    DIG.stat1_09    DIG.stat1_10    DIG.stat1_11    DIG.stat1_12    DIG.stat1_13    DIG.stat1_14    DIG.stat1_15    DIG.stat1_16    \u0001\u0000\u0000\u0000\u0000\u0000\u0000\u0000\u0001\u0000\u0000\u0000\u0000\u0000\u0000\u0000\u0001\u0000\u0000\u0000\u0000\u0000\u0000\u0000\u0000\u0000\u0000\u0000\u0000\u0000\u0000\u0000\u0000\u0000\u0000\u0000ÿÿ\u0000\u0000\u0000\u0000\u0000\u0000", "PMU.016\u0000\u0000\u0000\u0000\u0000\u0000\u0000\u0000\u0000\u0000\u0010\u0000\u000f\u0000\u0006\u0000\u0003\u0000\u0001PZR.AI          PZR.BV          PZR.CI          PZR.AV          PZR.BI          PZR.CV          ANA1            ANA2            ANA3            DIG.stat1_01    DIG.stat1_02    DIG.stat1_03    DIG.stat1_04    DIG.stat1_05    DIG.stat1_06    DIG.stat1_07    DIG.stat1_08    DIG.stat1_09    DIG.stat1_10    DIG.stat1_11    DIG.stat1_12    DIG.stat1_13    DIG.stat1_14    DIG.stat1_15    DIG.stat1_16    \u0001\u0000\u0000\u0000\u0000\u0000\u0000\u0000\u0001\u0000\u0000\u0000\u0000\u0000\u0000\u0000\u0001\u0000\u0000\u0000\u0000\u0000\u0000\u0000\u0000\u0000\u0000\u0000\u0000\u0000\u0000\u0000\u0000\u0000\u0000\u0000ÿÿ\u0000\u0000\u0000\u0000\u0000\u0000", "PMU.017\u0000\u0000\u0000\u0000\u0000\u0000\u0000\u0000\u0000\u0000\u0011\u0000\u000f\u0000\u0006\u0000\u0003\u0000\u0001PZR.AI          PZR.BV          PZR.CI          PZR.AV          PZR.BI          PZR.CV          ANA1            ANA2            ANA3            DIG.stat1_01    DIG.stat1_02    DIG.stat1_03    DIG.stat1_04    DIG.stat1_05    DIG.stat1_06    DIG.stat1_07    DIG.stat1_08    DIG.stat1_09    DIG.stat1_10    DIG.stat1_11    DIG.stat1_12    DIG.stat1_13    DIG.stat1_14    DIG.stat1_15    DIG.stat1_16    \u0001\u0000\u0000\u0000\u0000\u0000\u0000\u0000\u0001\u0000\u0000\u0000\u0000\u0000\u0000\u0000\u0001\u0000\u0000\u0000\u0000\u0000\u0000\u0000\u0000\u0000\u0000\u0000\u0000\u0000\u0000\u0000\u0000\u0000\u0000\u0000ÿÿ\u0000\u0000\u0000\u0000\u0000\u0000", "PMU.018\u0000\u0000\u0000\u0000\u0000\u0000\u0000\u0000\u0000\u0000\u0012\u0000\u000f\u0000\u0006\u0000\u0003\u0000\u0001PZR.AI          PZR.BV          PZR.CI          PZR.AV          PZR.BI          PZR.CV          ANA1            ANA2            ANA3            DIG.stat1_01    DIG.stat1_02    DIG.stat1_03    DIG.stat1_04    DIG.stat1_05    DIG.stat1_06    DIG.stat1_07    DIG.stat1_08    DIG.stat1_09    DIG.stat1_10    DIG.stat1_11    DIG.stat1_12    DIG.stat1_13    DIG.stat1_14    DIG.stat1_15    DIG.stat1_16    \u0001\u0000\u0000\u0000\u0000\u0000\u0000\u0000\u0001\u0000\u0000\u0000\u0000\u0000\u0000\u0000\u0001\u0000\u0000\u0000\u0000\u0000\u0000\u0000\u0000\u0000\u0000\u0000\u0000\u0000\u0000\u0000\u0000\u0000\u0000\u0000ÿÿ\u0000\u0000\u0000\u0000\u0000\u0000", "PMU.019\u0000\u0000\u0000\u0000\u0000\u0000\u0000\u0000\u0000\u0000\u0013\u0000\u000f\u0000\u0006\u0000\u0003\u0000\u0001PZR.AI          PZR.BV          PZR.CI          PZR.AV          PZR.BI          PZR.CV          ANA1            ANA2            ANA3            DIG.stat1_01    DIG.stat1_02    DIG.stat1_03    DIG.stat1_04    DIG.stat1_05    DIG.stat1_06    DIG.stat1_07    DIG.stat1_08    DIG.stat1_09    DIG.stat1_10    DIG.stat1_11    DIG.stat1_12    DIG.stat1_13    DIG.stat1_14    DIG.stat1_15    DIG.stat1_16    \u0001\u0000\u0000\u0000\u0000\u0000\u0000\u0000\u0001\u0000\u0000\u0000\u0000\u0000\u0000\u0000\u0001\u0000\u0000\u0000\u0000\u0000\u0000\u0000\u0000\u0000\u0000\u0000\u0000\u0000\u0000\u0000\u0000\u0000\u0000\u0000ÿÿ\u0000\u0000\u0000\u0000\u0000\u0000", "PMU.020\u0000\u0000\u0000\u0000\u0000\u0000\u0000\u0000\u0000\u0000\u0014\u0000\u000f\u0000\u0006\u0000\u0003\u0000\u0001PZR.AI          PZR.BV          PZR.CI          PZR.AV          PZR.BI          PZR.CV          ANA1            ANA2            ANA3            DIG.stat1_01    DIG.stat1_02    DIG.stat1_03    DIG.stat1_04    DIG.stat1_05    DIG.stat1_06    DIG.stat1_07    DIG.stat1_08    DIG.stat1_09    DIG.stat1_10    DIG.stat1_11    DIG.stat1_12    DIG.stat1_13    DIG.stat1_14    DIG.stat1_15    DIG.stat1_16    \u0001\u0000\u0000\u0000\u0000\u0000\u0000\u0000\u0001\u0000\u0000\u0000\u0000\u0000\u0000\u0000\u0001\u0000\u0000\u0000\u0000\u0000\u0000\u0000\u0000\u0000\u0000\u0000\u0000\u0000\u0000\u0000\u0000\u0000\u0000\u0000ÿÿ\u0000\u0000\u0000\u0000\u0000\u0000", "PMU.021\u0000\u0000\u0000\u0000\u0000\u0000\u0000\u0000\u0000\u0000\u0015\u0000\u000f\u0000\u0006\u0000\u0003\u0000\u0001PZR.AI          PZR.BV          PZR.CI          PZR.AV          PZR.BI          PZR.CV          ANA1            ANA2            ANA3            DIG.stat1_01    DIG.stat1_02    DIG.stat1_03    DIG.stat1_04    DIG.stat1_05    DIG.stat1_06    DIG.stat1_07    DIG.stat1_08    DIG.stat1_09    DIG.stat1_10    DIG.stat1_11    DIG.stat1_12    DIG.stat1_13    DIG.stat1_14    DIG.stat1_15    DIG.stat1_16    \u0001\u0000\u0000\u0000\u0000\u0000\u0000\u0000\u0001\u0000\u0000\u0000\u0000\u0000\u0000\u0000\u0001\u0000\u0000\u0000\u0000\u0000\u0000\u0000\u0000\u0000\u0000\u0000\u0000\u0000\u0000\u0000\u0000\u0000\u0000\u0000ÿÿ\u0000\u0000\u0000\u0000\u0000\u0000", "PMU.022\u0000\u0000\u0000\u0000\u0000\u0000\u0000\u0000\u0000\u0000\u0016\u0000\u000f\u0000\u0006\u0000\u0003\u0000\u0001PZR.AI          PZR.BV          PZR.CI          PZR.AV          PZR.BI          PZR.CV          ANA1            ANA2            ANA3            DIG.stat1_01    DIG.stat1_02    DIG.stat1_03    DIG.stat1_04    DIG.stat1_05    DIG.stat1_06    DIG.stat1_07    DIG.stat1_08    DIG.stat1_09    DIG.stat1_10    DIG.stat1_11    DIG.stat1_12    DIG.stat1_13    DIG.stat1_14    DIG.stat1_15    DIG.stat1_16    \u0001\u0000\u0000\u0000\u0000\u0000\u0000\u0000\u0001\u0000\u0000\u0000\u0000\u0000\u0000\u0000\u0001\u0000\u0000\u0000\u0000\u0000\u0000\u0000\u0000\u0000\u0000\u0000\u0000\u0000\u0000\u0000\u0000\u0000\u0000\u0000ÿÿ\u0000\u0000\u0000\u0000\u0000\u0000", "PMU.023\u0000\u0000\u0000\u0000\u0000\u0000\u0000\u0000\u0000\u0000\u0017\u0000\u000f\u0000\u0006\u0000\u0003\u0000\u0001PZR.AI          PZR.BV          PZR.CI          PZR.AV          PZR.BI          PZR.CV          ANA1            ANA2            ANA3            DIG.stat1_01    DIG.stat1_02    DIG.stat1_03    DIG.stat1_04    DIG.stat1_05    DIG.stat1_06    DIG.stat1_07    DIG.stat1_08    DIG.stat1_09    DIG.stat1_10    DIG.stat1_11    DIG.stat1_12    DIG.stat1_13    DIG.stat1_14    DIG.stat1_15    DIG.stat1_16    \u0001\u0000\u0000\u0000\u0000\u0000\u0000\u0000\u0001\u0000\u0000\u0000\u0000\u0000\u0000\u0000\u0001\u0000\u0000\u0000\u0000\u0000\u0000\u0000\u0000\u0000\u0000\u0000\u0000\u0000\u0000\u0000\u0000\u0000\u0000\u0000ÿÿ\u0000\u0000\u0000\u0000\u0000\u0000", "PMU.024\u0000\u0000\u0000\u0000\u0000\u0000\u0000\u0000\u0000\u0000\u0018\u0000\u000f\u0000\u0006\u0000\u0003\u0000\u0001PZR.AI          PZR.BV          PZR.CI          PZR.AV          PZR.BI          PZR.CV          ANA1            ANA2            ANA3            DIG.stat1_01    DIG.stat1_02    DIG.stat1_03    DIG.stat1_04    DIG.stat1_05    DIG.stat1_06    DIG.stat1_07    DIG.stat1_08    DIG.stat1_09    DIG.stat1_10    DIG.stat1_11    DIG.stat1_12    DIG.stat1_13    DIG.stat1_14    DIG.stat1_15    DIG.stat1_16    \u0001\u0000\u0000\u0000\u0000\u0000\u0000\u0000\u0001\u0000\u0000\u0000\u0000\u0000\u0000\u0000\u0001\u0000\u0000\u0000\u0000\u0000\u0000\u0000\u0000\u0000\u0000\u0000\u0000\u0000\u0000\u0000\u0000\u0000\u0000\u0000ÿÿ\u0000\u0000\u0000\u0000\u0000\u0000", "PMU.025\u0000\u0000\u0000\u0000\u0000\u0000\u0000\u0000\u0000\u0000\u0019\u0000\u000f\u0000\u0006\u0000\u0003\u0000\u0001PZR.AI          PZR.BV          PZR.CI          PZR.AV          PZR.BI          PZR.CV          ANA1            ANA2            ANA3            DIG.stat1_01    DIG.stat1_02    DIG.stat1_03    DIG.stat1_04    DIG.stat1_05    DIG.stat1_06    DIG.stat1_07    DIG.stat1_08    DIG.stat1_09    DIG.stat1_10    DIG.stat1_11    DIG.stat1_12    DIG.stat1_13    DIG.stat1_14    DIG.stat1_15    DIG.stat1_16    \u0001\u0000\u0000\u0000\u0000\u0000\u0000\u0000\u0001\u0000\u0000\u0000\u0000\u0000\u0000\u0000\u0001\u0000\u0000\u0000\u0000\u0000\u0000\u0000\u0000\u0000\u0000\u0000\u0000\u0000\u0000\u0000\u0000\u0000\u0000\u0000ÿÿ\u0000\u0000\u0000\u0000\u0000\u0000", "PMU.026\u0000\u0000\u0000\u0000\u0000\u0000\u0000\u0000\u0000\u0000\u001a\u0000\u000f\u0000\u0006\u0000\u0003\u0000\u0001PZR.AI          PZR.BV          PZR.CI          PZR.AV          PZR.BI          PZR.CV          ANA1            ANA2            ANA3            DIG.stat1_01    DIG.stat1_02    DIG.stat1_03    DIG.stat1_04    DIG.stat1_05    DIG.stat1_06    DIG.stat1_07    DIG.stat1_08    DIG.stat1_09    DIG.stat1_10    DIG.stat1_11    DIG.stat1_12    DIG.stat1_13    DIG.stat1_14    DIG.stat1_15    DIG.stat1_16    \u0001\u0000\u0000\u0000\u0000\u0000\u0000\u0000\u0001\u0000\u0000\u0000\u0000\u0000\u0000\u0000\u0001\u0000\u0000\u0000\u0000\u0000\u0000\u0000\u0000\u0000\u0000\u0000\u0000\u0000\u0000\u0000\u0000\u0000\u0000\u0000ÿÿ\u0000\u0000\u0000\u0000\u0000\u0000", "PMU.027\u0000\u0000\u0000\u0000\u0000\u0000\u0000\u0000\u0000\u0000\u001b\u0000\u000f\u0000\u0006\u0000\u0003\u0000\u0001PZR.AI          PZR.BV          PZR.CI          PZR.AV          PZR.BI          PZR.CV          ANA1            ANA2            ANA3            DIG.stat1_01    DIG.stat1_02    DIG.stat1_03    DIG.stat1_04    DIG.stat1_05    DIG.stat1_06    DIG.stat1_07    DIG.stat1_08    DIG.stat1_09    DIG.stat1_10    DIG.stat1_11    DIG.stat1_12    DIG.stat1_13    DIG.stat1_14    DIG.stat1_15    DIG.stat1_16    \u0001\u0000\u0000\u0000\u0000\u0000\u0000\u0000\u0001\u0000\u0000\u0000\u0000\u0000\u0000\u0000\u0001\u0000\u0000\u0000\u0000\u0000\u0000\u0000\u0000\u0000\u0000\u0000\u0000\u0000\u0000\u0000\u0000\u0000\u0000\u0000ÿÿ\u0000\u0000\u0000\u0000\u0000\u0000", "PMU.028\u0000\u0000\u0000\u0000\u0000\u0000\u0000\u0000\u0000\u0000\u001c\u0000\u000f\u0000\u0006\u0000\u0003\u0000\u0001PZR.AI          PZR.BV          PZR.CI          PZR.AV          PZR.BI          PZR.CV          ANA1            ANA2            ANA3            DIG.stat1_01    DIG.stat1_02    DIG.stat1_03    DIG.stat1_04    DIG.stat1_05    DIG.stat1_06    DIG.stat1_07    DIG.stat1_08    DIG.stat1_09    DIG.stat1_10    DIG.stat1_11    DIG.stat1_12    DIG.stat1_13    DIG.stat1_14    DIG.stat1_15    DIG.stat1_16    \u0001\u0000\u0000\u0000\u0000\u0000\u0000\u0000\u0001\u0000\u0000\u0000\u0000\u0000\u0000\u0000\u0001\u0000\u0000\u0000\u0000\u0000\u0000\u0000\u0000\u0000\u0000\u0000\u0000\u0000\u0000\u0000\u0000\u0000\u0000\u0000ÿÿ\u0000\u0000\u0000\u0000\u0000\u0000", "PMU.029\u0000\u0000\u0000\u0000\u0000\u0000\u0000\u0000\u0000\u0000\u001d\u0000\u000f\u0000\u0006\u0000\u0003\u0000\u0001PZR.AI          PZR.BV          PZR.CI          PZR.AV          PZR.BI          PZR.CV          ANA1            ANA2            ANA3            DIG.stat1_01    DIG.stat1_02    DIG.stat1_03    DIG.stat1_04    DIG.stat1_05    DIG.stat1_06    DIG.stat1_07    DIG.stat1_08    DIG.stat1_09    DIG.stat1_10    DIG.stat1_11    DIG.stat1_12    DIG.stat1_13    DIG.stat1_14    DIG.stat1_15    DIG.stat1_16    \u0001\u0000\u0000\u0000\u0000\u0000\u0000\u0000\u0001\u0000\u0000\u0000\u0000\u0000\u0000\u0000\u0001\u0000\u0000\u0000\u0000\u0000\u0000\u0000\u0000\u0000\u0000\u0000\u0000\u0000\u0000\u0000\u0000\u0000\u0000\u0000ÿÿ\u0000\u0000\u0000\u0000\u0000\u0000", "PMU.030\u0000\u0000\u0000\u0000\u0000\u0000\u0000\u0000\u0000\u0000\u001e\u0000\u000f\u0000\u0006\u0000\u0003\u0000\u0001PZR.AI          PZR.BV          PZR.CI          PZR.AV          PZR.BI          PZR.CV          ANA1            ANA2            ANA3            DIG.stat1_01    DIG.stat1_02    DIG.stat1_03    DIG.stat1_04    DIG.stat1_05    DIG.stat1_06    DIG.stat1_07    DIG.stat1_08    DIG.stat1_09    DIG.stat1_10    DIG.stat1_11    DIG.stat1_12    DIG.stat1_13    DIG.stat1_14    DIG.stat1_15    DIG.stat1_16    \u0001\u0000\u0000\u0000\u0000\u0000\u0000\u0000\u0001\u0000\u0000\u0000\u0000\u0000\u0000\u0000\u0001\u0000\u0000\u0000\u0000\u0000\u0000\u0000\u0000\u0000\u0000\u0000\u0000\u0000\u0000\u0000\u0000\u0000\u0000\u0000ÿÿ\u0000\u0000\u0000\u0000\u0000\u0000", "PMU.031\u0000\u0000\u0000\u0000\u0000\u0000\u0000\u0000\u0000\u0000\u001f\u0000\u000f\u0000\u0006\u0000\u0003\u0000\u0001PZR.AI          PZR.BV          PZR.CI          PZR.AV          PZR.BI          PZR.CV          ANA1            ANA2            ANA3            DIG.stat1_01    DIG.stat1_02    DIG.stat1_03    DIG.stat1_04    DIG.stat1_05    DIG.stat1_06    DIG.stat1_07    DIG.stat1_08    DIG.stat1_09    DIG.stat1_10    DIG.stat1_11    DIG.stat1_12    DIG.stat1_13    DIG.stat1_14    DIG.stat1_15    DIG.stat1_16    \u0001\u0000\u0000\u0000\u0000\u0000\u0000\u0000\u0001\u0000\u0000\u0000\u0000\u0000\u0000\u0000\u0001\u0000\u0000\u0000\u0000\u0000\u0000\u0000\u0000\u0000\u0000\u0000\u0000\u0000\u0000\u0000\u0000\u0000\u0000\u0000ÿÿ\u0000\u0000\u0000\u0000\u0000\u0000", "PMU.032\u0000\u0000\u0000\u0000\u0000\u0000\u0000\u0000\u0000\u0000 \u0000\u000f\u0000\u0006\u0000\u0003\u0000\u0001PZR.AI          PZR.BV          PZR.CI          PZR.AV          PZR.BI          PZR.CV          ANA1            ANA2            ANA3            DIG.stat1_01    DIG.stat1_02    DIG.stat1_03    DIG.stat1_04    DIG.stat1_05    DIG.stat1_06    DIG.stat1_07    DIG.stat1_08    DIG.stat1_09    DIG.stat1_10    DIG.stat1_11    DIG.stat1_12    DIG.stat1_13    DIG.stat1_14    DIG.stat1_15    DIG.stat1_16    \u0001\u0000\u0000\u0000\u0000\u0000\u0000\u0000\u0001\u0000\u0000\u0000\u0000\u0000\u0000\u0000\u0001\u0000\u0000\u0000\u0000\u0000\u0000\u0000\u0000\u0000\u0000\u0000\u0000\u0000\u0000\u0000\u0000\u0000\u0000\u0000ÿÿ\u0000\u0000\u0000\u0000\u0000\u0000", "PMU.033\u0000\u0000\u0000\u0000\u0000\u0000\u0000\u0000\u0000\u0000!\u0000\u000f\u0000\u0006\u0000\u0003\u0000\u0001PZR.AI          PZR.BV          PZR.CI          PZR.AV          PZR.BI          PZR.CV          ANA1            ANA2            ANA3            DIG.stat1_01    DIG.stat1_02    DIG.stat1_03    DIG.stat1_04    DIG.stat1_05    DIG.stat1_06    DIG.stat1_07    DIG.stat1_08    DIG.stat1_09    DIG.stat1_10    DIG.stat1_11    DIG.stat1_12    DIG.stat1_13    DIG.stat1_14    DIG.stat1_15    DIG.stat1_16    \u0001\u0000\u0000\u0000\u0000\u0000\u0000\u0000\u0001\u0000\u0000\u0000\u0000\u0000\u0000\u0000\u0001\u0000\u0000\u0000\u0000\u0000\u0000\u0000\u0000\u0000\u0000\u0000\u0000\u0000\u0000\u0000\u0000\u0000\u0000\u0000ÿÿ\u0000\u0000\u0000\u0000\u0000\u0000", "PMU.034\u0000\u0000\u0000\u0000\u0000\u0000\u0000\u0000\u0000\u0000\"\u0000\u000f\u0000\u0006\u0000\u0003\u0000\u0001PZR.AI          PZR.BV          PZR.CI          PZR.AV          PZR.BI          PZR.CV          ANA1            ANA2            ANA3            DIG.stat1_01    DIG.stat1_02    DIG.stat1_03    DIG.stat1_04    DIG.stat1_05    DIG.stat1_06    DIG.stat1_07    DIG.stat1_08    DIG.stat1_09    DIG.stat1_10    DIG.stat1_11    DIG.stat1_12    DIG.stat1_13    DIG.stat1_14    DIG.stat1_15    DIG.stat1_16    \u0001\u0000\u0000\u0000\u0000\u0000\u0000\u0000\u0001\u0000\u0000\u0000\u0000\u0000\u0000\u0000\u0001\u0000\u0000\u0000\u0000\u0000\u0000\u0000\u0000\u0000\u0000\u0000\u0000\u0000\u0000\u0000\u0000\u0000\u0000\u0000ÿÿ\u0000\u0000\u0000\u0000\u0000\u0000", "PMU.035\u0000\u0000\u0000\u0000\u0000\u0000\u0000\u0000\u0000\u0000#\u0000\u000f\u0000\u0006\u0000\u0003\u0000\u0001PZR.AI          PZR.BV          PZR.CI          PZR.AV          PZR.BI          PZR.CV          ANA1            ANA2            ANA3            DIG.stat1_01    DIG.stat1_02    DIG.stat1_03    DIG.stat1_04    DIG.stat1_05    DIG.stat1_06    DIG.stat1_07    DIG.stat1_08    DIG.stat1_09    DIG.stat1_10    DIG.stat1_11    DIG.stat1_12    DIG.stat1_13    DIG.stat1_14    DIG.stat1_15    DIG.stat1_16    \u0001\u0000\u0000\u0000\u0000\u0000\u0000\u0000\u0001\u0000\u0000\u0000\u0000\u0000\u0000\u0000\u0001\u0000\u0000\u0000\u0000\u0000\u0000\u0000\u0000\u0000\u0000\u0000\u0000\u0000\u0000\u0000\u0000\u0000\u0000\u0000ÿÿ\u0000\u0000\u0000\u0000\u0000\u0000", "PMU.036\u0000\u0000\u0000\u0000\u0000\u0000\u0000\u0000\u0000\u0000$\u0000\u000f\u0000\u0006\u0000\u0003\u0000\u0001PZR.AI          PZR.BV          PZR.CI          PZR.AV          PZR.BI          PZR.CV          ANA1            ANA2            ANA3            DIG.stat1_01    DIG.stat1_02    DIG.stat1_03    DIG.stat1_04    DIG.stat1_05    DIG.stat1_06    DIG.stat1_07    DIG.stat1_08    DIG.stat1_09    DIG.stat1_10    DIG.stat1_11    DIG.stat1_12    DIG.stat1_13    DIG.stat1_14    DIG.stat1_15    DIG.stat1_16    \u0001\u0000\u0000\u0000\u0000\u0000\u0000\u0000\u0001\u0000\u0000\u0000\u0000\u0000\u0000\u0000\u0001\u0000\u0000\u0000\u0000\u0000\u0000\u0000\u0000\u0000\u0000\u0000\u0000\u0000\u0000\u0000\u0000\u0000\u0000\u0000ÿÿ\u0000\u0000\u0000\u0000\u0000\u0000", "PMU.037\u0000\u0000\u0000\u0000\u0000\u0000\u0000\u0000\u0000\u0000%\u0000\u000f\u0000\u0006\u0000\u0003\u0000\u0001PZR.AI          PZR.BV          PZR.CI          PZR.AV          PZR.BI          PZR.CV          ANA1            ANA2            ANA3            DIG.stat1_01    DIG.stat1_02    DIG.stat1_03    DIG.stat1_04    DIG.stat1_05    DIG.stat1_06    DIG.stat1_07    DIG.stat1_08    DIG.stat1_09    DIG.stat1_10    DIG.stat1_11    DIG.stat1_12    DIG.stat1_13    DIG.stat1_14    DIG.stat1_15    DIG.stat1_16    \u0001\u0000\u0000\u0000\u0000\u0000\u0000\u0000\u0001\u0000\u0000\u0000\u0000\u0000\u0000\u0000\u0001\u0000\u0000\u0000\u0000\u0000\u0000\u0000\u0000\u0000\u0000\u0000\u0000\u0000\u0000\u0000\u0000\u0000\u0000\u0000ÿÿ\u0000\u0000\u0000\u0000\u0000\u0000", "PMU.038\u0000\u0000\u0000\u0000\u0000\u0000\u0000\u0000\u0000\u0000&\u0000\u000f\u0000\u0006\u0000\u0003\u0000\u0001PZR.AI          PZR.BV          PZR.CI          PZR.AV          PZR.BI          PZR.CV          ANA1            ANA2            ANA3            DIG.stat1_01    DIG.stat1_02    DIG.stat1_03    DIG.stat1_04    DIG.stat1_05    DIG.stat1_06    DIG.stat1_07    DIG.stat1_08    DIG.stat1_09    DIG.stat1_10    DIG.stat1_11    DIG.stat1_12    DIG.stat1_13    DIG.stat1_14    DIG.stat1_15    DIG.stat1_16    \u0001\u0000\u0000\u0000\u0000\u0000\u0000\u0000\u0001\u0000\u0000\u0000\u0000\u0000\u0000\u0000\u0001\u0000\u0000\u0000\u0000\u0000\u0000\u0000\u0000\u0000\u0000\u0000\u0000\u0000\u0000\u0000\u0000\u0000\u0000\u0000ÿÿ\u0000\u0000\u0000\u0000\u0000\u0000", "PMU.039\u0000\u0000\u0000\u0000\u0000\u0000\u0000\u0000\u0000\u0000'\u0000\u000f\u0000\u0006\u0000\u0003\u0000\u0001PZR.AI          PZR.BV          PZR.CI          PZR.AV          PZR.BI          PZR.CV          ANA1            ANA2            ANA3            DIG.stat1_01    DIG.stat1_02    DIG.stat1_03    DIG.stat1_04    DIG.stat1_05    DIG.stat1_06    DIG.stat1_07    DIG.stat1_08    DIG.stat1_09    DIG.stat1_10    DIG.stat1_11    DIG.stat1_12    DIG.stat1_13    DIG.stat1_14    DIG.stat1_15    DIG.stat1_16    \u0001\u0000\u0000\u0000\u0000\u0000\u0000\u0000\u0001\u0000\u0000\u0000\u0000\u0000\u0000\u0000\u0001\u0000\u0000\u0000\u0000\u0000\u0000\u0000\u0000\u0000\u0000\u0000\u0000\u0000\u0000\u0000\u0000\u0000\u0000\u0000ÿÿ\u0000\u0000\u0000\u0000\u0000\u0000", "PMU.040\u0000\u0000\u0000\u0000\u0000\u0000\u0000\u0000\u0000\u0000(\u0000\u000f\u0000\u0006\u0000\u0003\u0000\u0001PZR.AI          PZR.BV          PZR.CI          PZR.AV          PZR.BI          PZR.CV          ANA1            ANA2            ANA3            DIG.stat1_01    DIG.stat1_02    DIG.stat1_03    DIG.stat1_04    DIG.stat1_05    DIG.stat1_06    DIG.stat1_07    DIG.stat1_08    DIG.stat1_09    DIG.stat1_10    DIG.stat1_11    DIG.stat1_12    DIG.stat1_13    DIG.stat1_14    DIG.stat1_15    DIG.stat1_16    \u0001\u0000\u0000\u0000\u0000\u0000\u0000\u0000\u0001\u0000\u0000\u0000\u0000\u0000\u0000\u0000\u0001\u0000\u0000\u0000\u0000\u0000\u0000\u0000\u0000\u0000\u0000\u0000\u0000\u0000\u0000\u0000\u0000\u0000\u0000\u0000ÿÿ\u0000\u0000\u0000\u0000\u0000\u0000", "PMU.041\u0000\u0000\u0000\u0000\u0000\u0000\u0000\u0000\u0000\u0000)\u0000\u000f\u0000\u0006\u0000\u0003\u0000\u0001PZR.AI          PZR.BV          PZR.CI          PZR.AV          PZR.BI          PZR.CV          ANA1            ANA2            ANA3            DIG.stat1_01    DIG.stat1_02    DIG.stat1_03    DIG.stat1_04    DIG.stat1_05    DIG.stat1_06    DIG.stat1_07    DIG.stat1_08    DIG.stat1_09    DIG.stat1_10    DIG.stat1_11    DIG.stat1_12    DIG.stat1_13    DIG.stat1_14    DIG.stat1_15    DIG.stat1_16    \u0001\u0000\u0000\u0000\u0000\u0000\u0000\u0000\u0001\u0000\u0000\u0000\u0000\u0000\u0000\u0000\u0001\u0000\u0000\u0000\u0000\u0000\u0000\u0000\u0000\u0000\u0000\u0000\u0000\u0000\u0000\u0000\u0000\u0000\u0000\u0000ÿÿ\u0000\u0000\u0000\u0000\u0000\u0000", "PMU.042\u0000\u0000\u0000\u0000\u0000\u0000\u0000\u0000\u0000\u0000*\u0000\u000f\u0000\u0006\u0000\u0003\u0000\u0001PZR.AI          PZR.BV          PZR.CI          PZR.AV          PZR.BI          PZR.CV          ANA1            ANA2            ANA3            DIG.stat1_01    DIG.stat1_02    DIG.stat1_03    DIG.stat1_04    DIG.stat1_05    DIG.stat1_06    DIG.stat1_07    DIG.stat1_08    DIG.stat1_09    DIG.stat1_10    DIG.stat1_11    DIG.stat1_12    DIG.stat1_13    DIG.stat1_14    DIG.stat1_15    DIG.stat1_16    \u0001\u0000\u0000\u0000\u0000\u0000\u0000\u0000\u0001\u0000\u0000\u0000\u0000\u0000\u0000\u0000\u0001\u0000\u0000\u0000\u0000\u0000\u0000\u0000\u0000\u0000\u0000\u0000\u0000\u0000\u0000\u0000\u0000\u0000\u0000\u0000ÿÿ\u0000\u0000\u0000\u0000\u0000\u0000", "PMU.043\u0000\u0000\u0000\u0000\u0000\u0000\u0000\u0000\u0000\u0000+\u0000\u000f\u0000\u0006\u0000\u0003\u0000\u0001PZR.AI          PZR.BV          PZR.CI          PZR.AV          PZR.BI          PZR.CV          ANA1            ANA2            ANA3            DIG.stat1_01    DIG.stat1_02    DIG.stat1_03    DIG.stat1_04    DIG.stat1_05    DIG.stat1_06    DIG.stat1_07    DIG.stat1_08    DIG.stat1_09    DIG.stat1_10    DIG.stat1_11    DIG.stat1_12    DIG.stat1_13    DIG.stat1_14    DIG.stat1_15    DIG.stat1_16    \u0001\u0000\u0000\u0000\u0000\u0000\u0000\u0000\u0001\u0000\u0000\u0000\u0000\u0000\u0000\u0000\u0001\u0000\u0000\u0000\u0000\u0000\u0000\u0000\u0000\u0000\u0000\u0000\u0000\u0000\u0000\u0000\u0000\u0000\u0000\u0000ÿÿ\u0000\u0000\u0000\u0000\u0000\u0000", "PMU.044\u0000\u0000\u0000\u0000\u0000\u0000\u0000\u0000\u0000\u0000,\u0000\u000f\u0000\u0006\u0000\u0003\u0000\u0001PZR.AI          PZR.BV          PZR.CI          PZR.AV          PZR.BI          PZR.CV          ANA1            ANA2            ANA3            DIG.stat1_01    DIG.stat1_02    DIG.stat1_03    DIG.stat1_04    DIG.stat1_05    DIG.stat1_06    DIG.stat1_07    DIG.stat1_08    DIG.stat1_09    DIG.stat1_10    DIG.stat1_11    DIG.stat1_12    DIG.stat1_13    DIG.stat1_14    DIG.stat1_15    DIG.stat1_16    \u0001\u0000\u0000\u0000\u0000\u0000\u0000\u0000\u0001\u0000\u0000\u0000\u0000\u0000\u0000\u0000\u0001\u0000\u0000\u0000\u0000\u0000\u0000\u0000\u0000\u0000\u0000\u0000\u0000\u0000\u0000\u0000\u0000\u0000\u0000\u0000ÿÿ\u0000\u0000\u0000\u0000\u0000\u0000", "PMU.045\u0000\u0000\u0000\u0000\u0000\u0000\u0000\u0000\u0000\u0000-\u0000\u000f\u0000\u0006\u0000\u0003\u0000\u0001PZR.AI          PZR.BV          PZR.CI          PZR.AV          PZR.BI          PZR.CV          ANA1            ANA2            ANA3            DIG.stat1_01    DIG.stat1_02    DIG.stat1_03    DIG.stat1_04    DIG.stat1_05    DIG.stat1_06    DIG.stat1_07    DIG.stat1_08    DIG.stat1_09    DIG.stat1_10    DIG.stat1_11    DIG.stat1_12    DIG.stat1_13    DIG.stat1_14    DIG.stat1_15    DIG.stat1_16    \u0001\u0000\u0000\u0000\u0000\u0000\u0000\u0000\u0001\u0000\u0000\u0000\u0000\u0000\u0000\u0000\u0001\u0000\u0000\u0000\u0000\u0000\u0000\u0000\u0000\u0000\u0000\u0000\u0000\u0000\u0000\u0000\u0000\u0000\u0000\u0000ÿÿ\u0000\u0000\u0000\u0000\u0000\u0000", "PMU.046\u0000\u0000\u0000\u0000\u0000\u0000\u0000\u0000\u0000\u0000.\u0000\u000f\u0000\u0006\u0000\u0003\u0000\u0001PZR.AI          PZR.BV          PZR.CI          PZR.AV          PZR.BI          PZR.CV          ANA1            ANA2            ANA3            DIG.stat1_01    DIG.stat1_02    DIG.stat1_03    DIG.stat1_04    DIG.stat1_05    DIG.stat1_06    DIG.stat1_07    DIG.stat1_08    DIG.stat1_09    DIG.stat1_10    DIG.stat1_11    DIG.stat1_12    DIG.stat1_13    DIG.stat1_14    DIG.stat1_15    DIG.stat1_16    \u0001\u0000\u0000\u0000\u0000\u0000\u0000\u0000\u0001\u0000\u0000\u0000\u0000\u0000\u0000\u0000\u0001\u0000\u0000\u0000\u0000\u0000\u0000\u0000\u0000\u0000\u0000\u0000\u0000\u0000\u0000\u0000\u0000\u0000\u0000\u0000ÿÿ\u0000\u0000\u0000\u0000\u0000\u0000", "PMU.047\u0000\u0000\u0000\u0000\u0000\u0000\u0000\u0000\u0000\u0000/\u0000\u000f\u0000\u0006\u0000\u0003\u0000\u0001PZR.AI          PZR.BV          PZR.CI          PZR.AV          PZR.BI          PZR.CV          ANA1            ANA2            ANA3            DIG.stat1_01    DIG.stat1_02    DIG.stat1_03    DIG.stat1_04    DIG.stat1_05    DIG.stat1_06    DIG.stat1_07    DIG.stat1_08    DIG.stat1_09    DIG.stat1_10    DIG.stat1_11    DIG.stat1_12    DIG.stat1_13    DIG.stat1_14    DIG.stat1_15    DIG.stat1_16    \u0001\u0000\u0000\u0000\u0000\u0000\u0000\u0000\u0001\u0000\u0000\u0000\u0000\u0000\u0000\u0000\u0001\u0000\u0000\u0000\u0000\u0000\u0000\u0000\u0000\u0000\u0000\u0000\u0000\u0000\u0000\u0000\u0000\u0000\u0000\u0000ÿÿ\u0000\u0000\u0000\u0000\u0000\u0000", "PMU.048\u0000\u0000\u0000\u0000\u0000\u0000\u0000\u0000\u0000\u00000\u0000\u000f\u0000\u0006\u0000\u0003\u0000\u0001PZR.AI          PZR.BV          PZR.CI          PZR.AV          PZR.BI          PZR.CV          ANA1            ANA2            ANA3            DIG.stat1_01    DIG.stat1_02    DIG.stat1_03    DIG.stat1_04    DIG.stat1_05    DIG.stat1_06    DIG.stat1_07    DIG.stat1_08    DIG.stat1_09    DIG.stat1_10    DIG.stat1_11    DIG.stat1_12    DIG.stat1_13    DIG.stat1_14    DIG.stat1_15    DIG.stat1_16    \u0001\u0000\u0000\u0000\u0000\u0000\u0000\u0000\u0001\u0000\u0000\u0000\u0000\u0000\u0000\u0000\u0001\u0000\u0000\u0000\u0000\u0000\u0000\u0000\u0000\u0000\u0000\u0000\u0000\u0000\u0000\u0000\u0000\u0000\u0000\u0000ÿÿ\u0000\u0000\u0000\u0000\u0000\u0000", "PMU.049\u0000\u0000\u0000\u0000\u0000\u0000\u0000\u0000\u0000\u00001\u0000\u000f\u0000\u0006\u0000\u0003\u0000\u0001PZR.AI          PZR.BV          PZR.CI          PZR.AV          PZR.BI          PZR.CV          ANA1            ANA2            ANA3            DIG.stat1_01    DIG.stat1_02    DIG.stat1_03    DIG.stat1_04    DIG.stat1_05    DIG.stat1_06    DIG.stat1_07    DIG.stat1_08    DIG.stat1_09    DIG.stat1_10    DIG.stat1_11    DIG.stat1_12    DIG.stat1_13    DIG.stat1_14    DIG.stat1_15    DIG.stat1_16    \u0001\u0000\u0000\u0000\u0000\u0000\u0000\u0000\u0001\u0000\u0000\u0000\u0000\u0000\u0000\u0000\u0001\u0000\u0000\u0000\u0000\u0000\u0000\u0000\u0000\u0000\u0000\u0000\u0000\u0000\u0000\u0000\u0000\u0000\u0000\u0000ÿÿ\u0000\u0000\u0000\u0000\u0000\u0000", "PMU.050\u0000\u0000\u0000\u0000\u0000\u0000\u0000\u0000\u0000\u00002\u0000\u000f\u0000\u0006\u0000\u0003\u0000\u0001PZR.AI          PZR.BV          PZR.CI          PZR.AV          PZR.BI          PZR.CV          ANA1            ANA2            ANA3            DIG.stat1_01    DIG.stat1_02    DIG.stat1_03    DIG.stat1_04    DIG.stat1_05    DIG.stat1_06    DIG.stat1_07    DIG.stat1_08    DIG.stat1_09    DIG.stat1_10    DIG.stat1_11    DIG.stat1_12    DIG.stat1_13    DIG.stat1_14    DIG.stat1_15    DIG.stat1_16    \u0001\u0000\u0000\u0000\u0000\u0000\u0000\u0000\u0001\u0000\u0000\u0000\u0000\u0000\u0000\u0000\u0001\u0000\u0000\u0000\u0000\u0000\u0000\u0000\u0000\u0000\u0000\u0000\u0000\u0000\u0000\u0000\u0000\u0000\u0000\u0000ÿÿ\u0000\u0000\u0000\u0000\u0000\u0000", "PMU.051\u0000\u0000\u0000\u0000\u0000\u0000\u0000\u0000\u0000\u00003\u0000\u000f\u0000\u0006\u0000\u0003\u0000\u0001PZR.AI          PZR.BV          PZR.CI          PZR.AV          PZR.BI          PZR.CV          ANA1            ANA2            ANA3            DIG.stat1_01    DIG.stat1_02    DIG.stat1_03    DIG.stat1_04    DIG.stat1_05    DIG.stat1_06    DIG.stat1_07    DIG.stat1_08    DIG.stat1_09    DIG.stat1_10    DIG.stat1_11    DIG.stat1_12    DIG.stat1_13    DIG.stat1_14    DIG.stat1_15    DIG.stat1_16    \u0001\u0000\u0000\u0000\u0000\u0000\u0000\u0000\u0001\u0000\u0000\u0000\u0000\u0000\u0000\u0000\u0001\u0000\u0000\u0000\u0000\u0000\u0000\u0000\u0000\u0000\u0000\u0000\u0000\u0000\u0000\u0000\u0000\u0000\u0000\u0000ÿÿ\u0000\u0000\u0000\u0000\u0000\u0000", "PMU.052\u0000\u0000\u0000\u0000\u0000\u0000\u0000\u0000\u0000\u00004\u0000\u000f\u0000\u0006\u0000\u0003\u0000\u0001PZR.AI          PZR.BV          PZR.CI          PZR.AV          PZR.BI          PZR.CV          ANA1            ANA2            ANA3            DIG.stat1_01    DIG.stat1_02    DIG.stat1_03    DIG.stat1_04    DIG.stat1_05    DIG.stat1_06    DIG.stat1_07    DIG.stat1_08    DIG.stat1_09    DIG.stat1_10    DIG.stat1_11    DIG.stat1_12    DIG.stat1_13    DIG.stat1_14    DIG.stat1_15    DIG.stat1_16    \u0001\u0000\u0000\u0000\u0000\u0000\u0000\u0000\u0001\u0000\u0000\u0000\u0000\u0000\u0000\u0000\u0001\u0000\u0000\u0000\u0000\u0000\u0000\u0000\u0000\u0000\u0000\u0000\u0000\u0000\u0000\u0000\u0000\u0000\u0000\u0000ÿÿ\u0000\u0000\u0000\u0000\u0000\u0000", "PMU.053\u0000\u0000\u0000\u0000\u0000\u0000\u0000\u0000\u0000\u00005\u0000\u000f\u0000\u0006\u0000\u0003\u0000\u0001PZR.AI          PZR.BV          PZR.CI          PZR.AV          PZR.BI          PZR.CV          ANA1            ANA2            ANA3            DIG.stat1_01    DIG.stat1_02    DIG.stat1_03    DIG.stat1_04    DIG.stat1_05    DIG.stat1_06    DIG.stat1_07    DIG.stat1_08    DIG.stat1_09    DIG.stat1_10    DIG.stat1_11    DIG.stat1_12    DIG.stat1_13    DIG.stat1_14    DIG.stat1_15    DIG.stat1_16    \u0001\u0000\u0000\u0000\u0000\u0000\u0000\u0000\u0001\u0000\u0000\u0000\u0000\u0000\u0000\u0000\u0001\u0000\u0000\u0000\u0000\u0000\u0000\u0000\u0000\u0000\u0000\u0000\u0000\u0000\u0000\u0000\u0000\u0000\u0000\u0000ÿÿ\u0000\u0000\u0000\u0000\u0000\u0000", "PMU.054\u0000\u0000\u0000\u0000\u0000\u0000\u0000\u0000\u0000\u00006\u0000\u000f\u0000\u0006\u0000\u0003\u0000\u0001PZR.AI          PZR.BV          PZR.CI          PZR.AV          PZR.BI          PZR.CV          ANA1            ANA2            ANA3            DIG.stat1_01    DIG.stat1_02    DIG.stat1_03    DIG.stat1_04    DIG.stat1_05    DIG.stat1_06    DIG.stat1_07    DIG.stat1_08    DIG.stat1_09    DIG.stat1_10    DIG.stat1_11    DIG.stat1_12    DIG.stat1_13    DIG.stat1_14    DIG.stat1_15    DIG.stat1_16    \u0001\u0000\u0000\u0000\u0000\u0000\u0000\u0000\u0001\u0000\u0000\u0000\u0000\u0000\u0000\u0000\u0001\u0000\u0000\u0000\u0000\u0000\u0000\u0000\u0000\u0000\u0000\u0000\u0000\u0000\u0000\u0000\u0000\u0000\u0000\u0000ÿÿ\u0000\u0000\u0000\u0000\u0000\u0000", "PMU.055\u0000\u0000\u0000\u0000\u0000\u0000\u0000\u0000\u0000\u00007\u0000\u000f\u0000\u0006\u0000\u0003\u0000\u0001PZR.AI          PZR.BV          PZR.CI          PZR.AV          PZR.BI          PZR.CV          ANA1            ANA2            ANA3            DIG.stat1_01    DIG.stat1_02    DIG.stat1_03    DIG.stat1_04    DIG.stat1_05    DIG.stat1_06    DIG.stat1_07    DIG.stat1_08    DIG.stat1_09    DIG.stat1_10    DIG.stat1_11    DIG.stat1_12    DIG.stat1_13    DIG.stat1_14    DIG.stat1_15    DIG.stat1_16    \u0001\u0000\u0000\u0000\u0000\u0000\u0000\u0000\u0001\u0000\u0000\u0000\u0000\u0000\u0000\u0000\u0001\u0000\u0000\u0000\u0000\u0000\u0000\u0000\u0000\u0000\u0000\u0000\u0000\u0000\u0000\u0000\u0000\u0000\u0000\u0000ÿÿ\u0000\u0000\u0000\u0000\u0000\u0000", "PMU.056\u0000\u0000\u0000\u0000\u0000\u0000\u0000\u0000\u0000\u00008\u0000\u000f\u0000\u0006\u0000\u0003\u0000\u0001PZR.AI          PZR.BV          PZR.CI          PZR.AV          PZR.BI          PZR.CV          ANA1            ANA2            ANA3            DIG.stat1_01    DIG.stat1_02    DIG.stat1_03    DIG.stat1_04    DIG.stat1_05    DIG.stat1_06    DIG.stat1_07    DIG.stat1_08    DIG.stat1_09    DIG.stat1_10    DIG.stat1_11    DIG.stat1_12    DIG.stat1_13    DIG.stat1_14    DIG.stat1_15    DIG.stat1_16    \u0001\u0000\u0000\u0000\u0000\u0000\u0000\u0000\u0001\u0000\u0000\u0000\u0000\u0000\u0000\u0000\u0001\u0000\u0000\u0000\u0000\u0000\u0000\u0000\u0000\u0000\u0000\u0000\u0000\u0000\u0000\u0000\u0000\u0000\u0000\u0000ÿÿ\u0000\u0000\u0000\u0000\u0000\u0000", "PMU.057\u0000\u0000\u0000\u0000\u0000\u0000\u0000\u0000\u0000\u00009\u0000\u000f\u0000\u0006\u0000\u0003\u0000\u0001PZR.AI          PZR.BV          PZR.CI          PZR.AV          PZR.BI          PZR.CV          ANA1            ANA2            ANA3            DIG.stat1_01    DIG.stat1_02    DIG.stat1_03    DIG.stat1_04    DIG.stat1_05    DIG.stat1_06    DIG.stat1_07    DIG.stat1_08    DIG.stat1_09    DIG.stat1_10    DIG.stat1_11    DIG.stat1_12    DIG.stat1_13    DIG.stat1_14    DIG.stat1_15    DIG.stat1_16    \u0001\u0000\u0000\u0000\u0000\u0000\u0000\u0000\u0001\u0000\u0000\u0000\u0000\u0000\u0000\u0000\u0001\u0000\u0000\u0000\u0000\u0000\u0000\u0000\u0000\u0000\u0000\u0000\u0000\u0000\u0000\u0000\u0000\u0000\u0000\u0000ÿÿ\u0000\u0000\u0000\u0000\u0000\u0000", "PMU.058\u0000\u0000\u0000\u0000\u0000\u0000\u0000\u0000\u0000\u0000:\u0000\u000f\u0000\u0006\u0000\u0003\u0000\u0001PZR.AI          PZR.BV          PZR.CI          PZR.AV          PZR.BI          PZR.CV          ANA1            ANA2            ANA3            DIG.stat1_01    DIG.stat1_02    DIG.stat1_03    DIG.stat1_04    DIG.stat1_05    DIG.stat1_06    DIG.stat1_07    DIG.stat1_08    DIG.stat1_09    DIG.stat1_10    DIG.stat1_11    DIG.stat1_12    DIG.stat1_13    DIG.stat1_14    DIG.stat1_15    DIG.stat1_16    \u0001\u0000\u0000\u0000\u0000\u0000\u0000\u0000\u0001\u0000\u0000\u0000\u0000\u0000\u0000\u0000\u0001\u0000\u0000\u0000\u0000\u0000\u0000\u0000\u0000\u0000\u0000\u0000\u0000\u0000\u0000\u0000\u0000\u0000\u0000\u0000ÿÿ\u0000\u0000\u0000\u0000\u0000\u0000", "PMU.059\u0000\u0000\u0000\u0000\u0000\u0000\u0000\u0000\u0000\u0000;\u0000\u000f\u0000\u0006\u0000\u0003\u0000\u0001PZR.AI          PZR.BV          PZR.CI          PZR.AV          PZR.BI          PZR.CV          ANA1            ANA2            ANA3            DIG.stat1_01    DIG.stat1_02    DIG.stat1_03    DIG.stat1_04    DIG.stat1_05    DIG.stat1_06    DIG.stat1_07    DIG.stat1_08    DIG.stat1_09    DIG.stat1_10    DIG.stat1_11    DIG.stat1_12    DIG.stat1_13    DIG.stat1_14    DIG.stat1_15    DIG.stat1_16    \u0001\u0000\u0000\u0000\u0000\u0000\u0000\u0000\u0001\u0000\u0000\u0000\u0000\u0000\u0000\u0000\u0001\u0000\u0000\u0000\u0000\u0000\u0000\u0000\u0000\u0000\u0000\u0000\u0000\u0000\u0000\u0000\u0000\u0000\u0000\u0000ÿÿ\u0000\u0000\u0000\u0000\u0000\u0000", "PMU.060\u0000\u0000\u0000\u0000\u0000\u0000\u0000\u0000\u0000\u0000<\u0000\u000f\u0000\u0006\u0000\u0003\u0000\u0001PZR.AI          PZR.BV          PZR.CI          PZR.AV          PZR.BI          PZR.CV          ANA1            ANA2            ANA3            DIG.stat1_01    DIG.stat1_02    DIG.stat1_03    DIG.stat1_04    DIG.stat1_05    DIG.stat1_06    DIG.stat1_07    DIG.stat1_08    DIG.stat1_09    DIG.stat1_10    DIG.stat1_11    DIG.stat1_12    DIG.stat1_13    DIG.stat1_14    DIG.stat1_15    DIG.stat1_16    \u0001\u0000\u0000\u0000\u0000\u0000\u0000\u0000\u0001\u0000\u0000\u0000\u0000\u0000\u0000\u0000\u0001\u0000\u0000\u0000\u0000\u0000\u0000\u0000\u0000\u0000\u0000\u0000\u0000\u0000\u0000\u0000\u0000\u0000\u0000\u0000ÿÿ\u0000\u0000\u0000\u0000\u0000\u0000", "PMU.061\u0000\u0000\u0000\u0000\u0000\u0000\u0000\u0000\u0000\u0000=\u0000\u000f\u0000\u0006\u0000\u0003\u0000\u0001PZR.AI          PZR.BV          PZR.CI          PZR.AV          PZR.BI          PZR.CV          ANA1            ANA2            ANA3            DIG.stat1_01    DIG.stat1_02    DIG.stat1_03    DIG.stat1_04    DIG.stat1_05    DIG.stat1_06    DIG.stat1_07    DIG.stat1_08    DIG.stat1_09    DIG.stat1_10    DIG.stat1_11    DIG.stat1_12    DIG.stat1_13    DIG.stat1_14    DIG.stat1_15    DIG.stat1_16    \u0001\u0000\u0000\u0000\u0000\u0000\u0000\u0000\u0001\u0000\u0000\u0000\u0000\u0000\u0000\u0000\u0001\u0000\u0000\u0000\u0000\u0000\u0000\u0000\u0000\u0000\u0000\u0000\u0000\u0000\u0000\u0000\u0000\u0000\u0000\u0000ÿÿ\u0000\u0000\u0000\u0000\u0000\u0000", "PMU.062\u0000\u0000\u0000\u0000\u0000\u0000\u0000\u0000\u0000\u0000>\u0000\u000f\u0000\u0006\u0000\u0003\u0000\u0001PZR.AI          PZR.BV          PZR.CI          PZR.AV          PZR.BI          PZR.CV          ANA1            ANA2            ANA3            DIG.stat1_01    DIG.stat1_02    DIG.stat1_03    DIG.stat1_04    DIG.stat1_05    DIG.stat1_06    DIG.stat1_07    DIG.stat1_08    DIG.stat1_09    DIG.stat1_10    DIG.stat1_11    DIG.stat1_12    DIG.stat1_13    DIG.stat1_14    DIG.stat1_15    DIG.stat1_16    \u0001\u0000\u0000\u0000\u0000\u0000\u0000\u0000\u0001\u0000\u0000\u0000\u0000\u0000\u0000\u0000\u0001\u0000\u0000\u0000\u0000\u0000\u0000\u0000\u0000\u0000\u0000\u0000\u0000\u0000\u0000\u0000\u0000\u0000\u0000\u0000ÿÿ\u0000\u0000\u0000\u0000\u0000\u0000", "PMU.063\u0000\u0000\u0000\u0000\u0000\u0000\u0000\u0000\u0000\u0000?\u0000\u000f\u0000\u0006\u0000\u0003\u0000\u0001PZR.AI          PZR.BV          PZR.CI          PZR.AV          PZR.BI          PZR.CV          ANA1            ANA2            ANA3            DIG.stat1_01    DIG.stat1_02    DIG.stat1_03    DIG.stat1_04    DIG.stat1_05    DIG.stat1_06    DIG.stat1_07    DIG.stat1_08    DIG.stat1_09    DIG.stat1_10    DIG.stat1_11    DIG.stat1_12    DIG.stat1_13    DIG.stat1_14    DIG.stat1_15    DIG.stat1_16    \u0001\u0000\u0000\u0000\u0000\u0000\u0000\u0000\u0001\u0000\u0000\u0000\u0000\u0000\u0000\u0000\u0001\u0000\u0000\u0000\u0000\u0000\u0000\u0000\u0000\u0000\u0000\u0000\u0000\u0000\u0000\u0000\u0000\u0000\u0000\u0000ÿÿ\u0000\u0000\u0000\u0000\u0000\u0000", "PMU.064\u0000\u0000\u0000\u0000\u0000\u0000\u0000\u0000\u0000\u0000@\u0000\u000f\u0000\u0006\u0000\u0003\u0000\u0001PZR.AI          PZR.BV          PZR.CI          PZR.AV          PZR.BI          PZR.CV          ANA1            ANA2            ANA3            DIG.stat1_01    DIG.stat1_02    DIG.stat1_03    DIG.stat1_04    DIG.stat1_05    DIG.stat1_06    DIG.stat1_07    DIG.stat1_08    DIG.stat1_09    DIG.stat1_10    DIG.stat1_11    DIG.stat1_12    DIG.stat1_13    DIG.stat1_14    DIG.stat1_15    DIG.stat1_16    \u0001\u0000\u0000\u0000\u0000\u0000\u0000\u0000\u0001\u0000\u0000\u0000\u0000\u0000\u0000\u0000\u0001\u0000\u0000\u0000\u0000\u0000\u0000\u0000\u0000\u0000\u0000\u0000\u0000\u0000\u0000\u0000\u0000\u0000\u0000\u0000ÿÿ\u0000\u0000\u0000\u0000\u0000\u0000", "PMU.065\u0000\u0000\u0000\u0000\u0000\u0000\u0000\u0000\u0000\u0000A\u0000\u000f\u0000\u0006\u0000\u0003\u0000\u0001PZR.AI          PZR.BV          PZR.CI          PZR.AV          PZR.BI          PZR.CV          ANA1            ANA2            ANA3            DIG.stat1_01    DIG.stat1_02    DIG.stat1_03    DIG.stat1_04    DIG.stat1_05    DIG.stat1_06    DIG.stat1_07    DIG.stat1_08    DIG.stat1_09    DIG.stat1_10    DIG.stat1_11    DIG.stat1_12    DIG.stat1_13    DIG.stat1_14    DIG.stat1_15    DIG.stat1_16    \u0001\u0000\u0000\u0000\u0000\u0000\u0000\u0000\u0001\u0000\u0000\u0000\u0000\u0000\u0000\u0000\u0001\u0000\u0000\u0000\u0000\u0000\u0000\u0000\u0000\u0000\u0000\u0000\u0000\u0000\u0000\u0000\u0000\u0000\u0000\u0000ÿÿ\u0000\u0000\u0000\u0000\u0000\u0000", "PMU.066\u0000\u0000\u0000\u0000\u0000\u0000\u0000\u0000\u0000\u0000B\u0000\u000f\u0000\u0006\u0000\u0003\u0000\u0001PZR.AI          PZR.BV          PZR.CI          PZR.AV          PZR.BI          PZR.CV          ANA1            ANA2            ANA3            DIG.stat1_01    DIG.stat1_02    DIG.stat1_03    DIG.stat1_04    DIG.stat1_05    DIG.stat1_06    DIG.stat1_07    DIG.stat1_08    DIG.stat1_09    DIG.stat1_10    DIG.stat1_11    DIG.stat1_12    DIG.stat1_13    DIG.stat1_14    DIG.stat1_15    DIG.stat1_16    \u0001\u0000\u0000\u0000\u0000\u0000\u0000\u0000\u0001\u0000\u0000\u0000\u0000\u0000\u0000\u0000\u0001\u0000\u0000\u0000\u0000\u0000\u0000\u0000\u0000\u0000\u0000\u0000\u0000\u0000\u0000\u0000\u0000\u0000\u0000\u0000ÿÿ\u0000\u0000\u0000\u0000\u0000\u0000", "PMU.067\u0000\u0000\u0000\u0000\u0000\u0000\u0000\u0000\u0000\u0000C\u0000\u000f\u0000\u0006\u0000\u0003\u0000\u0001PZR.AI          PZR.BV          PZR.CI          PZR.AV          PZR.BI          PZR.CV          ANA1            ANA2            ANA3            DIG.stat1_01    DIG.stat1_02    DIG.stat1_03    DIG.stat1_04    DIG.stat1_05    DIG.stat1_06    DIG.stat1_07    DIG.stat1_08    DIG.stat1_09    DIG.stat1_10    DIG.stat1_11    DIG.stat1_12    DIG.stat1_13    DIG.stat1_14    DIG.stat1_15    DIG.stat1_16    \u0001\u0000\u0000\u0000\u0000\u0000\u0000\u0000\u0001\u0000\u0000\u0000\u0000\u0000\u0000\u0000\u0001\u0000\u0000\u0000\u0000\u0000\u0000\u0000\u0000\u0000\u0000\u0000\u0000\u0000\u0000\u0000\u0000\u0000\u0000\u0000ÿÿ\u0000\u0000\u0000\u0000\u0000\u0000", "PMU.068\u0000\u0000\u0000\u0000\u0000\u0000\u0000\u0000\u0000\u0000D\u0000\u000f\u0000\u0006\u0000\u0003\u0000\u0001PZR.AI          PZR.BV          PZR.CI          PZR.AV          PZR.BI          PZR.CV          ANA1            ANA2            ANA3            DIG.stat1_01    DIG.stat1_02    DIG.stat1_03    DIG.stat1_04    DIG.stat1_05    DIG.stat1_06    DIG.stat1_07    DIG.stat1_08    DIG.stat1_09    DIG.stat1_10    DIG.stat1_11    DIG.stat1_12    DIG.stat1_13    DIG.stat1_14    DIG.stat1_15    DIG.stat1_16    \u0001\u0000\u0000\u0000\u0000\u0000\u0000\u0000\u0001\u0000\u0000\u0000\u0000\u0000\u0000\u0000\u0001\u0000\u0000\u0000\u0000\u0000\u0000\u0000\u0000\u0000\u0000\u0000\u0000\u0000\u0000\u0000\u0000\u0000\u0000\u0000ÿÿ\u0000\u0000\u0000\u0000\u0000\u0000", "PMU.069\u0000\u0000\u0000\u0000\u0000\u0000\u0000\u0000\u0000\u0000E\u0000\u000f\u0000\u0006\u0000\u0003\u0000\u0001PZR.AI          PZR.BV          PZR.CI          PZR.AV          PZR.BI          PZR.CV          ANA1            ANA2            ANA3            DIG.stat1_01    DIG.stat1_02    DIG.stat1_03    DIG.stat1_04    DIG.stat1_05    DIG.stat1_06    DIG.stat1_07    DIG.stat1_08    DIG.stat1_09    DIG.stat1_10    DIG.stat1_11    DIG.stat1_12    DIG.stat1_13    DIG.stat1_14    DIG.stat1_15    DIG.stat1_16    \u0001\u0000\u0000\u0000\u0000\u0000\u0000\u0000\u0001\u0000\u0000\u0000\u0000\u0000\u0000\u0000\u0001\u0000\u0000\u0000\u0000\u0000\u0000\u0000\u0000\u0000\u0000\u0000\u0000\u0000\u0000\u0000\u0000\u0000\u0000\u0000ÿÿ\u0000\u0000\u0000\u0000\u0000\u0000", "PMU.070\u0000\u0000\u0000\u0000\u0000\u0000\u0000\u0000\u0000\u0000F\u0000\u000f\u0000\u0006\u0000\u0003\u0000\u0001PZR.AI          PZR.BV          PZR.CI          PZR.AV          PZR.BI          PZR.CV          ANA1            ANA2            ANA3            DIG.stat1_01    DIG.stat1_02    DIG.stat1_03    DIG.stat1_04    DIG.stat1_05    DIG.stat1_06    DIG.stat1_07    DIG.stat1_08    DIG.stat1_09    DIG.stat1_10    DIG.stat1_11    DIG.stat1_12    DIG.stat1_13    DIG.stat1_14    DIG.stat1_15    DIG.stat1_16    \u0001\u0000\u0000\u0000\u0000\u0000\u0000\u0000\u0001\u0000\u0000\u0000\u0000\u0000\u0000\u0000\u0001\u0000\u0000\u0000\u0000\u0000\u0000\u0000\u0000\u0000\u0000\u0000\u0000\u0000\u0000\u0000\u0000\u0000\u0000\u0000ÿÿ\u0000\u0000\u0000\u0000\u0000\u0000", "PMU.071\u0000\u0000\u0000\u0000\u0000\u0000\u0000\u0000\u0000\u0000G\u0000\u000f\u0000\u0006\u0000\u0003\u0000\u0001PZR.AI          PZR.BV          PZR.CI          PZR.AV          PZR.BI          PZR.CV          ANA1            ANA2            ANA3            DIG.stat1_01    DIG.stat1_02    DIG.stat1_03    DIG.stat1_04    DIG.stat1_05    DIG.stat1_06    DIG.stat1_07    DIG.stat1_08    DIG.stat1_09    DIG.stat1_10    DIG.stat1_11    DIG.stat1_12    DIG.stat1_13    DIG.stat1_14    DIG.stat1_15    DIG.stat1_16    \u0001\u0000\u0000\u0000\u0000\u0000\u0000\u0000\u0001\u0000\u0000\u0000\u0000\u0000\u0000\u0000\u0001\u0000\u0000\u0000\u0000\u0000\u0000\u0000\u0000\u0000\u0000\u0000\u0000\u0000\u0000\u0000\u0000\u0000\u0000\u0000ÿÿ\u0000\u0000\u0000\u0000\u0000\u0000", "PMU.072\u0000\u0000\u0000\u0000\u0000\u0000\u0000\u0000\u0000\u0000H\u0000\u000f\u0000\u0006\u0000\u0003\u0000\u0001PZR.AI          PZR.BV          PZR.CI          PZR.AV          PZR.BI          PZR.CV          ANA1            ANA2            ANA3            DIG.stat1_01    DIG.stat1_02    DIG.stat1_03    DIG.stat1_04    DIG.stat1_05    DIG.stat1_06    DIG.stat1_07    DIG.stat1_08    DIG.stat1_09    DIG.stat1_10    DIG.stat1_11    DIG.stat1_12    DIG.stat1_13    DIG.stat1_14    DIG.stat1_15    DIG.stat1_16    \u0001\u0000\u0000\u0000\u0000\u0000\u0000\u0000\u0001\u0000\u0000\u0000\u0000\u0000\u0000\u0000\u0001\u0000\u0000\u0000\u0000\u0000\u0000\u0000\u0000\u0000\u0000\u0000\u0000\u0000\u0000\u0000\u0000\u0000\u0000\u0000ÿÿ\u0000\u0000\u0000\u0000\u0000\u0000", "PMU.073\u0000\u0000\u0000\u0000\u0000\u0000\u0000\u0000\u0000\u0000I\u0000\u000f\u0000\u0006\u0000\u0003\u0000\u0001PZR.AI          PZR.BV          PZR.CI          PZR.AV          PZR.BI          PZR.CV          ANA1            ANA2            ANA3            DIG.stat1_01    DIG.stat1_02    DIG.stat1_03    DIG.stat1_04    DIG.stat1_05    DIG.stat1_06    DIG.stat1_07    DIG.stat1_08    DIG.stat1_09    DIG.stat1_10    DIG.stat1_11    DIG.stat1_12    DIG.stat1_13    DIG.stat1_14    DIG.stat1_15    DIG.stat1_16    \u0001\u0000\u0000\u0000\u0000\u0000\u0000\u0000\u0001\u0000\u0000\u0000\u0000\u0000\u0000\u0000\u0001\u0000\u0000\u0000\u0000\u0000\u0000\u0000\u0000\u0000\u0000\u0000\u0000\u0000\u0000\u0000\u0000\u0000\u0000\u0000ÿÿ\u0000\u0000\u0000\u0000\u0000\u0000", "PMU.074\u0000\u0000\u0000\u0000\u0000\u0000\u0000\u0000\u0000\u0000J\u0000\u000f\u0000\u0006\u0000\u0003\u0000\u0001PZR.AI          PZR.BV          PZR.CI          PZR.AV          PZR.BI          PZR.CV          ANA1            ANA2            ANA3            DIG.stat1_01    DIG.stat1_02    DIG.stat1_03    DIG.stat1_04    DIG.stat1_05    DIG.stat1_06    DIG.stat1_07    DIG.stat1_08    DIG.stat1_09    DIG.stat1_10    DIG.stat1_11    DIG.stat1_12    DIG.stat1_13    DIG.stat1_14    DIG.stat1_15    DIG.stat1_16    \u0001\u0000\u0000\u0000\u0000\u0000\u0000\u0000\u0001\u0000\u0000\u0000\u0000\u0000\u0000\u0000\u0001\u0000\u0000\u0000\u0000\u0000\u0000\u0000\u0000\u0000\u0000\u0000\u0000\u0000\u0000\u0000\u0000\u0000\u0000\u0000ÿÿ\u0000\u0000\u0000\u0000\u0000\u0000", "PMU.075\u0000\u0000\u0000\u0000\u0000\u0000\u0000\u0000\u0000\u0000K\u0000\u000f\u0000\u0006\u0000\u0003\u0000\u0001PZR.AI          PZR.BV          PZR.CI          PZR.AV          PZR.BI          PZR.CV          ANA1            ANA2            ANA3            DIG.stat1_01    DIG.stat1_02    DIG.stat1_03    DIG.stat1_04    DIG.stat1_05    DIG.stat1_06    DIG.stat1_07    DIG.stat1_08    DIG.stat1_09    DIG.stat1_10    DIG.stat1_11    DIG.stat1_12    DIG.stat1_13    DIG.stat1_14    DIG.stat1_15    DIG.stat1_16    \u0001\u0000\u0000\u0000\u0000\u0000\u0000\u0000\u0001\u0000\u0000\u0000\u0000\u0000\u0000\u0000\u0001\u0000\u0000\u0000\u0000\u0000\u0000\u0000\u0000\u0000\u0000\u0000\u0000\u0000\u0000\u0000\u0000\u0000\u0000\u0000ÿÿ\u0000\u0000\u0000\u0000\u0000\u0000", "PMU.076\u0000\u0000\u0000\u0000\u0000\u0000\u0000\u0000\u0000\u0000L\u0000\u000f\u0000\u0006\u0000\u0003\u0000\u0001PZR.AI          PZR.BV          PZR.CI          PZR.AV          PZR.BI          PZR.CV          ANA1            ANA2            ANA3            DIG.stat1_01    DIG.stat1_02    DIG.stat1_03    DIG.stat1_04    DIG.stat1_05    DIG.stat1_06    DIG.stat1_07    DIG.stat1_08    DIG.stat1_09    DIG.stat1_10    DIG.stat1_11    DIG.stat1_12    DIG.stat1_13    DIG.stat1_14    DIG.stat1_15    DIG.stat1_16    \u0001\u0000\u0000\u0000\u0000\u0000\u0000\u0000\u0001\u0000\u0000\u0000\u0000\u0000\u0000\u0000\u0001\u0000\u0000\u0000\u0000\u0000\u0000\u0000\u0000\u0000\u0000\u0000\u0000\u0000\u0000\u0000\u0000\u0000\u0000\u0000ÿÿ\u0000\u0000\u0000\u0000\u0000\u0000", "PMU.077\u0000\u0000\u0000\u0000\u0000\u0000\u0000\u0000\u0000\u0000M\u0000\u000f\u0000\u0006\u0000\u0003\u0000\u0001PZR.AI          PZR.BV          PZR.CI          PZR.AV          PZR.BI          PZR.CV          ANA1            ANA2            ANA3            DIG.stat1_01    DIG.stat1_02    DIG.stat1_03    DIG.stat1_04    DIG.stat1_05    DIG.stat1_06    DIG.stat1_07    DIG.stat1_08    DIG.stat1_09    DIG.stat1_10    DIG.stat1_11    DIG.stat1_12    DIG.stat1_13    DIG.stat1_14    DIG.stat1_15    DIG.stat1_16    \u0001\u0000\u0000\u0000\u0000\u0000\u0000\u0000\u0001\u0000\u0000\u0000\u0000\u0000\u0000\u0000\u0001\u0000\u0000\u0000\u0000\u0000\u0000\u0000\u0000\u0000\u0000\u0000\u0000\u0000\u0000\u0000\u0000\u0000\u0000\u0000ÿÿ\u0000\u0000\u0000\u0000\u0000\u0000", "PMU.078\u0000\u0000\u0000\u0000\u0000\u0000\u0000\u0000\u0000\u0000N\u0000\u000f\u0000\u0006\u0000\u0003\u0000\u0001PZR.AI          PZR.BV          PZR.CI          PZR.AV          PZR.BI          PZR.CV          ANA1            ANA2            ANA3            DIG.stat1_01    DIG.stat1_02    DIG.stat1_03    DIG.stat1_04    DIG.stat1_05    DIG.stat1_06    DIG.stat1_07    DIG.stat1_08    DIG.stat1_09    DIG.stat1_10    DIG.stat1_11    DIG.stat1_12    DIG.stat1_13    DIG.stat1_14    DIG.stat1_15    DIG.stat1_16    \u0001\u0000\u0000\u0000\u0000\u0000\u0000\u0000\u0001\u0000\u0000\u0000\u0000\u0000\u0000\u0000\u0001\u0000\u0000\u0000\u0000\u0000\u0000\u0000\u0000\u0000\u0000\u0000\u0000\u0000\u0000\u0000\u0000\u0000\u0000\u0000ÿÿ\u0000\u0000\u0000\u0000\u0000\u0000", "PMU.079\u0000\u0000\u0000\u0000\u0000\u0000\u0000\u0000\u0000\u0000O\u0000\u000f\u0000\u0006\u0000\u0003\u0000\u0001PZR.AI          PZR.BV          PZR.CI          PZR.AV          PZR.BI          PZR.CV          ANA1            ANA2            ANA3            DIG.stat1_01    DIG.stat1_02    DIG.stat1_03    DIG.stat1_04    DIG.stat1_05    DIG.stat1_06    DIG.stat1_07    DIG.stat1_08    DIG.stat1_09    DIG.stat1_10    DIG.stat1_11    DIG.stat1_12    DIG.stat1_13    DIG.stat1_14    DIG.stat1_15    DIG.stat1_16    \u0001\u0000\u0000\u0000\u0000\u0000\u0000\u0000\u0001\u0000\u0000\u0000\u0000\u0000\u0000\u0000\u0001\u0000\u0000\u0000\u0000\u0000\u0000\u0000\u0000\u0000\u0000\u0000\u0000\u0000\u0000\u0000\u0000\u0000\u0000\u0000ÿÿ\u0000\u0000\u0000\u0000\u0000\u0000", "PMU.080\u0000\u0000\u0000\u0000\u0000\u0000\u0000\u0000\u0000\u0000P\u0000\u000f\u0000\u0006\u0000\u0003\u0000\u0001PZR.AI          PZR.BV          PZR.CI          PZR.AV          PZR.BI          PZR.CV          ANA1            ANA2            ANA3            DIG.stat1_01    DIG.stat1_02    DIG.stat1_03    DIG.stat1_04    DIG.stat1_05    DIG.stat1_06    DIG.stat1_07    DIG.stat1_08    DIG.stat1_09    DIG.stat1_10    DIG.stat1_11    DIG.stat1_12    DIG.stat1_13    DIG.stat1_14    DIG.stat1_15    DIG.stat1_16    \u0001\u0000\u0000\u0000\u0000\u0000\u0000\u0000\u0001\u0000\u0000\u0000\u0000\u0000\u0000\u0000\u0001\u0000\u0000\u0000\u0000\u0000\u0000\u0000\u0000\u0000\u0000\u0000\u0000\u0000\u0000\u0000\u0000\u0000\u0000\u0000ÿÿ\u0000\u0000\u0000\u0000\u0000\u0000", "PMU.081\u0000\u0000\u0000\u0000\u0000\u0000\u0000\u0000\u0000\u0000Q\u0000\u000f\u0000\u0006\u0000\u0003\u0000\u0001PZR.AI          PZR.BV          PZR.CI          PZR.AV          PZR.BI          PZR.CV          ANA1            ANA2            ANA3            DIG.stat1_01    DIG.stat1_02    DIG.stat1_03    DIG.stat1_04    DIG.stat1_05    DIG.stat1_06    DIG.stat1_07    DIG.stat1_08    DIG.stat1_09    DIG.stat1_10    DIG.stat1_11    DIG.stat1_12    DIG.stat1_13    DIG.stat1_14    DIG.stat1_15    DIG.stat1_16    \u0001\u0000\u0000\u0000\u0000\u0000\u0000\u0000\u0001\u0000\u0000\u0000\u0000\u0000\u0000\u0000\u0001\u0000\u0000\u0000\u0000\u0000\u0000\u0000\u0000\u0000\u0000\u0000\u0000\u0000\u0000\u0000\u0000\u0000\u0000\u0000ÿÿ\u0000\u0000\u0000\u0000\u0000\u0000", "PMU.082\u0000\u0000\u0000\u0000\u0000\u0000\u0000\u0000\u0000\u0000R\u0000\u000f\u0000\u0006\u0000\u0003\u0000\u0001PZR.AI          PZR.BV          PZR.CI          PZR.AV          PZR.BI          PZR.CV          ANA1            ANA2            ANA3            DIG.stat1_01    DIG.stat1_02    DIG.stat1_03    DIG.stat1_04    DIG.stat1_05    DIG.stat1_06    DIG.stat1_07    DIG.stat1_08    DIG.stat1_09    DIG.stat1_10    DIG.stat1_11    DIG.stat1_12    DIG.stat1_13    DIG.stat1_14    DIG.stat1_15    DIG.stat1_16    \u0001\u0000\u0000\u0000\u0000\u0000\u0000\u0000\u0001\u0000\u0000\u0000\u0000\u0000\u0000\u0000\u0001\u0000\u0000\u0000\u0000\u0000\u0000\u0000\u0000\u0000\u0000\u0000\u0000\u0000\u0000\u0000\u0000\u0000\u0000\u0000ÿÿ\u0000\u0000\u0000\u0000\u0000\u0000", "PMU.083\u0000\u0000\u0000\u0000\u0000\u0000\u0000\u0000\u0000\u0000S\u0000\u000f\u0000\u0006\u0000\u0003\u0000\u0001PZR.AI          PZR.BV          PZR.CI          PZR.AV          PZR.BI          PZR.CV          ANA1            ANA2            ANA3            DIG.stat1_01    DIG.stat1_02    DIG.stat1_03    DIG.stat1_04    DIG.stat1_05    DIG.stat1_06    DIG.stat1_07    DIG.stat1_08    DIG.stat1_09    DIG.stat1_10    DIG.stat1_11    DIG.stat1_12    DIG.stat1_13    DIG.stat1_14    DIG.stat1_15    DIG.stat1_16    \u0001\u0000\u0000\u0000\u0000\u0000\u0000\u0000\u0001\u0000\u0000\u0000\u0000\u0000\u0000\u0000\u0001\u0000\u0000\u0000\u0000\u0000\u0000\u0000\u0000\u0000\u0000\u0000\u0000\u0000\u0000\u0000\u0000\u0000\u0000\u0000ÿÿ\u0000\u0000\u0000\u0000\u0000\u0000", "PMU.084\u0000\u0000\u0000\u0000\u0000\u0000\u0000\u0000\u0000\u0000T\u0000\u000f\u0000\u0006\u0000\u0003\u0000\u0001PZR.AI          PZR.BV          PZR.CI          PZR.AV          PZR.BI          PZR.CV          ANA1            ANA2            ANA3            DIG.stat1_01    DIG.stat1_02    DIG.stat1_03    DIG.stat1_04    DIG.stat1_05    DIG.stat1_06    DIG.stat1_07    DIG.stat1_08    DIG.stat1_09    DIG.stat1_10    DIG.stat1_11    DIG.stat1_12    DIG.stat1_13    DIG.stat1_14    DIG.stat1_15    DIG.stat1_16    \u0001\u0000\u0000\u0000\u0000\u0000\u0000\u0000\u0001\u0000\u0000\u0000\u0000\u0000\u0000\u0000\u0001\u0000\u0000\u0000\u0000\u0000\u0000\u0000\u0000\u0000\u0000\u0000\u0000\u0000\u0000\u0000\u0000\u0000\u0000\u0000ÿÿ\u0000\u0000\u0000\u0000\u0000\u0000", "PMU.085\u0000\u0000\u0000\u0000\u0000\u0000\u0000\u0000\u0000\u0000U\u0000\u000f\u0000\u0006\u0000\u0003\u0000\u0001PZR.AI          PZR.BV          PZR.CI          PZR.AV          PZR.BI          PZR.CV          ANA1            ANA2            ANA3            DIG.stat1_01    DIG.stat1_02    DIG.stat1_03    DIG.stat1_04    DIG.stat1_05    DIG.stat1_06    DIG.stat1_07    DIG.stat1_08    DIG.stat1_09    DIG.stat1_10    DIG.stat1_11    DIG.stat1_12    DIG.stat1_13    DIG.stat1_14    DIG.stat1_15    DIG.stat1_16    \u0001\u0000\u0000\u0000\u0000\u0000\u0000\u0000\u0001\u0000\u0000\u0000\u0000\u0000\u0000\u0000\u0001\u0000\u0000\u0000\u0000\u0000\u0000\u0000\u0000\u0000\u0000\u0000\u0000\u0000\u0000\u0000\u0000\u0000\u0000\u0000ÿÿ\u0000\u0000\u0000\u0000\u0000\u0000", "PMU.086\u0000\u0000\u0000\u0000\u0000\u0000\u0000\u0000\u0000\u0000V\u0000\u000f\u0000\u0006\u0000\u0003\u0000\u0001PZR.AI          PZR.BV          PZR.CI          PZR.AV          PZR.BI          PZR.CV          ANA1            ANA2            ANA3            DIG.stat1_01    DIG.stat1_02    DIG.stat1_03    DIG.stat1_04    DIG.stat1_05    DIG.stat1_06    DIG.stat1_07    DIG.stat1_08    DIG.stat1_09    DIG.stat1_10    DIG.stat1_11    DIG.stat1_12    DIG.stat1_13    DIG.stat1_14    DIG.stat1_15    DIG.stat1_16    \u0001\u0000\u0000\u0000\u0000\u0000\u0000\u0000\u0001\u0000\u0000\u0000\u0000\u0000\u0000\u0000\u0001\u0000\u0000\u0000\u0000\u0000\u0000\u0000\u0000\u0000\u0000\u0000\u0000\u0000\u0000\u0000\u0000\u0000\u0000\u0000ÿÿ\u0000\u0000\u0000\u0000\u0000\u0000", "PMU.087\u0000\u0000\u0000\u0000\u0000\u0000\u0000\u0000\u0000\u0000W\u0000\u000f\u0000\u0006\u0000\u0003\u0000\u0001PZR.AI          PZR.BV          PZR.CI          PZR.AV          PZR.BI          PZR.CV          ANA1            ANA2            ANA3            DIG.stat1_01    DIG.stat1_02    DIG.stat1_03    DIG.stat1_04    DIG.stat1_05    DIG.stat1_06    DIG.stat1_07    DIG.stat1_08    DIG.stat1_09    DIG.stat1_10    DIG.stat1_11    DIG.stat1_12    DIG.stat1_13    DIG.stat1_14    DIG.stat1_15    DIG.stat1_16    \u0001\u0000\u0000\u0000\u0000\u0000\u0000\u0000\u0001\u0000\u0000\u0000\u0000\u0000\u0000\u0000\u0001\u0000\u0000\u0000\u0000\u0000\u0000\u0000\u0000\u0000\u0000\u0000\u0000\u0000\u0000\u0000\u0000\u0000\u0000\u0000ÿÿ\u0000\u0000\u0000\u0000\u0000\u0000", "PMU.088\u0000\u0000\u0000\u0000\u0000\u0000\u0000\u0000\u0000\u0000X\u0000\u000f\u0000\u0006\u0000\u0003\u0000\u0001PZR.AI          PZR.BV          PZR.CI          PZR.AV          PZR.BI          PZR.CV          ANA1            ANA2            ANA3            DIG.stat1_01    DIG.stat1_02    DIG.stat1_03    DIG.stat1_04    DIG.stat1_05    DIG.stat1_06    DIG.stat1_07    DIG.stat1_08    DIG.stat1_09    DIG.stat1_10    DIG.stat1_11    DIG.stat1_12    DIG.stat1_13    DIG.stat1_14    DIG.stat1_15    DIG.stat1_16    \u0001\u0000\u0000\u0000\u0000\u0000\u0000\u0000\u0001\u0000\u0000\u0000\u0000\u0000\u0000\u0000\u0001\u0000\u0000\u0000\u0000\u0000\u0000\u0000\u0000\u0000\u0000\u0000\u0000\u0000\u0000\u0000\u0000\u0000\u0000\u0000ÿÿ\u0000\u0000\u0000\u0000\u0000\u0000", "PMU.089\u0000\u0000\u0000\u0000\u0000\u0000\u0000\u0000\u0000\u0000Y\u0000\u000f\u0000\u0006\u0000\u0003\u0000\u0001PZR.AI          PZR.BV          PZR.CI          PZR.AV          PZR.BI          PZR.CV          ANA1            ANA2            ANA3            DIG.stat1_01    DIG.stat1_02    DIG.stat1_03    DIG.stat1_04    DIG.stat1_05    DIG.stat1_06    DIG.stat1_07    DIG.stat1_08    DIG.stat1_09    DIG.stat1_10    DIG.stat1_11    DIG.stat1_12    DIG.stat1_13    DIG.stat1_14    DIG.stat1_15    DIG.stat1_16    \u0001\u0000\u0000\u0000\u0000\u0000\u0000\u0000\u0001\u0000\u0000\u0000\u0000\u0000\u0000\u0000\u0001\u0000\u0000\u0000\u0000\u0000\u0000\u0000\u0000\u0000\u0000\u0000\u0000\u0000\u0000\u0000\u0000\u0000\u0000\u0000ÿÿ\u0000\u0000\u0000\u0000\u0000\u0000", "PMU.090\u0000\u0000\u0000\u0000\u0000\u0000\u0000\u0000\u0000\u0000Z\u0000\u000f\u0000\u0006\u0000\u0003\u0000\u0001PZR.AI          PZR.BV          PZR.CI          PZR.AV          PZR.BI          PZR.CV          ANA1            ANA2            ANA3            DIG.stat1_01    DIG.stat1_02    DIG.stat1_03    DIG.stat1_04    DIG.stat1_05    DIG.stat1_06    DIG.stat1_07    DIG.stat1_08    DIG.stat1_09    DIG.stat1_10    DIG.stat1_11    DIG.stat1_12    DIG.stat1_13    DIG.stat1_14    DIG.stat1_15    DIG.stat1_16    \u0001\u0000\u0000\u0000\u0000\u0000\u0000\u0000\u0001\u0000\u0000\u0000\u0000\u0000\u0000\u0000\u0001\u0000\u0000\u0000\u0000\u0000\u0000\u0000\u0000\u0000\u0000\u0000\u0000\u0000\u0000\u0000\u0000\u0000\u0000\u0000ÿÿ\u0000\u0000\u0000\u0000\u0000\u0000", "PMU.091\u0000\u0000\u0000\u0000\u0000\u0000\u0000\u0000\u0000\u0000[\u0000\u000f\u0000\u0006\u0000\u0003\u0000\u0001PZR.AI          PZR.BV          PZR.CI          PZR.AV          PZR.BI          PZR.CV          ANA1            ANA2            ANA3            DIG.stat1_01    DIG.stat1_02    DIG.stat1_03    DIG.stat1_04    DIG.stat1_05    DIG.stat1_06    DIG.stat1_07    DIG.stat1_08    DIG.stat1_09    DIG.stat1_10    DIG.stat1_11    DIG.stat1_12    DIG.stat1_13    DIG.stat1_14    DIG.stat1_15    DIG.stat1_16    \u0001\u0000\u0000\u0000\u0000\u0000\u0000\u0000\u0001\u0000\u0000\u0000\u0000\u0000\u0000\u0000\u0001\u0000\u0000\u0000\u0000\u0000\u0000\u0000\u0000\u0000\u0000\u0000\u0000\u0000\u0000\u0000\u0000\u0000\u0000\u0000ÿÿ\u0000\u0000\u0000\u0000\u0000\u0000", "PMU.092\u0000\u0000\u0000\u0000\u0000\u0000\u0000\u0000\u0000\u0000\\\u0000\u000f\u0000\u0006\u0000\u0003\u0000\u0001PZR.AI          PZR.BV          PZR.CI          PZR.AV          PZR.BI          PZR.CV          ANA1            ANA2            ANA3            DIG.stat1_01    DIG.stat1_02    DIG.stat1_03    DIG.stat1_04    DIG.stat1_05    DIG.stat1_06    DIG.stat1_07    DIG.stat1_08    DIG.stat1_09    DIG.stat1_10    DIG.stat1_11    DIG.stat1_12    DIG.stat1_13    DIG.stat1_14    DIG.stat1_15    DIG.stat1_16    \u0001\u0000\u0000\u0000\u0000\u0000\u0000\u0000\u0001\u0000\u0000\u0000\u0000\u0000\u0000\u0000\u0001\u0000\u0000\u0000\u0000\u0000\u0000\u0000\u0000\u0000\u0000\u0000\u0000\u0000\u0000\u0000\u0000\u0000\u0000\u0000ÿÿ\u0000\u0000\u0000\u0000\u0000\u0000", "PMU.093\u0000\u0000\u0000\u0000\u0000\u0000\u0000\u0000\u0000\u0000]\u0000\u000f\u0000\u0006\u0000\u0003\u0000\u0001PZR.AI          PZR.BV          PZR.CI          PZR.AV          PZR.BI          PZR.CV          ANA1            ANA2            ANA3            DIG.stat1_01    DIG.stat1_02    DIG.stat1_03    DIG.stat1_04    DIG.stat1_05    DIG.stat1_06    DIG.stat1_07    DIG.stat1_08    DIG.stat1_09    DIG.stat1_10    DIG.stat1_11    DIG.stat1_12    DIG.stat1_13    DIG.stat1_14    DIG.stat1_15    DIG.stat1_16    \u0001\u0000\u0000\u0000\u0000\u0000\u0000\u0000\u0001\u0000\u0000\u0000\u0000\u0000\u0000\u0000\u0001\u0000\u0000\u0000\u0000\u0000\u0000\u0000\u0000\u0000\u0000\u0000\u0000\u0000\u0000\u0000\u0000\u0000\u0000\u0000ÿÿ\u0000\u0000\u0000\u0000\u0000\u0000", "PMU.094\u0000\u0000\u0000\u0000\u0000\u0000\u0000\u0000\u0000\u0000^\u0000\u000f\u0000\u0006\u0000\u0003\u0000\u0001PZR.AI          PZR.BV          PZR.CI          PZR.AV          PZR.BI          PZR.CV          ANA1            ANA2            ANA3            DIG.stat1_01    DIG.stat1_02    DIG.stat1_03    DIG.stat1_04    DIG.stat1_05    DIG.stat1_06    DIG.stat1_07    DIG.stat1_08    DIG.stat1_09    DIG.stat1_10    DIG.stat1_11    DIG.stat1_12    DIG.stat1_13    DIG.stat1_14    DIG.stat1_15    DIG.stat1_16    \u0001\u0000\u0000\u0000\u0000\u0000\u0000\u0000\u0001\u0000\u0000\u0000\u0000\u0000\u0000\u0000\u0001\u0000\u0000\u0000\u0000\u0000\u0000\u0000\u0000\u0000\u0000\u0000\u0000\u0000\u0000\u0000\u0000\u0000\u0000\u0000ÿÿ\u0000\u0000\u0000\u0000\u0000\u0000", "PMU.095\u0000\u0000\u0000\u0000\u0000\u0000\u0000\u0000\u0000\u0000_\u0000\u000f\u0000\u0006\u0000\u0003\u0000\u0001PZR.AI          PZR.BV          PZR.CI          PZR.AV          PZR.BI          PZR.CV          ANA1            ANA2            ANA3            DIG.stat1_01    DIG.stat1_02    DIG.stat1_03    DIG.stat1_04    DIG.stat1_05    DIG.stat1_06    DIG.stat1_07    DIG.stat1_08    DIG.stat1_09    DIG.stat1_10    DIG.stat1_11    DIG.stat1_12    DIG.stat1_13    DIG.stat1_14    DIG.stat1_15    DIG.stat1_16    \u0001\u0000\u0000\u0000\u0000\u0000\u0000\u0000\u0001\u0000\u0000\u0000\u0000\u0000\u0000\u0000\u0001\u0000\u0000\u0000\u0000\u0000\u0000\u0000\u0000\u0000\u0000\u0000\u0000\u0000\u0000\u0000\u0000\u0000\u0000\u0000ÿÿ\u0000\u0000\u0000\u0000\u0000\u0000", "PMU.096\u0000\u0000\u0000\u0000\u0000\u0000\u0000\u0000\u0000\u0000`\u0000\u000f\u0000\u0006\u0000\u0003\u0000\u0001PZR.AI          PZR.BV          PZR.CI          PZR.AV          PZR.BI          PZR.CV          ANA1            ANA2            ANA3            DIG.stat1_01    DIG.stat1_02    DIG.stat1_03    DIG.stat1_04    DIG.stat1_05    DIG.stat1_06    DIG.stat1_07    DIG.stat1_08    DIG.stat1_09    DIG.stat1_10    DIG.stat1_11    DIG.stat1_12    DIG.stat1_13    DIG.stat1_14    DIG.stat1_15    DIG.stat1_16    \u0001\u0000\u0000\u0000\u0000\u0000\u0000\u0000\u0001\u0000\u0000\u0000\u0000\u0000\u0000\u0000\u0001\u0000\u0000\u0000\u0000\u0000\u0000\u0000\u0000\u0000\u0000\u0000\u0000\u0000\u0000\u0000\u0000\u0000\u0000\u0000ÿÿ\u0000\u0000\u0000\u0000\u0000\u0000", "PMU.097\u0000\u0000\u0000\u0000\u0000\u0000\u0000\u0000\u0000\u0000a\u0000\u000f\u0000\u0006\u0000\u0003\u0000\u0001PZR.AI          PZR.BV          PZR.CI          PZR.AV          PZR.BI          PZR.CV          ANA1            ANA2            ANA3            DIG.stat1_01    DIG.stat1_02    DIG.stat1_03    DIG.stat1_04    DIG.stat1_05    DIG.stat1_06    DIG.stat1_07    DIG.stat1_08    DIG.stat1_09    DIG.stat1_10    DIG.stat1_11    DIG.stat1_12    DIG.stat1_13    DIG.stat1_14    DIG.stat1_15    DIG.stat1_16    \u0001\u0000\u0000\u0000\u0000\u0000\u0000\u0000\u0001\u0000\u0000\u0000\u0000\u0000\u0000\u0000\u0001\u0000\u0000\u0000\u0000\u0000\u0000\u0000\u0000\u0000\u0000\u0000\u0000\u0000\u0000\u0000\u0000\u0000\u0000\u0000ÿÿ\u0000\u0000\u0000\u0000\u0000\u0000", "PMU.098\u0000\u0000\u0000\u0000\u0000\u0000\u0000\u0000\u0000\u0000b\u0000\u000f\u0000\u0006\u0000\u0003\u0000\u0001PZR.AI          PZR.BV          PZR.CI          PZR.AV          PZR.BI          PZR.CV          ANA1            ANA2            ANA3            DIG.stat1_01    DIG.stat1_02    DIG.stat1_03    DIG.stat1_04    DIG.stat1_05    DIG.stat1_06    DIG.stat1_07    DIG.stat1_08    DIG.stat1_09    DIG.stat1_10    DIG.stat1_11    DIG.stat1_12    DIG.stat1_13    DIG.stat1_14    DIG.stat1_15    DIG.stat1_16    \u0001\u0000\u0000\u0000\u0000\u0000\u0000\u0000\u0001\u0000\u0000\u0000\u0000\u0000\u0000\u0000\u0001\u0000\u0000\u0000\u0000\u0000\u0000\u0000\u0000\u0000\u0000\u0000\u0000\u0000\u0000\u0000\u0000\u0000\u0000\u0000ÿÿ\u0000\u0000\u0000\u0000\u0000\u0000", "PMU.099\u0000\u0000\u0000\u0000\u0000\u0000\u0000\u0000\u0000\u0000c\u0000\u000f\u0000\u0006\u0000\u0003\u0000\u0001PZR.AI          PZR.BV          PZR.CI          PZR.AV          PZR.BI          PZR.CV          ANA1            ANA2            ANA3            DIG.stat1_01    DIG.stat1_02    DIG.stat1_03    DIG.stat1_04    DIG.stat1_05    DIG.stat1_06    DIG.stat1_07    DIG.stat1_08    DIG.stat1_09    DIG.stat1_10    DIG.stat1_11    DIG.stat1_12    DIG.stat1_13    DIG.stat1_14    DIG.stat1_15    DIG.stat1_16    \u0001\u0000\u0000\u0000\u0000\u0000\u0000\u0000\u0001\u0000\u0000\u0000\u0000\u0000\u0000\u0000\u0001\u0000\u0000\u0000\u0000\u0000\u0000\u0000\u0000\u0000\u0000\u0000\u0000\u0000\u0000\u0000\u0000\u0000\u0000\u0000ÿÿ\u0000\u0000\u0000\u0000\u0000\u0000", "PMU.100\u0000\u0000\u0000\u0000\u0000\u0000\u0000\u0000\u0000\u0000d\u0000\u000f\u0000\u0006\u0000\u0003\u0000\u0001PZR.AI          PZR.BV          PZR.CI          PZR.AV          PZR.BI          PZR.CV          ANA1            ANA2            ANA3            DIG.stat1_01    DIG.stat1_02    DIG.stat1_03    DIG.stat1_04    DIG.stat1_05    DIG.stat1_06    DIG.stat1_07    DIG.stat1_08    DIG.stat1_09    DIG.stat1_10    DIG.stat1_11    DIG.stat1_12    DIG.stat1_13    DIG.stat1_14    DIG.stat1_15    DIG.stat1_16    \u0001\u0000\u0000\u0000\u0000\u0000\u0000\u0000\u0001\u0000\u0000\u0000\u0000\u0000\u0000\u0000\u0001\u0000\u0000\u0000\u0000\u0000\u0000\u0000\u0000\u0000\u0000\u0000\u0000\u0000\u0000\u0000\u0000\u0000\u0000\u0000ÿÿ\u0000\u0000\u0000\u0000\u0000\u0000", "PMU.101\u0000\u0000\u0000\u0000\u0000\u0000\u0000\u0000\u0000\u0000e\u0000\u000f\u0000\u0006\u0000\u0003\u0000\u0001PZR.AI          PZR.BV          PZR.CI          PZR.AV          PZR.BI          PZR.CV          ANA1            ANA2            ANA3            DIG.stat1_01    DIG.stat1_02    DIG.stat1_03    DIG.stat1_04    DIG.stat1_05    DIG.stat1_06    DIG.stat1_07    DIG.stat1_08    DIG.stat1_09    DIG.stat1_10    DIG.stat1_11    DIG.stat1_12    DIG.stat1_13    DIG.stat1_14    DIG.stat1_15    DIG.stat1_16    \u0001\u0000\u0000\u0000\u0000\u0000\u0000\u0000\u0001\u0000\u0000\u0000\u0000\u0000\u0000\u0000\u0001\u0000\u0000\u0000\u0000\u0000\u0000\u0000\u0000\u0000\u0000\u0000\u0000\u0000\u0000\u0000\u0000\u0000\u0000\u0000ÿÿ\u0000\u0000\u0000\u0000\u0000\u0000", "PMU.102\u0000\u0000\u0000\u0000\u0000\u0000\u0000\u0000\u0000\u0000f\u0000\u000f\u0000\u0006\u0000\u0003\u0000\u0001PZR.AI          PZR.BV          PZR.CI          PZR.AV          PZR.BI          PZR.CV          ANA1            ANA2            ANA3            DIG.stat1_01    DIG.stat1_02    DIG.stat1_03    DIG.stat1_04    DIG.stat1_05    DIG.stat1_06    DIG.stat1_07    DIG.stat1_08    DIG.stat1_09    DIG.stat1_10    DIG.stat1_11    DIG.stat1_12    DIG.stat1_13    DIG.stat1_14    DIG.stat1_15    DIG.stat1_16    \u0001\u0000\u0000\u0000\u0000\u0000\u0000\u0000\u0001\u0000\u0000\u0000\u0000\u0000\u0000\u0000\u0001\u0000\u0000\u0000\u0000\u0000\u0000\u0000\u0000\u0000\u0000\u0000\u0000\u0000\u0000\u0000\u0000\u0000\u0000\u0000ÿÿ\u0000\u0000\u0000\u0000\u0000\u0000", "PMU.103\u0000\u0000\u0000\u0000\u0000\u0000\u0000\u0000\u0000\u0000g\u0000\u000f\u0000\u0006\u0000\u0003\u0000\u0001PZR.AI          PZR.BV          PZR.CI          PZR.AV          PZR.BI          PZR.CV          ANA1            ANA2            ANA3            DIG.stat1_01    DIG.stat1_02    DIG.stat1_03    DIG.stat1_04    DIG.stat1_05    DIG.stat1_06    DIG.stat1_07    DIG.stat1_08    DIG.stat1_09    DIG.stat1_10    DIG.stat1_11    DIG.stat1_12    DIG.stat1_13    DIG.stat1_14    DIG.stat1_15    DIG.stat1_16    \u0001\u0000\u0000\u0000\u0000\u0000\u0000\u0000\u0001\u0000\u0000\u0000\u0000\u0000\u0000\u0000\u0001\u0000\u0000\u0000\u0000\u0000\u0000\u0000\u0000\u0000\u0000\u0000\u0000\u0000\u0000\u0000\u0000\u0000\u0000\u0000ÿÿ\u0000\u0000\u0000\u0000\u0000\u0000", "PMU.104\u0000\u0000\u0000\u0000\u0000\u0000\u0000\u0000\u0000\u0000h\u0000\u000f\u0000\u0006\u0000\u0003\u0000\u0001PZR.AI          PZR.BV          PZR.CI          PZR.AV          PZR.BI          PZR.CV          ANA1            ANA2            ANA3            DIG.stat1_01    DIG.stat1_02    DIG.stat1_03    DIG.stat1_04    DIG.stat1_05    DIG.stat1_06    DIG.stat1_07    DIG.stat1_08    DIG.stat1_09    DIG.stat1_10    DIG.stat1_11    DIG.stat1_12    DIG.stat1_13    DIG.stat1_14    DIG.stat1_15    DIG.stat1_16    \u0001\u0000\u0000\u0000\u0000\u0000\u0000\u0000\u0001\u0000\u0000\u0000\u0000\u0000\u0000\u0000\u0001\u0000\u0000\u0000\u0000\u0000\u0000\u0000\u0000\u0000\u0000\u0000\u0000\u0000\u0000\u0000\u0000\u0000\u0000\u0000ÿÿ\u0000\u0000\u0000\u0000\u0000\u0000", "PMU.105\u0000\u0000\u0000\u0000\u0000\u0000\u0000\u0000\u0000\u0000i\u0000\u000f\u0000\u0006\u0000\u0003\u0000\u0001PZR.AI          PZR.BV          PZR.CI          PZR.AV          PZR.BI          PZR.CV          ANA1            ANA2            ANA3            DIG.stat1_01    DIG.stat1_02    DIG.stat1_03    DIG.stat1_04    DIG.stat1_05    DIG.stat1_06    DIG.stat1_07    DIG.stat1_08    DIG.stat1_09    DIG.stat1_10    DIG.stat1_11    DIG.stat1_12    DIG.stat1_13    DIG.stat1_14    DIG.stat1_15    DIG.stat1_16    \u0001\u0000\u0000\u0000\u0000\u0000\u0000\u0000\u0001\u0000\u0000\u0000\u0000\u0000\u0000\u0000\u0001\u0000\u0000\u0000\u0000\u0000\u0000\u0000\u0000\u0000\u0000\u0000\u0000\u0000\u0000\u0000\u0000\u0000\u0000\u0000ÿÿ\u0000\u0000\u0000\u0000\u0000\u0000", "PMU.106\u0000\u0000\u0000\u0000\u0000\u0000\u0000\u0000\u0000\u0000j\u0000\u000f\u0000\u0006\u0000\u0003\u0000\u0001PZR.AI          PZR.BV          PZR.CI          PZR.AV          PZR.BI          PZR.CV          ANA1            ANA2            ANA3            DIG.stat1_01    DIG.stat1_02    DIG.stat1_03    DIG.stat1_04    DIG.stat1_05    DIG.stat1_06    DIG.stat1_07    DIG.stat1_08    DIG.stat1_09    DIG.stat1_10    DIG.stat1_11    DIG.stat1_12    DIG.stat1_13    DIG.stat1_14    DIG.stat1_15    DIG.stat1_16    \u0001\u0000\u0000\u0000\u0000\u0000\u0000\u0000\u0001\u0000\u0000\u0000\u0000\u0000\u0000\u0000\u0001\u0000\u0000\u0000\u0000\u0000\u0000\u0000\u0000\u0000\u0000\u0000\u0000\u0000\u0000\u0000\u0000\u0000\u0000\u0000ÿÿ\u0000\u0000\u0000\u0000\u0000\u0000", "PMU.107\u0000\u0000\u0000\u0000\u0000\u0000\u0000\u0000\u0000\u0000k\u0000\u000f\u0000\u0006\u0000\u0003\u0000\u0001PZR.AI          PZR.BV          PZR.CI          PZR.AV          PZR.BI          PZR.CV          ANA1            ANA2            ANA3            DIG.stat1_01    DIG.stat1_02    DIG.stat1_03    DIG.stat1_04    DIG.stat1_05    DIG.stat1_06    DIG.stat1_07    DIG.stat1_08    DIG.stat1_09    DIG.stat1_10    DIG.stat1_11    DIG.stat1_12    DIG.stat1_13    DIG.stat1_14    DIG.stat1_15    DIG.stat1_16    \u0001\u0000\u0000\u0000\u0000\u0000\u0000\u0000\u0001\u0000\u0000\u0000\u0000\u0000\u0000\u0000\u0001\u0000\u0000\u0000\u0000\u0000\u0000\u0000\u0000\u0000\u0000\u0000\u0000\u0000\u0000\u0000\u0000\u0000\u0000\u0000ÿÿ\u0000\u0000\u0000\u0000\u0000\u0000", "PMU.108\u0000\u0000\u0000\u0000\u0000\u0000\u0000\u0000\u0000\u0000l\u0000\u000f\u0000\u0006\u0000\u0003\u0000\u0001PZR.AI          PZR.BV          PZR.CI          PZR.AV          PZR.BI          PZR.CV          ANA1            ANA2            ANA3            DIG.stat1_01    DIG.stat1_02    DIG.stat1_03    DIG.stat1_04    DIG.stat1_05    DIG.stat1_06    DIG.stat1_07    DIG.stat1_08    DIG.stat1_09    DIG.stat1_10    DIG.stat1_11    DIG.stat1_12    DIG.stat1_13    DIG.stat1_14    DIG.stat1_15    DIG.stat1_16    \u0001\u0000\u0000\u0000\u0000\u0000\u0000\u0000\u0001\u0000\u0000\u0000\u0000\u0000\u0000\u0000\u0001\u0000\u0000\u0000\u0000\u0000\u0000\u0000\u0000\u0000\u0000\u0000\u0000\u0000\u0000\u0000\u0000\u0000\u0000\u0000ÿÿ\u0000\u0000\u0000\u0000\u0000\u0000", "PMU.109\u0000\u0000\u0000\u0000\u0000\u0000\u0000\u0000\u0000\u0000m\u0000\u000f\u0000\u0006\u0000\u0003\u0000\u0001PZR.AI          PZR.BV          PZR.CI          PZR.AV          PZR.BI          PZR.CV          ANA1            ANA2            ANA3            DIG.stat1_01    DIG.stat1_02    DIG.stat1_03    DIG.stat1_04    DIG.stat1_05    DIG.stat1_06    DIG.stat1_07    DIG.stat1_08    DIG.stat1_09    DIG.stat1_10    DIG.stat1_11    DIG.stat1_12    DIG.stat1_13    DIG.stat1_14    DIG.stat1_15    DIG.stat1_16    \u0001\u0000\u0000\u0000\u0000\u0000\u0000\u0000\u0001\u0000\u0000\u0000\u0000\u0000\u0000\u0000\u0001\u0000\u0000\u0000\u0000\u0000\u0000\u0000\u0000\u0000\u0000\u0000\u0000\u0000\u0000\u0000\u0000\u0000\u0000\u0000ÿÿ\u0000\u0000\u0000\u0000\u0000\u0000", "PMU.110\u0000\u0000\u0000\u0000\u0000\u0000\u0000\u0000\u0000\u0000n\u0000\u000f\u0000\u0006\u0000\u0003\u0000\u0001PZR.AI          PZR.BV          PZR.CI          PZR.AV          PZR.BI          PZR.CV          ANA1            ANA2            ANA3            DIG.stat1_01    DIG.stat1_02    DIG.stat1_03    DIG.stat1_04    DIG.stat1_05    DIG.stat1_06    DIG.stat1_07    DIG.stat1_08    DIG.stat1_09    DIG.stat1_10    DIG.stat1_11    DIG.stat1_12    DIG.stat1_13    DIG.stat1_14    DIG.stat1_15    DIG.stat1_16    \u0001\u0000\u0000\u0000\u0000\u0000\u0000\u0000\u0001\u0000\u0000\u0000\u0000\u0000\u0000\u0000\u0001\u0000\u0000\u0000\u0000\u0000\u0000\u0000\u0000\u0000\u0000\u0000\u0000\u0000\u0000\u0000\u0000\u0000\u0000\u0000ÿÿ\u0000\u0000\u0000\u0000\u0000\u0000", "PMU.111\u0000\u0000\u0000\u0000\u0000\u0000\u0000\u0000\u0000\u0000o\u0000\u000f\u0000\u0006\u0000\u0003\u0000\u0001PZR.AI          PZR.BV          PZR.CI          PZR.AV          PZR.BI          PZR.CV          ANA1            ANA2            ANA3            DIG.stat1_01    DIG.stat1_02    DIG.stat1_03    DIG.stat1_04    DIG.stat1_05    DIG.stat1_06    DIG.stat1_07    DIG.stat1_08    DIG.stat1_09    DIG.stat1_10    DIG.stat1_11    DIG.stat1_12    DIG.stat1_13    DIG.stat1_14    DIG.stat1_15    DIG.stat1_16    \u0001\u0000\u0000\u0000\u0000\u0000\u0000\u0000\u0001\u0000\u0000\u0000\u0000\u0000\u0000\u0000\u0001\u0000\u0000\u0000\u0000\u0000\u0000\u0000\u0000\u0000\u0000\u0000\u0000\u0000\u0000\u0000\u0000\u0000\u0000\u0000ÿÿ\u0000\u0000\u0000\u0000\u0000\u0000", "PMU.112\u0000\u0000\u0000\u0000\u0000\u0000\u0000\u0000\u0000\u0000p\u0000\u000f\u0000\u0006\u0000\u0003\u0000\u0001PZR.AI          PZR.BV          PZR.CI          PZR.AV          PZR.BI          PZR.CV          ANA1            ANA2            ANA3            DIG.stat1_01    DIG.stat1_02    DIG.stat1_03    DIG.stat1_04    DIG.stat1_05    DIG.stat1_06    DIG.stat1_07    DIG.stat1_08    DIG.stat1_09    DIG.stat1_10    DIG.stat1_11    DIG.stat1_12    DIG.stat1_13    DIG.stat1_14    DIG.stat1_15    DIG.stat1_16    \u0001\u0000\u0000\u0000\u0000\u0000\u0000\u0000\u0001\u0000\u0000\u0000\u0000\u0000\u0000\u0000\u0001\u0000\u0000\u0000\u0000\u0000\u0000\u0000\u0000\u0000\u0000\u0000\u0000\u0000\u0000\u0000\u0000\u0000\u0000\u0000ÿÿ\u0000\u0000\u0000\u0000\u0000\u0000", "PMU.113\u0000\u0000\u0000\u0000\u0000\u0000\u0000\u0000\u0000\u0000q\u0000\u000f\u0000\u0006\u0000\u0003\u0000\u0001PZR.AI          PZR.BV          PZR.CI          PZR.AV          PZR.BI          PZR.CV          ANA1            ANA2            ANA3            DIG.stat1_01    DIG.stat1_02    DIG.stat1_03    DIG.stat1_04    DIG.stat1_05    DIG.stat1_06    DIG.stat1_07    DIG.stat1_08    DIG.stat1_09    DIG.stat1_10    DIG.stat1_11    DIG.stat1_12    DIG.stat1_13    DIG.stat1_14    DIG.stat1_15    DIG.stat1_16    \u0001\u0000\u0000\u0000\u0000\u0000\u0000\u0000\u0001\u0000\u0000\u0000\u0000\u0000\u0000\u0000\u0001\u0000\u0000\u0000\u0000\u0000\u0000\u0000\u0000\u0000\u0000\u0000\u0000\u0000\u0000\u0000\u0000\u0000\u0000\u0000ÿÿ\u0000\u0000\u0000\u0000\u0000\u0000", "PMU.114\u0000\u0000\u0000\u0000\u0000\u0000\u0000\u0000\u0000\u0000r\u0000\u000f\u0000\u0006\u0000\u0003\u0000\u0001PZR.AI          PZR.BV          PZR.CI          PZR.AV          PZR.BI          PZR.CV          ANA1            ANA2            ANA3            DIG.stat1_01    DIG.stat1_02    DIG.stat1_03    DIG.stat1_04    DIG.stat1_05    DIG.stat1_06    DIG.stat1_07    DIG.stat1_08    DIG.stat1_09    DIG.stat1_10    DIG.stat1_11    DIG.stat1_12    DIG.stat1_13    DIG.stat1_14    DIG.stat1_15    DIG.stat1_16    \u0001\u0000\u0000\u0000\u0000\u0000\u0000\u0000\u0001\u0000\u0000\u0000\u0000\u0000\u0000\u0000\u0001\u0000\u0000\u0000\u0000\u0000\u0000\u0000\u0000\u0000\u0000\u0000\u0000\u0000\u0000\u0000\u0000\u0000\u0000\u0000ÿÿ\u0000\u0000\u0000\u0000\u0000\u0000", "PMU.115\u0000\u0000\u0000\u0000\u0000\u0000\u0000\u0000\u0000\u0000s\u0000\u000f\u0000\u0006\u0000\u0003\u0000\u0001PZR.AI          PZR.BV          PZR.CI          PZR.AV          PZR.BI          PZR.CV          ANA1            ANA2            ANA3            DIG.stat1_01    DIG.stat1_02    DIG.stat1_03    DIG.stat1_04    DIG.stat1_05    DIG.stat1_06    DIG.stat1_07    DIG.stat1_08    DIG.stat1_09    DIG.stat1_10    DIG.stat1_11    DIG.stat1_12    DIG.stat1_13    DIG.stat1_14    DIG.stat1_15    DIG.stat1_16    \u0001\u0000\u0000\u0000\u0000\u0000\u0000\u0000\u0001\u0000\u0000\u0000\u0000\u0000\u0000\u0000\u0001\u0000\u0000\u0000\u0000\u0000\u0000\u0000\u0000\u0000\u0000\u0000\u0000\u0000\u0000\u0000\u0000\u0000\u0000\u0000ÿÿ\u0000\u0000\u0000\u0000\u0000\u0000", "PMU.116\u0000\u0000\u0000\u0000\u0000\u0000\u0000\u0000\u0000\u0000t\u0000\u000f\u0000\u0006\u0000\u0003\u0000\u0001PZR.AI          PZR.BV          PZR.CI          PZR.AV          PZR.BI          PZR.CV          ANA1            ANA2            ANA3            DIG.stat1_01    DIG.stat1_02    DIG.stat1_03    DIG.stat1_04    DIG.stat1_05    DIG.stat1_06    DIG.stat1_07    DIG.stat1_08    DIG.stat1_09    DIG.stat1_10    DIG.stat1_11    DIG.stat1_12    DIG.stat1_13    DIG.stat1_14    DIG.stat1_15    DIG.stat1_16    \u0001\u0000\u0000\u0000\u0000\u0000\u0000\u0000\u0001\u0000\u0000\u0000\u0000\u0000\u0000\u0000\u0001\u0000\u0000\u0000\u0000\u0000\u0000\u0000\u0000\u0000\u0000\u0000\u0000\u0000\u0000\u0000\u0000\u0000\u0000\u0000ÿÿ\u0000\u0000\u0000\u0000\u0000\u0000", "PMU.117\u0000\u0000\u0000\u0000\u0000\u0000\u0000\u0000\u0000\u0000u\u0000\u000f\u0000\u0006\u0000\u0003\u0000\u0001PZR.AI          PZR.BV          PZR.CI          PZR.AV          PZR.BI          PZR.CV          ANA1            ANA2            ANA3            DIG.stat1_01    DIG.stat1_02    DIG.stat1_03    DIG.stat1_04    DIG.stat1_05    DIG.stat1_06    DIG.stat1_07    DIG.stat1_08    DIG.stat1_09    DIG.stat1_10    DIG.stat1_11    DIG.stat1_12    DIG.stat1_13    DIG.stat1_14    DIG.stat1_15    DIG.stat1_16    \u0001\u0000\u0000\u0000\u0000\u0000\u0000\u0000\u0001\u0000\u0000\u0000\u0000\u0000\u0000\u0000\u0001\u0000\u0000\u0000\u0000\u0000\u0000\u0000\u0000\u0000\u0000\u0000\u0000\u0000\u0000\u0000\u0000\u0000\u0000\u0000ÿÿ\u0000\u0000\u0000\u0000\u0000\u0000", "PMU.118\u0000\u0000\u0000\u0000\u0000\u0000\u0000\u0000\u0000\u0000v\u0000\u000f\u0000\u0006\u0000\u0003\u0000\u0001PZR.AI          PZR.BV          PZR.CI          PZR.AV          PZR.BI          PZR.CV          ANA1            ANA2            ANA3            DIG.stat1_01    DIG.stat1_02    DIG.stat1_03    DIG.stat1_04    DIG.stat1_05    DIG.stat1_06    DIG.stat1_07    DIG.stat1_08    DIG.stat1_09    DIG.stat1_10    DIG.stat1_11    DIG.stat1_12    DIG.stat1_13    DIG.stat1_14    DIG.stat1_15    DIG.stat1_16    \u0001\u0000\u0000\u0000\u0000\u0000\u0000\u0000\u0001\u0000\u0000\u0000\u0000\u0000\u0000\u0000\u0001\u0000\u0000\u0000\u0000\u0000\u0000\u0000\u0000\u0000\u0000\u0000\u0000\u0000\u0000\u0000\u0000\u0000\u0000\u0000ÿÿ\u0000\u0000\u0000\u0000\u0000\u0000", "PMU.119\u0000\u0000\u0000\u0000\u0000\u0000\u0000\u0000\u0000\u0000w\u0000\u000f\u0000\u0006\u0000\u0003\u0000\u0001PZR.AI          PZR.BV          PZR.CI          PZR.AV          PZR.BI          PZR.CV          ANA1            ANA2            ANA3            DIG.stat1_01    DIG.stat1_02    DIG.stat1_03    DIG.stat1_04    DIG.stat1_05    DIG.stat1_06    DIG.stat1_07    DIG.stat1_08    DIG.stat1_09    DIG.stat1_10    DIG.stat1_11    DIG.stat1_12    DIG.stat1_13    DIG.stat1_14    DIG.stat1_15    DIG.stat1_16    \u0001\u0000\u0000\u0000\u0000\u0000\u0000\u0000\u0001\u0000\u0000\u0000\u0000\u0000\u0000\u0000\u0001\u0000\u0000\u0000\u0000\u0000\u0000\u0000\u0000\u0000\u0000\u0000\u0000\u0000\u0000\u0000\u0000\u0000\u0000\u0000ÿÿ\u0000\u0000\u0000\u0000\u0000\u0000", "PMU.120\u0000\u0000\u0000\u0000\u0000\u0000\u0000\u0000\u0000\u0000x\u0000\u000f\u0000\u0006\u0000\u0003\u0000\u0001PZR.AI          PZR.BV          PZR.CI          PZR.AV          PZR.BI          PZR.CV          ANA1            ANA2            ANA3            DIG.stat1_01    DIG.stat1_02    DIG.stat1_03    DIG.stat1_04    DIG.stat1_05    DIG.stat1_06    DIG.stat1_07    DIG.stat1_08    DIG.stat1_09    DIG.stat1_10    DIG.stat1_11    DIG.stat1_12    DIG.stat1_13    DIG.stat1_14    DIG.stat1_15    DIG.stat1_16    \u0001\u0000\u0000\u0000\u0000\u0000\u0000\u0000\u0001\u0000\u0000\u0000\u0000\u0000\u0000\u0000\u0001\u0000\u0000\u0000\u0000\u0000\u0000\u0000\u0000\u0000\u0000\u0000\u0000\u0000\u0000\u0000\u0000\u0000\u0000\u0000ÿÿ\u0000\u0000\u0000\u0000\u0000\u0000", "PMU.121\u0000\u0000\u0000\u0000\u0000\u0000\u0000\u0000\u0000\u0000y\u0000\u000f\u0000\u0006\u0000\u0003\u0000\u0001PZR.AI          PZR.BV          PZR.CI          PZR.AV          PZR.BI          PZR.CV          ANA1            ANA2            ANA3            DIG.stat1_01    DIG.stat1_02    DIG.stat1_03    DIG.stat1_04    DIG.stat1_05    DIG.stat1_06    DIG.stat1_07    DIG.stat1_08    DIG.stat1_09    DIG.stat1_10    DIG.stat1_11    DIG.stat1_12    DIG.stat1_13    DIG.stat1_14    DIG.stat1_15    DIG.stat1_16    \u0001\u0000\u0000\u0000\u0000\u0000\u0000\u0000\u0001\u0000\u0000\u0000\u0000\u0000\u0000\u0000\u0001\u0000\u0000\u0000\u0000\u0000\u0000\u0000\u0000\u0000\u0000\u0000\u0000\u0000\u0000\u0000\u0000\u0000\u0000\u0000ÿÿ\u0000\u0000\u0000\u0000\u0000\u0000", "PMU.122\u0000\u0000\u0000\u0000\u0000\u0000\u0000\u0000\u0000\u0000z\u0000\u000f\u0000\u0006\u0000\u0003\u0000\u0001PZR.AI          PZR.BV          PZR.CI          PZR.AV          PZR.BI          PZR.CV          ANA1            ANA2            ANA3            DIG.stat1_01    DIG.stat1_02    DIG.stat1_03    DIG.stat1_04    DIG.stat1_05    DIG.stat1_06    DIG.stat1_07    DIG.stat1_08    DIG.stat1_09    DIG.stat1_10    DIG.stat1_11    DIG.stat1_12    DIG.stat1_13    DIG.stat1_14    DIG.stat1_15    DIG.stat1_16    \u0001\u0000\u0000\u0000\u0000\u0000\u0000\u0000\u0001\u0000\u0000\u0000\u0000\u0000\u0000\u0000\u0001\u0000\u0000\u0000\u0000\u0000\u0000\u0000\u0000\u0000\u0000\u0000\u0000\u0000\u0000\u0000\u0000\u0000\u0000\u0000ÿÿ\u0000\u0000\u0000\u0000\u0000\u0000", "PMU.123\u0000\u0000\u0000\u0000\u0000\u0000\u0000\u0000\u0000\u0000{\u0000\u000f\u0000\u0006\u0000\u0003\u0000\u0001PZR.AI          PZR.BV          PZR.CI          PZR.AV          PZR.BI          PZR.CV          ANA1            ANA2            ANA3            DIG.stat1_01    DIG.stat1_02    DIG.stat1_03    DIG.stat1_04    DIG.stat1_05    DIG.stat1_06    DIG.stat1_07    DIG.stat1_08    DIG.stat1_09    DIG.stat1_10    DIG.stat1_11    DIG.stat1_12    DIG.stat1_13    DIG.stat1_14    DIG.stat1_15    DIG.stat1_16    \u0001\u0000\u0000\u0000\u0000\u0000\u0000\u0000\u0001\u0000\u0000\u0000\u0000\u0000\u0000\u0000\u0001\u0000\u0000\u0000\u0000\u0000\u0000\u0000\u0000\u0000\u0000\u0000\u0000\u0000\u0000\u0000\u0000\u0000\u0000\u0000ÿÿ\u0000\u0000\u0000\u0000\u0000\u0000", "PMU.124\u0000\u0000\u0000\u0000\u0000\u0000\u0000\u0000\u0000\u0000|\u0000\u000f\u0000\u0006\u0000\u0003\u0000\u0001PZR.AI          PZR.BV          PZR.CI          PZR.AV          PZR.BI          PZR.CV          ANA1            ANA2            ANA3            DIG.stat1_01    DIG.stat1_02    DIG.stat1_03    DIG.stat1_04    DIG.stat1_05    DIG.stat1_06    DIG.stat1_07    DIG.stat1_08    DIG.stat1_09    DIG.stat1_10    DIG.stat1_11    DIG.stat1_12    DIG.stat1_13    DIG.stat1_14    DIG.stat1_15    DIG.stat1_16    \u0001\u0000\u0000\u0000\u0000\u0000\u0000\u0000\u0001\u0000\u0000\u0000\u0000\u0000\u0000\u0000\u0001\u0000\u0000\u0000\u0000\u0000\u0000\u0000\u0000\u0000\u0000\u0000\u0000\u0000\u0000\u0000\u0000\u0000\u0000\u0000ÿÿ\u0000\u0000\u0000\u0000\u0000\u0000", "PMU.125\u0000\u0000\u0000\u0000\u0000\u0000\u0000\u0000\u0000\u0000}\u0000\u000f\u0000\u0006\u0000\u0003\u0000\u0001PZR.AI          PZR.BV          PZR.CI          PZR.AV          PZR.BI          PZR.CV          ANA1            ANA2            ANA3            DIG.stat1_01    DIG.stat1_02    DIG.stat1_03    DIG.stat1_04    DIG.stat1_05    DIG.stat1_06    DIG.stat1_07    DIG.stat1_08    DIG.stat1_09    DIG.stat1_10    DIG.stat1_11    DIG.stat1_12    DIG.stat1_13    DIG.stat1_14    DIG.stat1_15    DIG.stat1_16    \u0001\u0000\u0000\u0000\u0000\u0000\u0000\u0000\u0001\u0000\u0000\u0000\u0000\u0000\u0000\u0000\u0001\u0000\u0000\u0000\u0000\u0000\u0000\u0000\u0000\u0000\u0000\u0000\u0000\u0000\u0000\u0000\u0000\u0000\u0000\u0000ÿÿ\u0000\u0000\u0000\u0000\u0000\u0000", "PMU.126\u0000\u0000\u0000\u0000\u0000\u0000\u0000\u0000\u0000\u0000~\u0000\u000f\u0000\u0006\u0000\u0003\u0000\u0001PZR.AI          PZR.BV          PZR.CI          PZR.AV          PZR.BI          PZR.CV          ANA1            ANA2            ANA3            DIG.stat1_01    DIG.stat1_02    DIG.stat1_03    DIG.stat1_04    DIG.stat1_05    DIG.stat1_06    DIG.stat1_07    DIG.stat1_08    DIG.stat1_09    DIG.stat1_10    DIG.stat1_11    DIG.stat1_12    DIG.stat1_13    DIG.stat1_14    DIG.stat1_15    DIG.stat1_16    \u0001\u0000\u0000\u0000\u0000\u0000\u0000\u0000\u0001\u0000\u0000\u0000\u0000\u0000\u0000\u0000\u0001\u0000\u0000\u0000\u0000\u0000\u0000\u0000\u0000\u0000\u0000\u0000\u0000\u0000\u0000\u0000\u0000\u0000\u0000\u0000ÿÿ\u0000\u0000\u0000\u0000\u0000\u0000", "PMU.127\u0000\u0000\u0000\u0000\u0000\u0000\u0000\u0000\u0000\u0000\u0000\u000f\u0000\u0006\u0000\u0003\u0000\u0001PZR.AI          PZR.BV          PZR.CI          PZR.AV          PZR.BI          PZR.CV          ANA1            ANA2            ANA3            DIG.stat1_01    DIG.stat1_02    DIG.stat1_03    DIG.stat1_04    DIG.stat1_05    DIG.stat1_06    DIG.stat1_07    DIG.stat1_08    DIG.stat1_09    DIG.stat1_10    DIG.stat1_11    DIG.stat1_12    DIG.stat1_13    DIG.stat1_14    DIG.stat1_15    DIG.stat1_16    \u0001\u0000\u0000\u0000\u0000\u0000\u0000\u0000\u0001\u0000\u0000\u0000\u0000\u0000\u0000\u0000\u0001\u0000\u0000\u0000\u0000\u0000\u0000\u0000\u0000\u0000\u0000\u0000\u0000\u0000\u0000\u0000\u0000\u0000\u0000\u0000ÿÿ\u0000\u0000\u0000\u0000\u0000\u0000", "PMU.128\u0000\u0000\u0000\u0000\u0000\u0000\u0000\u0000\u0000\u0000€\u0000\u000f\u0000\u0006\u0000\u0003\u0000\u0001PZR.AI          PZR.BV          PZR.CI          PZR.AV          PZR.BI          PZR.CV          ANA1            ANA2            ANA3            DIG.stat1_01    DIG.stat1_02    DIG.stat1_03    DIG.stat1_04    DIG.stat1_05    DIG.stat1_06    DIG.stat1_07    DIG.stat1_08    DIG.stat1_09    DIG.stat1_10    DIG.stat1_11    DIG.stat1_12    DIG.stat1_13    DIG.stat1_14    DIG.stat1_15    DIG.stat1_16    \u0001\u0000\u0000\u0000\u0000\u0000\u0000\u0000\u0001\u0000\u0000\u0000\u0000\u0000\u0000\u0000\u0001\u0000\u0000\u0000\u0000\u0000\u0000\u0000\u0000\u0000\u0000\u0000\u0000\u0000\u0000\u0000\u0000\u0000\u0000\u0000ÿÿ\u0000\u0000\u0000\u0000\u0000\u0000", "PMU.129\u0000\u0000\u0000\u0000\u0000\u0000\u0000\u0000\u0000\u0000\u0000\u000f\u0000\u0006\u0000\u0003\u0000\u0001PZR.AI          PZR.BV          PZR.CI          PZR.AV          PZR.BI          PZR.CV          ANA1            ANA2            ANA3            DIG.stat1_01    DIG.stat1_02    DIG.stat1_03    DIG.stat1_04    DIG.stat1_05    DIG.stat1_06    DIG.stat1_07    DIG.stat1_08    DIG.stat1_09    DIG.stat1_10    DIG.stat1_11    DIG.stat1_12    DIG.stat1_13    DIG.stat1_14    DIG.stat1_15    DIG.stat1_16    \u0001\u0000\u0000\u0000\u0000\u0000\u0000\u0000\u0001\u0000\u0000\u0000\u0000\u0000\u0000\u0000\u0001\u0000\u0000\u0000\u0000\u0000\u0000\u0000\u0000\u0000\u0000\u0000\u0000\u0000\u0000\u0000\u0000\u0000\u0000\u0000ÿÿ\u0000\u0000\u0000\u0000\u0000\u0000", "PMU.130\u0000\u0000\u0000\u0000\u0000\u0000\u0000\u0000\u0000\u0000‚\u0000\u000f\u0000\u0006\u0000\u0003\u0000\u0001PZR.AI          PZR.BV          PZR.CI          PZR.AV          PZR.BI          PZR.CV          ANA1            ANA2            ANA3            DIG.stat1_01    DIG.stat1_02    DIG.stat1_03    DIG.stat1_04    DIG.stat1_05    DIG.stat1_06    DIG.stat1_07    DIG.stat1_08    DIG.stat1_09    DIG.stat1_10    DIG.stat1_11    DIG.stat1_12    DIG.stat1_13    DIG.stat1_14    DIG.stat1_15    DIG.stat1_16    \u0001\u0000\u0000\u0000\u0000\u0000\u0000\u0000\u0001\u0000\u0000\u0000\u0000\u0000\u0000\u0000\u0001\u0000\u0000\u0000\u0000\u0000\u0000\u0000\u0000\u0000\u0000\u0000\u0000\u0000\u0000\u0000\u0000\u0000\u0000\u0000ÿÿ\u0000\u0000\u0000\u0000\u0000\u0000", "PMU.131\u0000\u0000\u0000\u0000\u0000\u0000\u0000\u0000\u0000\u0000ƒ\u0000\u000f\u0000\u0006\u0000\u0003\u0000\u0001PZR.AI          PZR.BV          PZR.CI          PZR.AV          PZR.BI          PZR.CV          ANA1            ANA2            ANA3            DIG.stat1_01    DIG.stat1_02    DIG.stat1_03    DIG.stat1_04    DIG.stat1_05    DIG.stat1_06    DIG.stat1_07    DIG.stat1_08    DIG.stat1_09    DIG.stat1_10    DIG.stat1_11    DIG.stat1_12    DIG.stat1_13    DIG.stat1_14    DIG.stat1_15    DIG.stat1_16    \u0001\u0000\u0000\u0000\u0000\u0000\u0000\u0000\u0001\u0000\u0000\u0000\u0000\u0000\u0000\u0000\u0001\u0000\u0000\u0000\u0000\u0000\u0000\u0000\u0000\u0000\u0000\u0000\u0000\u0000\u0000\u0000\u0000\u0000\u0000\u0000ÿÿ\u0000\u0000\u0000\u0000\u0000\u0000", "PMU.132\u0000\u0000\u0000\u0000\u0000\u0000\u0000\u0000\u0000\u0000„\u0000\u000f\u0000\u0006\u0000\u0003\u0000\u0001PZR.AI          PZR.BV          PZR.CI          PZR.AV          PZR.BI          PZR.CV          ANA1            ANA2            ANA3            DIG.stat1_01    DIG.stat1_02    DIG.stat1_03    DIG.stat1_04    DIG.stat1_05    DIG.stat1_06    DIG.stat1_07    DIG.stat1_08    DIG.stat1_09    DIG.stat1_10    DIG.stat1_11    DIG.stat1_12    DIG.stat1_13    DIG.stat1_14    DIG.stat1_15    DIG.stat1_16    \u0001\u0000\u0000\u0000\u0000\u0000\u0000\u0000\u0001\u0000\u0000\u0000\u0000\u0000\u0000\u0000\u0001\u0000\u0000\u0000\u0000\u0000\u0000\u0000\u0000\u0000\u0000\u0000\u0000\u0000\u0000\u0000\u0000\u0000\u0000\u0000ÿÿ\u0000\u0000\u0000\u0000\u0000\u0000", "PMU.133\u0000\u0000\u0000\u0000\u0000\u0000\u0000\u0000\u0000\u0000…\u0000\u000f\u0000\u0006\u0000\u0003\u0000\u0001PZR.AI          PZR.BV          PZR.CI          PZR.AV          PZR.BI          PZR.CV          ANA1            ANA2            ANA3            DIG.stat1_01    DIG.stat1_02    DIG.stat1_03    DIG.stat1_04    DIG.stat1_05    DIG.stat1_06    DIG.stat1_07    DIG.stat1_08    DIG.stat1_09    DIG.stat1_10    DIG.stat1_11    DIG.stat1_12    DIG.stat1_13    DIG.stat1_14    DIG.stat1_15    DIG.stat1_16    \u0001\u0000\u0000\u0000\u0000\u0000\u0000\u0000\u0001\u0000\u0000\u0000\u0000\u0000\u0000\u0000\u0001\u0000\u0000\u0000\u0000\u0000\u0000\u0000\u0000\u0000\u0000\u0000\u0000\u0000\u0000\u0000\u0000\u0000\u0000\u0000ÿÿ\u0000\u0000\u0000\u0000\u0000\u0000", "PMU.134\u0000\u0000\u0000\u0000\u0000\u0000\u0000\u0000\u0000\u0000†\u0000\u000f\u0000\u0006\u0000\u0003\u0000\u0001PZR.AI          PZR.BV          PZR.CI          PZR.AV          PZR.BI          PZR.CV          ANA1            ANA2            ANA3            DIG.stat1_01    DIG.stat1_02    DIG.stat1_03    DIG.stat1_04    DIG.stat1_05    DIG.stat1_06    DIG.stat1_07    DIG.stat1_08    DIG.stat1_09    DIG.stat1_10    DIG.stat1_11    DIG.stat1_12    DIG.stat1_13    DIG.stat1_14    DIG.stat1_15    DIG.stat1_16    \u0001\u0000\u0000\u0000\u0000\u0000\u0000\u0000\u0001\u0000\u0000\u0000\u0000\u0000\u0000\u0000\u0001\u0000\u0000\u0000\u0000\u0000\u0000\u0000\u0000\u0000\u0000\u0000\u0000\u0000\u0000\u0000\u0000\u0000\u0000\u0000ÿÿ\u0000\u0000\u0000\u0000\u0000\u0000", "PMU.135\u0000\u0000\u0000\u0000\u0000\u0000\u0000\u0000\u0000\u0000‡\u0000\u000f\u0000\u0006\u0000\u0003\u0000\u0001PZR.AI          PZR.BV          PZR.CI          PZR.AV          PZR.BI          PZR.CV          ANA1            ANA2            ANA3            DIG.stat1_01    DIG.stat1_02    DIG.stat1_03    DIG.stat1_04    DIG.stat1_05    DIG.stat1_06    DIG.stat1_07    DIG.stat1_08    DIG.stat1_09    DIG.stat1_10    DIG.stat1_11    DIG.stat1_12    DIG.stat1_13    DIG.stat1_14    DIG.stat1_15    DIG.stat1_16    \u0001\u0000\u0000\u0000\u0000\u0000\u0000\u0000\u0001\u0000\u0000\u0000\u0000\u0000\u0000\u0000\u0001\u0000\u0000\u0000\u0000\u0000\u0000\u0000\u0000\u0000\u0000\u0000\u0000\u0000\u0000\u0000\u0000\u0000\u0000\u0000ÿÿ\u0000\u0000\u0000\u0000\u0000\u0000", "PMU.136\u0000\u0000\u0000\u0000\u0000\u0000\u0000\u0000\u0000\u0000ˆ\u0000\u000f\u0000\u0006\u0000\u0003\u0000\u0001PZR.AI          PZR.BV          PZR.CI          PZR.AV          PZR.BI          PZR.CV          ANA1            ANA2            ANA3            DIG.stat1_01    DIG.stat1_02    DIG.stat1_03    DIG.stat1_04    DIG.stat1_05    DIG.stat1_06    DIG.stat1_07    DIG.stat1_08    DIG.stat1_09    DIG.stat1_10    DIG.stat1_11    DIG.stat1_12    DIG.stat1_13    DIG.stat1_14    DIG.stat1_15    DIG.stat1_16    \u0001\u0000\u0000\u0000\u0000\u0000\u0000\u0000\u0001\u0000\u0000\u0000\u0000\u0000\u0000\u0000\u0001\u0000\u0000\u0000\u0000\u0000\u0000\u0000\u0000\u0000\u0000\u0000\u0000\u0000\u0000\u0000\u0000\u0000\u0000\u0000ÿÿ\u0000\u0000\u0000\u0000\u0000\u0000", "PMU.137\u0000\u0000\u0000\u0000\u0000\u0000\u0000\u0000\u0000\u0000‰\u0000\u000f\u0000\u0006\u0000\u0003\u0000\u0001PZR.AI          PZR.BV          PZR.CI          PZR.AV          PZR.BI          PZR.CV          ANA1            ANA2            ANA3            DIG.stat1_01    DIG.stat1_02    DIG.stat1_03    DIG.stat1_04    DIG.stat1_05    DIG.stat1_06    DIG.stat1_07    DIG.stat1_08    DIG.stat1_09    DIG.stat1_10    DIG.stat1_11    DIG.stat1_12    DIG.stat1_13    DIG.stat1_14    DIG.stat1_15    DIG.stat1_16    \u0001\u0000\u0000\u0000\u0000\u0000\u0000\u0000\u0001\u0000\u0000\u0000\u0000\u0000\u0000\u0000\u0001\u0000\u0000\u0000\u0000\u0000\u0000\u0000\u0000\u0000\u0000\u0000\u0000\u0000\u0000\u0000\u0000\u0000\u0000\u0000ÿÿ\u0000\u0000\u0000\u0000\u0000\u0000", "PMU.138\u0000\u0000\u0000\u0000\u0000\u0000\u0000\u0000\u0000\u0000Š\u0000\u000f\u0000\u0006\u0000\u0003\u0000\u0001PZR.AI          PZR.BV          PZR.CI          PZR.AV          PZR.BI          PZR.CV          ANA1            ANA2            ANA3            DIG.stat1_01    DIG.stat1_02    DIG.stat1_03    DIG.stat1_04    DIG.stat1_05    DIG.stat1_06    DIG.stat1_07    DIG.stat1_08    DIG.stat1_09    DIG.stat1_10    DIG.stat1_11    DIG.stat1_12    DIG.stat1_13    DIG.stat1_14    DIG.stat1_15    DIG.stat1_16    \u0001\u0000\u0000\u0000\u0000\u0000\u0000\u0000\u0001\u0000\u0000\u0000\u0000\u0000\u0000\u0000\u0001\u0000\u0000\u0000\u0000\u0000\u0000\u0000\u0000\u0000\u0000\u0000\u0000\u0000\u0000\u0000\u0000\u0000\u0000\u0000ÿÿ\u0000\u0000\u0000\u0000\u0000\u0000", "PMU.139\u0000\u0000\u0000\u0000\u0000\u0000\u0000\u0000\u0000\u0000‹\u0000\u000f\u0000\u0006\u0000\u0003\u0000\u0001PZR.AI          PZR.BV          PZR.CI          PZR.AV          PZR.BI          PZR.CV          ANA1            ANA2            ANA3            DIG.stat1_01    DIG.stat1_02    DIG.stat1_03    DIG.stat1_04    DIG.stat1_05    DIG.stat1_06    DIG.stat1_07    DIG.stat1_08    DIG.stat1_09    DIG.stat1_10    DIG.stat1_11    DIG.stat1_12    DIG.stat1_13    DIG.stat1_14    DIG.stat1_15    DIG.stat1_16    \u0001\u0000\u0000\u0000\u0000\u0000\u0000\u0000\u0001\u0000\u0000\u0000\u0000\u0000\u0000\u0000\u0001\u0000\u0000\u0000\u0000\u0000\u0000\u0000\u0000\u0000\u0000\u0000\u0000\u0000\u0000\u0000\u0000\u0000\u0000\u0000ÿÿ\u0000\u0000\u0000\u0000\u0000\u0000"]}, "DATA Type"=w666, "CFG Type"=w665) -> (w664:cluster{"DATA Type":string, "CFG Type":string[]})
    n322 = local read "Stop Button"() -> (w674:bool)
    n323 = Enqueue Element(queue=w670, element=w664, error in (no error)=w667) -> (queue out=w669:refnum<queue>, error out=w668:errorcluster)  [unwired: 1 in, 1 out]
  }
  n324 = while {
    shift-right: [w683] -> _
    shift-left: string[] [] -> [w696]
    shift-right: [w691] -> _
    shift-left: u16[] [] -> [w692]
    shift-right: [w690] -> _
    shift-left: u16 0 -> [w694]
    shift-right: [w686] -> _
    shift-left: u16[] [] -> [w688]
    shift-right: [w684] -> _
    shift-left: u16[] [] -> [w685]
    stop <- w699 stop-if-true
    n325 = event shown="[0] \"PMU Phasors List 2\": Double Click" {
      selector: _ -> [_]
      dyn-events: _ -> [_]
      timeout: _ -> [_]
      event "PMU Phasors List 2": Double Click {
        n326 = event-data() -> ("Row"=→"PMU Row Number":i32)  [unwired: 1 in]
        n327 = local read "PMU1 CFG Packet"() -> (w701:string[])
        n328 = Index Array(array=w701, index="PMU Phasors List 2") -> (element=w707:string)
        n329 = call "PMU_INFO.vi"("data in"=w707) -> ("RET_DATA"=w711:T10)
        n330 = Unbundle By Name(w711) -> ("NUMs.PHNMR"=w710:u8, "Station Name"=w704:string)
        n331 = String Length(string=w707) -> (length=w708:i32)
        n332 = String Subset(string=w707, offset (0)=26, length (rest)=w708) -> (substring=w706:string)
        n333 = for {
          N: w710 -> [_]
          tunnel: w706 -> [w720]
          shift-right: [w716] -> _
          shift-left: 0 ("offset (0)") -> [w718]
          tunnel: w704 -> [w714]
          tunnel: [w712] -> w700 mode=indexing
          n334 = String Subset(string=w720, offset (0)=w718, length (rest)=16 ("length (rest)")) -> (substring=w713:string)
          n335 = Add(x=w718, y=16) -> (x+y=w716:i32)
          n336 = Concatenate Strings(w714, "/", w713) -> (w712:string)
        }
        n337 = property on="PMU Phasors List" class="LstBox (strict)"("Item Names"=w700) -> ()  [unwired: 2 in, 2 out]
      }
    }
    n338 = event shown="[0] \"PMU Phasors List\": Double Click" {
      selector: _ -> [_]
      dyn-events: _ -> [_]
      timeout: _ -> [_]
      tunnel: [w740] -> w695
      tunnel: w694 -> [w739]
      tunnel: [w738] -> w690
      tunnel: [w737] -> w687
      event "PMU Phasors List": Double Click {
        n339 = event-data() -> ("Row"=w737:i32)  [unwired: 1 in]
        "Phasor Row Number" <- w737
        n340 = Increment(x=w739) -> (x+1=w738:u16)
        n341 = property on="PMU Phasors List" class="LstBox (strict)"() -> ("Item Names"=w741:string[])  [unwired: 2 in, 2 out]
        n342 = Index Array(array=w741, index=w737) -> (element=w740:string)
      }
    }
    n343 = Equal?(x="", y=w695) -> (x = y?=w697:bool)
    n344 = Equal?(x=w690, y=u16 0) -> (x = y?=w689:bool)
    n345 = case shown="False" w689 {
      tunnel: w688 -> [w726 w728]
      tunnel: [w724 w728] -> w686
      tunnel: w687 -> [w725 _]
      tunnel: w685 -> [w723 w727]
      tunnel: [w722 w727] -> w684
      frame False {
        n346 = local read "PMU Row Number"() -> (w721:i32)
        n347 = Build Array (concatenate)(w723, w721) -> (w722:i32[])
        "PMU number in List" <- w722
        n348 = Build Array (concatenate)(w726, w725) -> (w724:i32[])
        "Phasor number in selected PMU" <- w724
      }
      frame True {
      }
    }
    n349 = case shown="True" w697 {
      tunnel: w696 -> [w733 w736]
      tunnel: [w735 w736] -> w683
      tunnel: w695 -> [w734 _]
      frame False {
        n350 = Build Array (concatenate)(w733, w734) -> (w735:string[])
      }
      frame True {
      }
    }
    "Phasor_Names" <- w683
    n351 = case shown="False" w689 {
      tunnel: w692 -> [w731 w732]
      tunnel: w690 -> [w730 _]
      tunnel: [w729 w732] -> w691
      frame False {
        n352 = Build Array (concatenate)(w731, w730) -> (w729:u16[])
        "Phasors Index" <- w729
      }
      frame True {
      }
    }
    n353 = property on="Chosen Data 2" class="LstBox (strict)"("Item Names"=w683) -> ()  [unwired: 2 in, 2 out]
    n354 = local read "Stop Button"() -> (w699:bool)
  }
  n355 = while {
    tunnel: w4 -> [w769]
    tunnel: w3 -> [w768]
    tunnel: w2 -> [w746]
    tunnel: w1 -> [w745]
    tunnel: [w743] -> _
    tunnel: [w742] -> _
    stop <- w770 stop-if-true
    # "Character Set"
    n356 = Dequeue Element(queue=w769, error in (no error)=w768) -> (element=w755:T7)  [unwired: 1 in, 3 out]
    n357 = property on="Phasor number in selected PMU" class="Arr (strict)"() -> ("Value"=w765:i32[])  [unwired: 2 in, 2 out]
    n358 = property on="PMU number in List" class="Arr (strict)"() -> ("Value"=w766:i32[])  [unwired: 2 in, 2 out]
    n359 = property on="Complex Phasors" class="Arr (strict)"() -> ("Value"=w764:csg[][])  [unwired: 2 in, 2 out]
    n360 = property on="Analog Values" class="Arr (strict)"() -> ("Value"=w763:sgl[][])  [unwired: 2 in, 2 out]
    n361 = property on="Frequency" class="Arr (strict)"() -> ("Value"=w762:sgl[])  [unwired: 2 in, 2 out]
    n362 = property on="dFreq" class="Arr (strict)"() -> ("Value"=w761:sgl[])  [unwired: 2 in, 2 out]
    n363 = Unbundle By Name(w755) -> ("Date/Time"=→"Date/Time 4":string)
    n364 = property on="Phasors Index" class="Arr (strict)"() -> ("Value"=w767:u16[])  [unwired: 2 in, 2 out]
    n365 = local read "Boolean array"() -> (w760:bool[][])
    n366 = call "DataChosen.vi"("Phasor Index"=w767, "Boolean array"=w760, "PMU Number in List"=w766, "Phasor  Number in List"=w765, "Complex Phasors"=w764, "Analog Values"=w763, "Frequency"=w762, "dFreq"=w761) -> ("Complex Phasors Output"=w758:csg[], "FREQ Values"=w757:dbl[], "DFREQ Values"=w756:dbl[])  [unwired: 5 in]
    "FREQ Values" <- w757
    "DFREQ Values" <- w756
    "Complex Phasors" <- w758
    n367 = Complex To Polar(r * e^(i*theta)=w758) -> (r=w753:sgl[], theta=w752:sgl[])
    "Angle" <- w752
    "Magnitude" <- w753
    n368 = property on="Phasor_Names" class="Arr (strict)"() -> ("Value"=w759:string[])  [unwired: 2 in, 2 out]
    n369 = for {
      tunnel: w759 -> [w785] mode=indexing
      tunnel: w758 -> [_] mode=indexing
      tunnel: w757 -> [w779] mode=indexing
      tunnel: w756 -> [w776] mode=indexing
      tunnel: w753 -> [w783] mode=indexing
      tunnel: w752 -> [w781] mode=indexing
      shift-right: [w771] -> _
      shift-left: "" ("string") -> [w772]
      tunnel: [w771] -> w749 mode=indexing
      w777 = ";" ("string")
      n370 = local read "Date/Time 4"() -> (w784:string)
      n371 = Number To Fractional String(number=w779) -> (F-format string=w778:string)  [unwired: 3 in]
      n372 = Number To Fractional String(number=w783) -> (F-format string=w782:string)  [unwired: 3 in]
      n373 = Number To Fractional String(number=w776) -> (F-format string=w775:string)  [unwired: 3 in]
      n374 = Number To Fractional String(number=w781) -> (F-format string=w780:string)  [unwired: 3 in]
      n375 = Concatenate Strings(w785, w777, w784, w777, w782, w777, w780, w777, w778, w777, w775) -> (w773:string)
      n376 = Concatenate Strings(w772, w773, "#" ("string")) -> (w771:string)
    }
    n377 = local read "Stop Button"() -> (w770:bool)
    n378 = property on="Phasors Index" class="Arr (strict)"() -> ("Value"=w748:u16[])  [unwired: 2 in, 2 out]
    n379 = Array Max & Min(array=w748) -> (max value=w747:u16)  [unwired: 3 out]
    n380 = Decrement(x=w747) -> (x-1=w750:u16)
    n381 = Index Array(array=w749, index=w750) -> (element=w744:string)
    "UDP STRNG 2" <- w744
    n382 = Enqueue Element(queue=w746, element=w744, error in (no error)=w745) -> (queue out=w743:refnum<queue>, error out=w742:errorcluster)  [unwired: 1 in, 1 out]
  }
  n383 = while {
    tunnel: w30 -> [w786]
    stop <- w816 stop-if-true
    # "UI Handling Loop"
    n384 = Index Array(array=w786, index="Names of PMUs") -> (element=w790:string)
    n385 = call "PMU_INFO.vi"("data in"=w790) -> ("RET_DATA"=w813:T10)
    n386 = local read "Stop Button"() -> (w816:bool)
    n387 = for {
      tunnel: w786 -> [w819] mode=indexing
      tunnel: [w817] -> w787 mode=concatenating
      n388 = String Subset(string=w819, offset (0)=0, length (rest)=16 ("length (rest)")) -> (substring=w818:string)
      n389 = String Length(string=w819) -> (length=w829:i32)
      n390 = String Subset(string=w819, offset (0)=20, length (rest)=2 ("length (rest)")) -> (substring=w827:string)
      n391 = Type Cast(type=u16 0, x=w827) -> (*(type *) &x=w823:u16)
      n392 = String Subset(string=w819, offset (0)=26, length (rest)=w829) -> (substring=w824:string)
      n393 = for {
        N: w823 -> [_]
        shift-right: [w835] -> _
        shift-left: 0 -> [w837]
        tunnel: w824 -> [w834]
        tunnel: w818 -> [w833]
        tunnel: [w831] -> w817 mode=indexing
        n394 = String Subset(string=w834, offset (0)=w837, length (rest)=16 ("length (rest)")) -> (substring=w832:string)
        n395 = Add(x=w837, y=16) -> (x+y=w835:i32)
        n396 = Concatenate Strings(w833, w832) -> (w831:string)
      }
    }
    "Available Phasors in the PMU/PDC Stream" <- w787
    n397 = Unbundle By Name(w813) -> ("NUMs.PHNMR"=→"No. of Phasors in this PMU":u8)
    n398 = Unbundle By Name(w813) -> ("NUMs.ANNMR"=→"No. of Analogs in this PMU":u8)
    n399 = Unbundle By Name(w813) -> ("NUMs.DGNMR"=w815:u8)
    n400 = Multiply(x=w815, y=u8 16) -> (x*y=→"No. of Digitals in this PMU":u8)
    n401 = local read "No. of Phasors in this PMU"() -> (w793:u8)
    n402 = String Length(string=w790) -> (length=w795:i32)
    n403 = local read "No. of Analogs in this PMU"() -> (w792:u8)
    n404 = String Subset(string=w790, offset (0)=26, length (rest)=w795) -> (substring=w806:string)
    n405 = local read "No. of Digitals in this PMU"() -> (w791:u8)
    n406 = String Length(string=w790) -> (length=w807:i32)
    n407 = Multiply(x=w793, y=u8 16) -> (x*y=w797:u8)
    n408 = String Length(string=w790) -> (length=w805:i32)
    n409 = Multiply(x=w792, y=u8 16) -> (x*y=w801:u8)
    n410 = String Subset(string=w806, offset (0)=w797, length (rest)=w805) -> (substring=w802:string)
    n411 = String Subset(string=w802, offset (0)=w801, length (rest)=w807) -> (substring=w803:string)
    n412 = for {
      N: w793 -> [_]
      tunnel: w806 -> [w856]
      tunnel: [w854] -> w788 mode=indexing
      shift-right: [w851] -> _
      shift-left: 0 ("offset (0)") -> [w853]
      n413 = String Subset(string=w856, offset (0)=w853, length (rest)=16 ("length (rest)")) -> (substring=w854:string)
      n414 = Add(x=w853, y=16) -> (x+y=w851:i32)
    }
    n415 = for {
      N: w792 -> [_]
      tunnel: w802 -> [w850]
      tunnel: [w848] -> w799 mode=indexing
      shift-right: [w845] -> _
      shift-left: 0 ("offset (0)") -> [w847]
      n416 = String Subset(string=w850, offset (0)=w847, length (rest)=16 ("length (rest)")) -> (substring=w848:string)
      n417 = Add(x=w847, y=16) -> (x+y=w845:i32)
    }
    n418 = for {
      N: w791 -> [_]
      tunnel: w803 -> [w844]
      tunnel: [w842] -> w804 mode=indexing
      shift-right: [w839] -> _
      shift-left: 0 ("offset (0)") -> [w841]
      n419 = String Subset(string=w844, offset (0)=w841, length (rest)=16 ("length (rest)")) -> (substring=w842:string)
      n420 = Add(x=w841, y=16) -> (x+y=w839:i32)
    }
    n421 = property on="PMU Analogs" class="LstBox (strict)"("Item Names"=w799) -> ()  [unwired: 2 in, 2 out]
    n422 = property on="PMU Digitals" class="LstBox (strict)"("Item Names"=w804) -> ()  [unwired: 2 in, 2 out]
    n423 = property on="PMU Phasors" class="LstBox (strict)"("Item Names"=w788) -> ()  [unwired: 2 in, 2 out]
    "PMU1 CFG Packet" <- w786
  }
  n424 = Flush Queue(queue=w36, error in (no error)=w35) -> ()  [unwired: 3 out]
